vi "数据编码.vi"(0 "table输入":string(combo), 5 "错误常量 2":errorcluster caption="错误输入", 9 "QN":string, 13 "MN":string, 14 "PW":string) -> (4 "错误常量":errorcluster caption="错误输出", 15 "通讯包字符串":string)   [LabVIEW 2016, in "数据传输系统.lvlib"]
panel:
  in  "时间戳 2":string
  out "核查数据发送次数":i32
  out "小时数据发送次数":i32
  out "长度":i32
  in  "数据块":T1
  out "通讯包":T2={"包头（2）"="##", "数据段长度（4）"="", "数据段"="", "CRC校验"="", "包尾"=""}
  # "范例代码：\n\n##0101QN=20160801085857223;ST=32;CN=1062;PW=100000;MN=010000A8900016F000169DC0;Flag=5\n;CP=&&RtdInterval=30&&1C80\\r\\n"
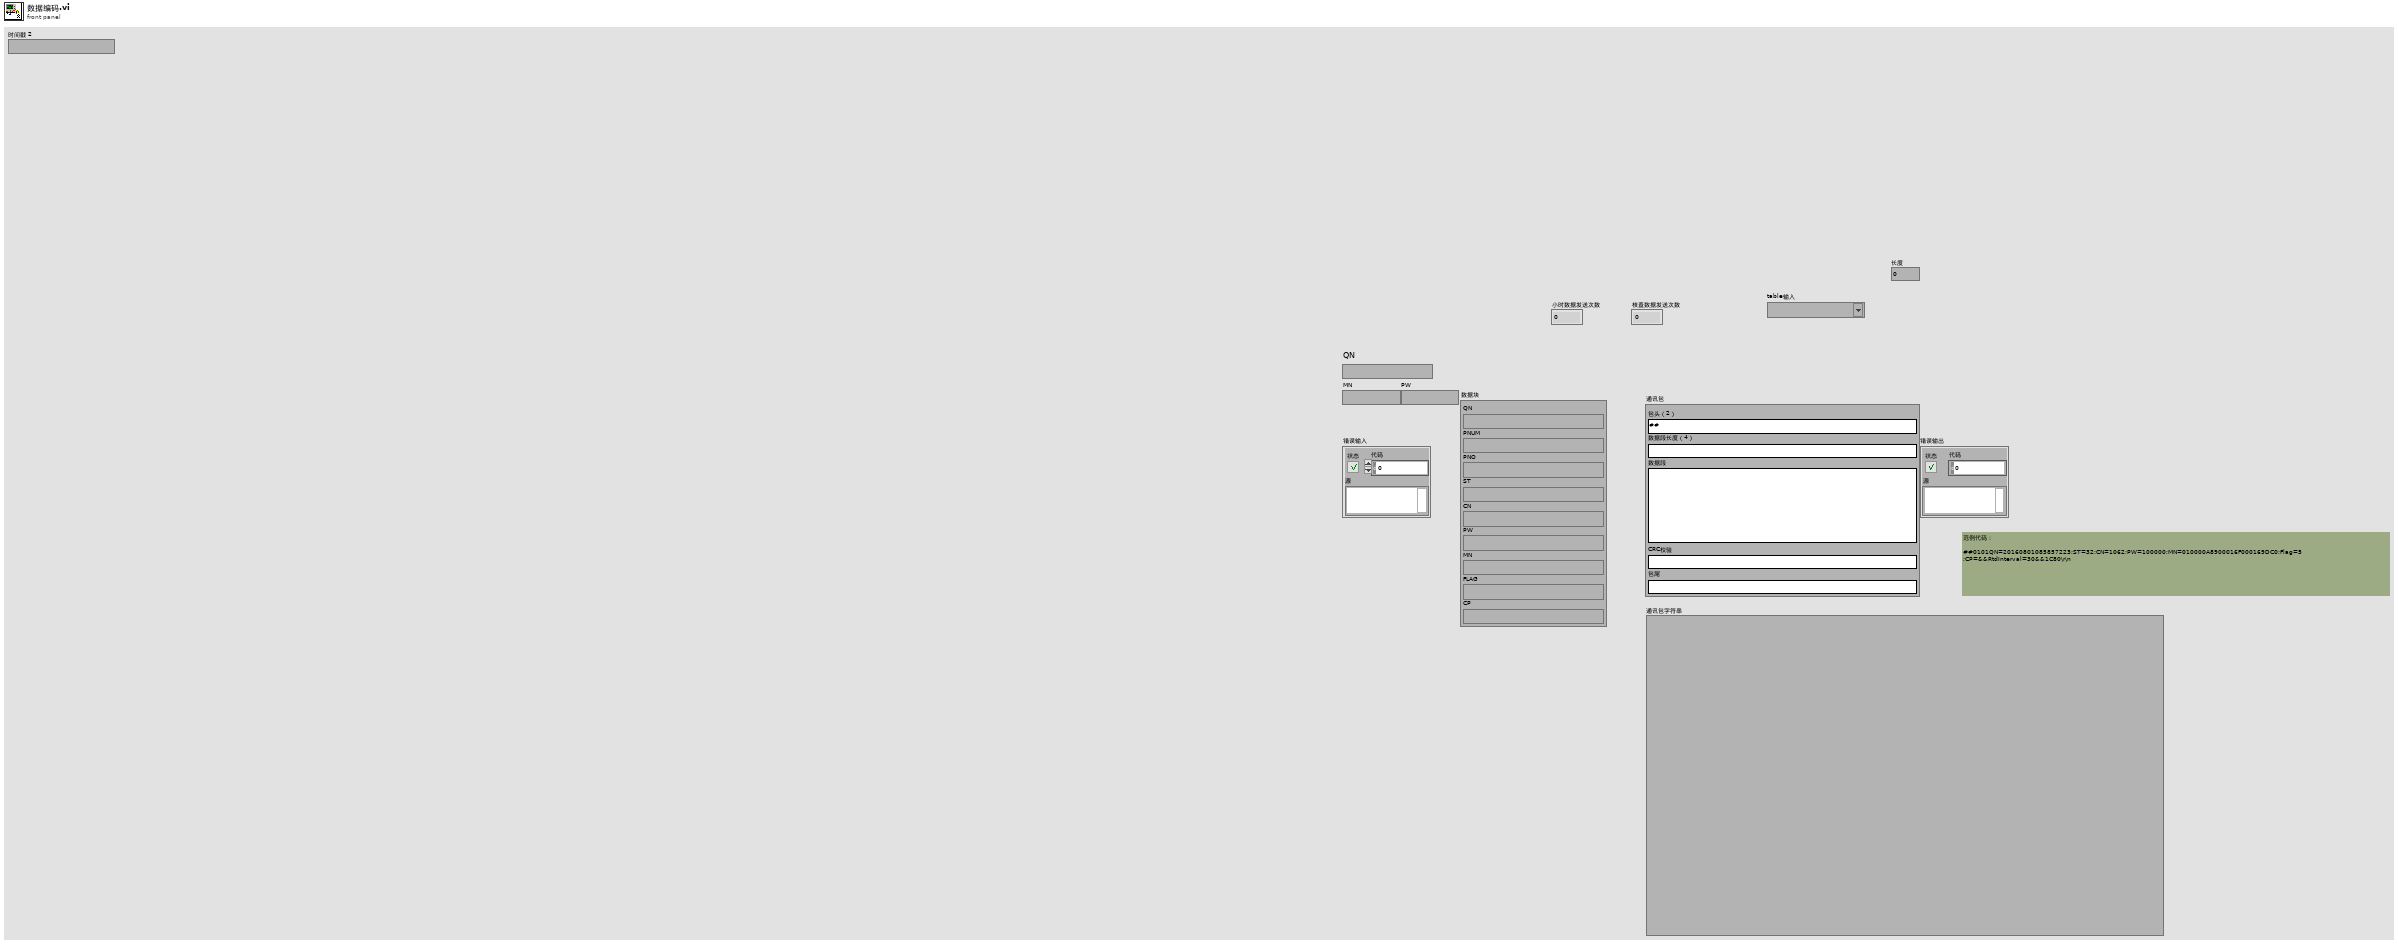
[diagram p1: front panel]
types:
  T1 = cluster{"QN":string, "ST":string, "CN":string, "PW":string, "MN":string, "FLAG":string, "PNUM":string, "PNO":string, "CP":string}
  T2 = cluster{"包头（2）":string, "数据段长度（4）":string, "数据段":string, "CRC校验":string, "包尾":string}
  T3 = cluster{"PH":string[][], "CODCr":string[][], "氨氮":string[][], "CODMn":string[][], "总氮":string[][], "总磷":string[][], "电导率":string[][], "水温":string[][], "DO":string[][], "浊度":string[][], "叶绿素":string[][], "藻密度":string[][], "铜":string[][], "盐度":string[][], "水位":string[][], "流速":string[][], "瞬时流量":string[][], "累积流量":string[][], "亚硝酸盐":string[][], "硫化物":string[][], "ORP":string[][], "铅":string[][], "镉":string[][], "锌":string[][], "镍":string[][], "锰":string[][], "汞":string[][]}
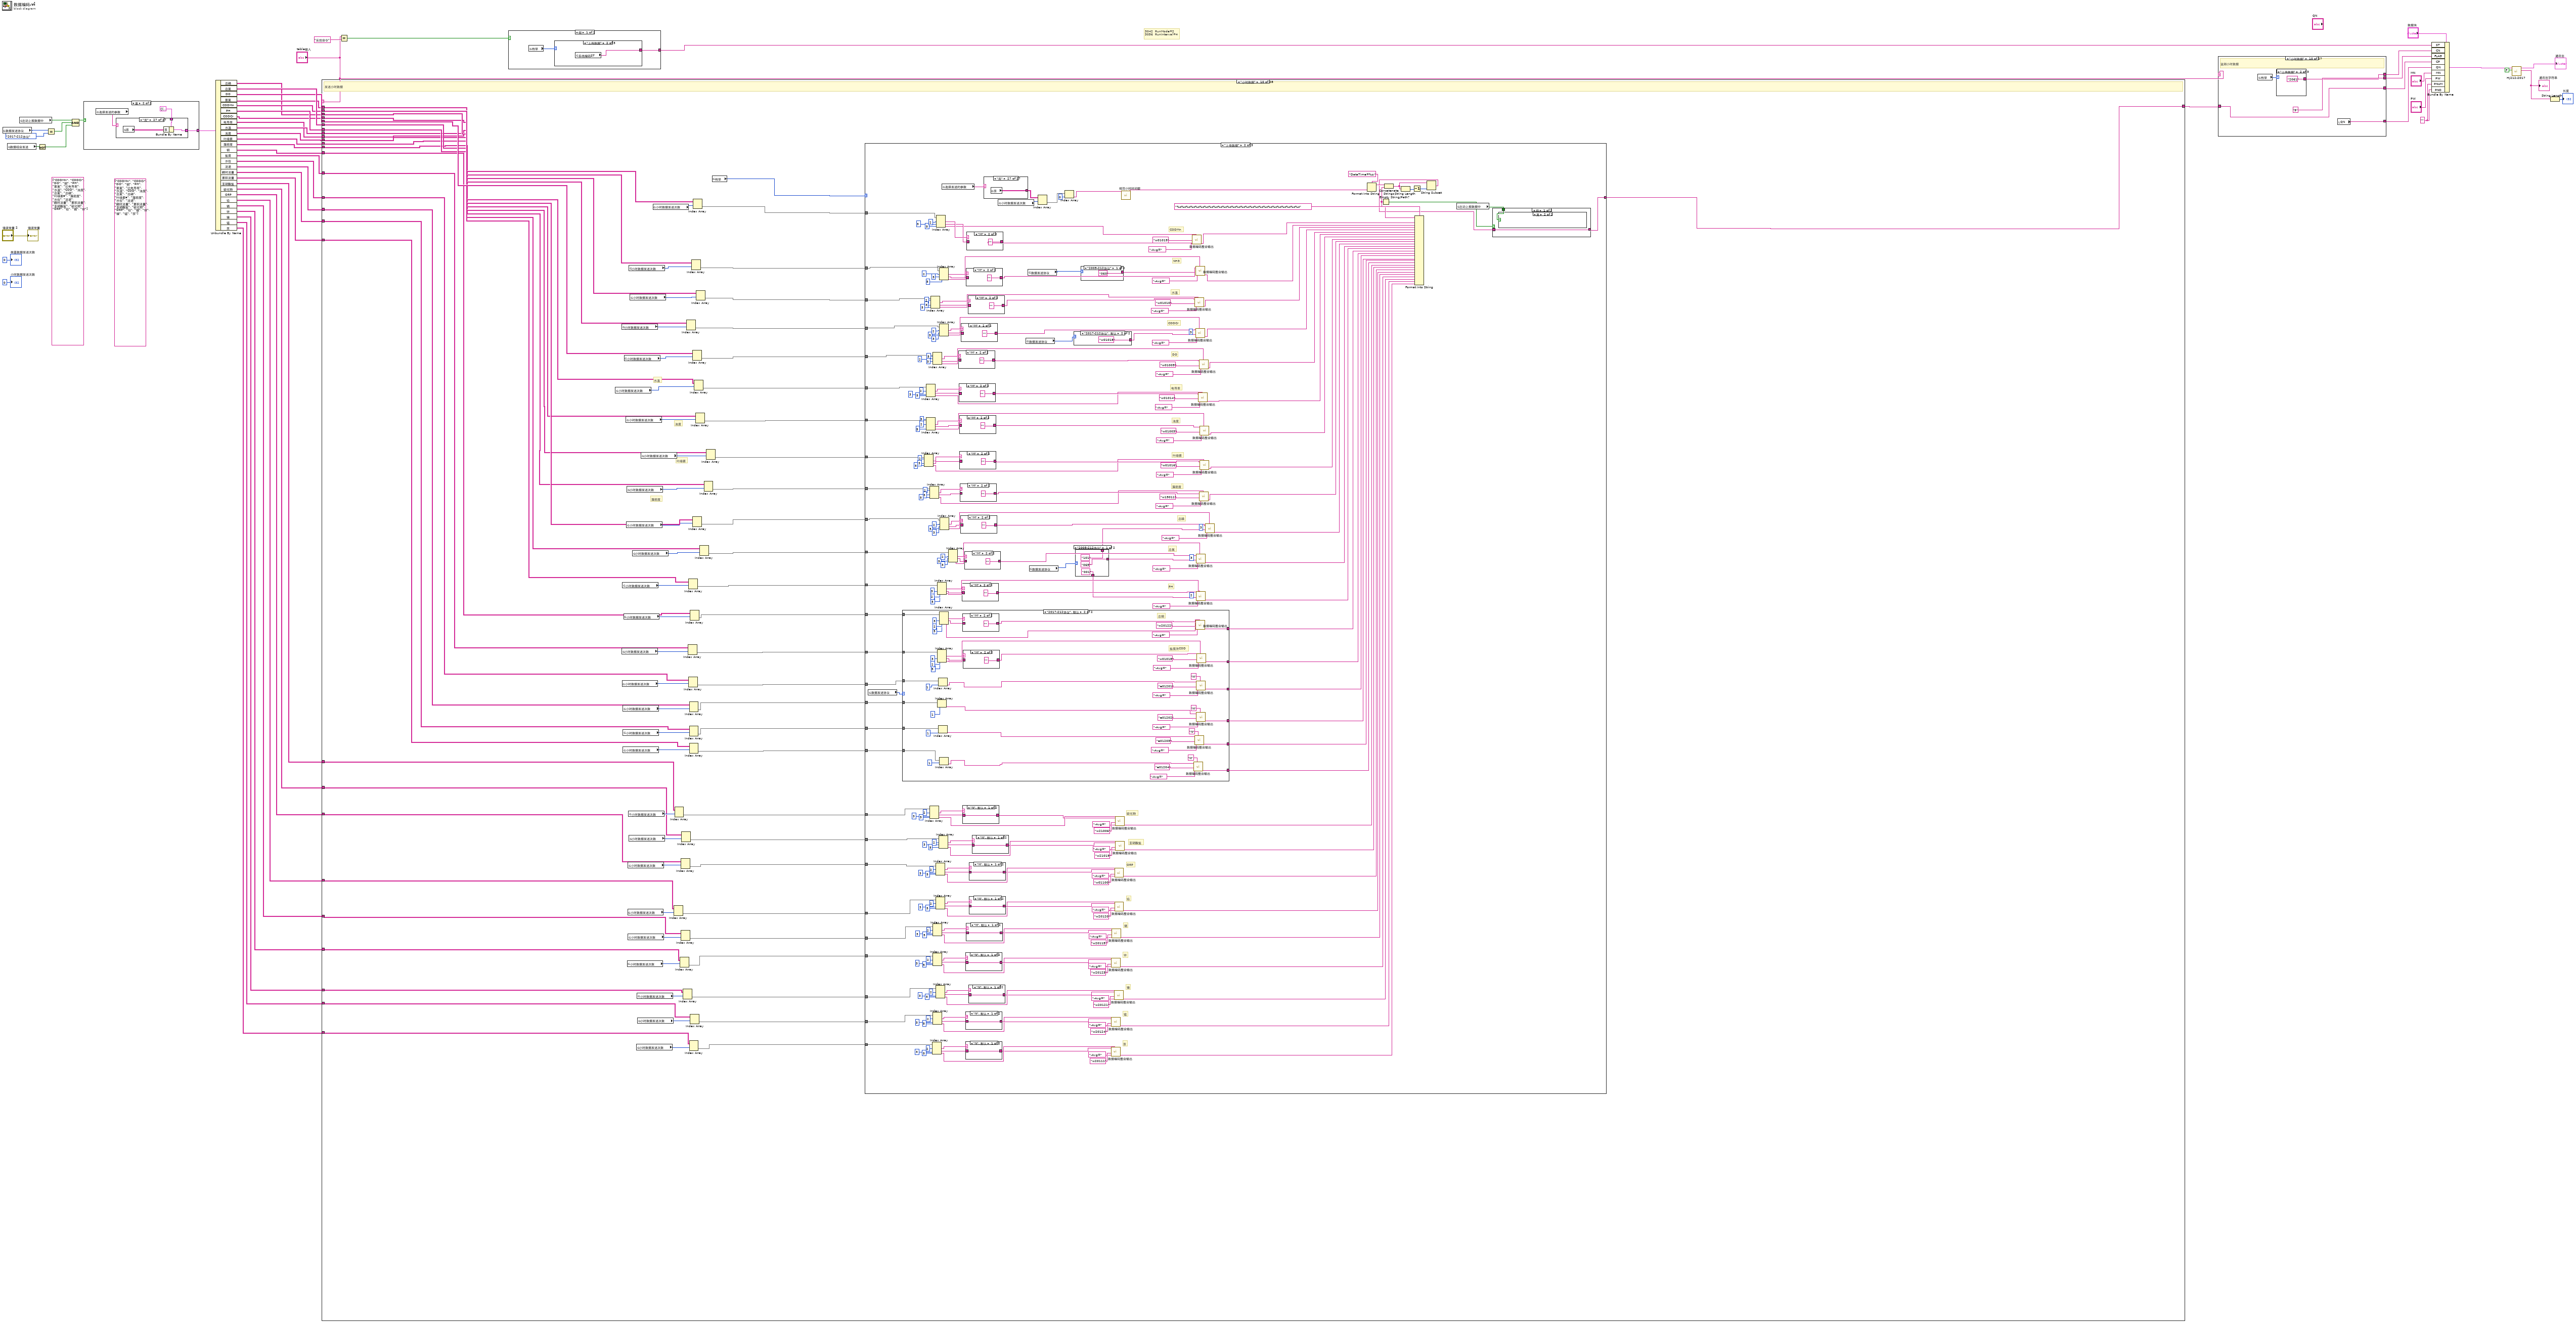
[diagram p0: block diagram]
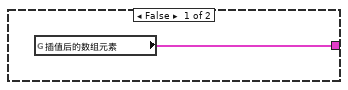
[diagram p2: hidden frame]
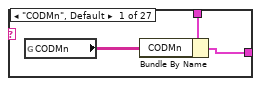
[diagram p3: hidden frame]
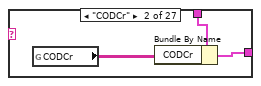
[diagram p4: hidden frame]
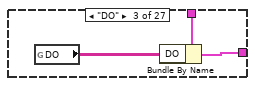
[diagram p5: hidden frame]
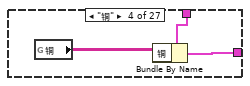
[diagram p6: hidden frame]
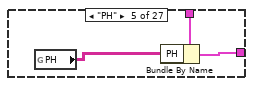
[diagram p7: hidden frame]
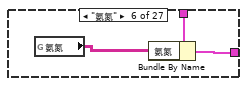
[diagram p8: hidden frame]
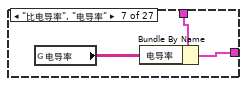
[diagram p9: hidden frame]
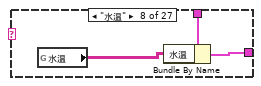
[diagram p10: hidden frame]
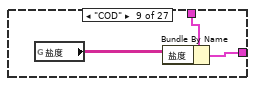
[diagram p11: hidden frame]
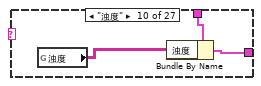
[diagram p12: hidden frame]
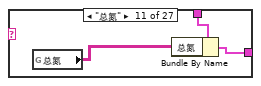
[diagram p13: hidden frame]
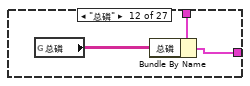
[diagram p14: hidden frame]
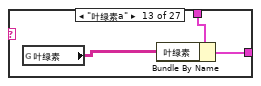
[diagram p15: hidden frame]
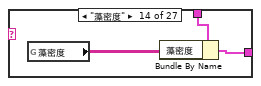
[diagram p16: hidden frame]
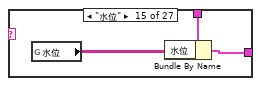
[diagram p17: hidden frame]
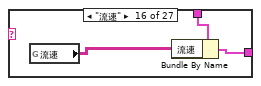
[diagram p18: hidden frame]
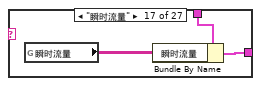
[diagram p19: hidden frame]
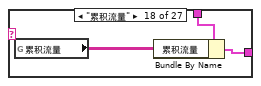
[diagram p20: hidden frame]
diagram:
  (unwired) string[] ["CODMn", "CODCr", "DO", "铜", "PH", "氨氮", "比电导率", "水温", "COD", "浊度", "总氮", "总磷", "叶绿素a", "藻密度", "水位", "流速", "瞬时流量", "累积流量", "亚硝酸盐", "硫化物", "ORP", "铅", "镉", "锌"] ("数组")
  (unwired) string[] ["CODMn", "CODCr", "DO", "铜", "PH", "氨氮", "比电导率", "水温", "COD", "浊度", "总氮", "总磷", "叶绿素a", "藻密度", "水位", "流速", "瞬时流量", "累积流量", "亚硝酸盐", "硫化物", "ORP", "铅", "镉", "锌", "镍", "锰", "汞"] ("数组")
  w40 = ""
  # "3042  RunMode=2\n3056  RunInterval=4"
  n1 = global read "断电保存全局.vi" "数据发送协议"() -> (w11:enum16{"2005-212协议", "2017-212协议"})
  n2 = global read "断电保存全局.vi" "数据组合发送"() -> (w13:bool)
  n3 = global read "全局 数据发送重叠.vi" "主动上报数据中"() -> (w26:bool)
  n4 = Not(x=w13) -> (.not. x?=w12:bool)
  n5 = Equal?(x=w11, y=enum16{"2005-212协议", "2017-212协议"}."2017-212协议" ("数据发送版本")) -> (x = y?=w16:bool)
  n6 = Compound Arithmetic op=AND ("复合运算")(w26, w16, w12) -> (w17:bool)
  n7 = case shown="真" w17 {
    tunnel: [w57 w59] -> w27
    frame False {
      n8 = global read "插值后的新数组.vi" "插值后的数组元素"() -> (w57:T3)
    }
    frame True {
      n9 = global read "全局 水样时间.vi" "选择发送的参数"() -> (w60:string)
      n10 = case shown="\"汞\"" w60 {
        tunnel: T3 {"PH"=[], "CODCr"=[], "氨氮"=[], "CODMn"=[], "总氮"=[], "总磷"=[], "电导率"=[], "水温"=[], "DO"=[], "浊度"=[], "叶绿素"=[], "藻密度"=[], "铜"=[], "盐度"=[], "水位"=[], "流速"=[], "瞬时流量"=[], "累积流量"=[], "亚硝酸盐"=[], "硫化物"=[], "ORP"=[], "铅"=[], "镉"=[], "锌"=[], "镍"=[], "锰"=[], "汞"=[]} ("插值后的数组元素") -> [w62 w66 w69 w72 w75 w78 w81 w84 w87 w90 w93 w96 w99 w101 w105 w108 w110 w113 w116 w119 w122 w125 w128 w131 w134 w137 w140]
        tunnel: [w61 w64 w67 w70 w73 w76 w80 w83 w85 w88 w91 w94 w97 w100 w103 w106 w109 w112 w115 w118 w121 w124 w127 w130 w133 w136 w139] -> w59
        frame "CODMn", Default {
          n11 = global read "全局 所有参数.vi" "CODMn"() -> (w63:string[][])
          n12 = Bundle By Name(cluster=w62, "CODMn"=w63) -> (w61:T3)
        }
        frame "CODCr" {
          n13 = global read "全局 所有参数.vi" "CODCr"() -> (w65:string[][])
          n14 = Bundle By Name(cluster=w66, "CODCr"=w65) -> (w64:T3)
        }
        frame "DO" {
          n15 = global read "全局 所有参数.vi" "DO"() -> (w68:string[][])
          n16 = Bundle By Name(cluster=w69, "DO"=w68) -> (w67:T3)
        }
        frame "铜" {
          n17 = global read "全局 所有参数.vi" "铜"() -> (w71:string[][])
          n18 = Bundle By Name(cluster=w72, "铜"=w71) -> (w70:T3)
        }
        frame "PH" {
          n19 = global read "全局 所有参数.vi" "PH"() -> (w74:string[][])
          n20 = Bundle By Name(cluster=w75, "PH"=w74) -> (w73:T3)
        }
        frame "氨氮" {
          n21 = global read "全局 所有参数.vi" "氨氮"() -> (w77:string[][])
          n22 = Bundle By Name(cluster=w78, "氨氮"=w77) -> (w76:T3)
        }
        frame "比电导率", "电导率" {
          n23 = global read "全局 所有参数.vi" "电导率"() -> (w79:string[][])
          n24 = Bundle By Name(cluster=w81, "电导率"=w79) -> (w80:T3)
        }
        frame "水温" {
          n25 = global read "全局 所有参数.vi" "水温"() -> (w82:string[][])
          n26 = Bundle By Name(cluster=w84, "水温"=w82) -> (w83:T3)
        }
        frame "COD" {
          n27 = global read "全局 所有参数.vi" "盐度"() -> (w86:string[][])
          n28 = Bundle By Name(cluster=w87, "盐度"=w86) -> (w85:T3)
        }
        frame "浊度" {
          n29 = global read "全局 所有参数.vi" "浊度"() -> (w89:string[][])
          n30 = Bundle By Name(cluster=w90, "浊度"=w89) -> (w88:T3)
        }
        frame "总氮" {
          n31 = global read "全局 所有参数.vi" "总氮"() -> (w92:string[][])
          n32 = Bundle By Name(cluster=w93, "总氮"=w92) -> (w91:T3)
        }
        frame "总磷" {
          n33 = global read "全局 所有参数.vi" "总磷"() -> (w95:string[][])
          n34 = Bundle By Name(cluster=w96, "总磷"=w95) -> (w94:T3)
        }
        frame "叶绿素a" {
          n35 = global read "全局 所有参数.vi" "叶绿素"() -> (w98:string[][])
          n36 = Bundle By Name(cluster=w99, "叶绿素"=w98) -> (w97:T3)
        }
        frame "藻密度" {
          n37 = global read "全局 所有参数.vi" "藻密度"() -> (w102:string[][])
          n38 = Bundle By Name(cluster=w101, "藻密度"=w102) -> (w100:T3)
        }
        frame "水位" {
          n39 = global read "全局 所有参数.vi" "水位"() -> (w104:string[][])
          n40 = Bundle By Name(cluster=w105, "水位"=w104) -> (w103:T3)
        }
        frame "流速" {
          n41 = global read "全局 所有参数.vi" "流速"() -> (w107:string[][])
          n42 = Bundle By Name(cluster=w108, "流速"=w107) -> (w106:T3)
        }
        frame "瞬时流量" {
          n43 = global read "全局 所有参数.vi" "瞬时流量"() -> (w111:string[][])
          n44 = Bundle By Name(cluster=w110, "瞬时流量"=w111) -> (w109:T3)
        }
        frame "累积流量" {
          n45 = global read "全局 所有参数.vi" "累积流量"() -> (w114:string[][])
          n46 = Bundle By Name(cluster=w113, "累积流量"=w114) -> (w112:T3)
        }
        frame "亚硝氮" {
          n47 = global read "全局 所有参数.vi" "亚硝酸盐"() -> (w117:string[][])
          n48 = Bundle By Name(cluster=w116, "亚硝酸盐"=w117) -> (w115:T3)
        }
        frame "硫化物" {
          n49 = global read "全局 所有参数.vi" "硫化物"() -> (w120:string[][])
          n50 = Bundle By Name(cluster=w119, "硫化物"=w120) -> (w118:T3)
        }
        frame "ORP" {
          n51 = global read "全局 所有参数.vi" "ORP"() -> (w123:string[][])
          n52 = Bundle By Name(cluster=w122, "ORP"=w123) -> (w121:T3)
        }
        frame "铅" {
          n53 = global read "全局 所有参数.vi" "铅"() -> (w126:string[][])
          n54 = Bundle By Name(cluster=w125, "铅"=w126) -> (w124:T3)
        }
        frame "镉" {
          n55 = global read "全局 所有参数.vi" "镉"() -> (w129:string[][])
          n56 = Bundle By Name(cluster=w128, "镉"=w129) -> (w127:T3)
        }
        frame "锌" {
          n57 = global read "全局 所有参数.vi" "锌"() -> (w132:string[][])
          n58 = Bundle By Name(cluster=w131, "锌"=w132) -> (w130:T3)
        }
        frame "镍" {
          n59 = global read "全局 所有参数.vi" "镍"() -> (w135:string[][])
          n60 = Bundle By Name(cluster=w134, "镍"=w135) -> (w133:T3)
        }
        frame "锰" {
          n61 = global read "全局 所有参数.vi" "锰"() -> (w138:string[][])
          n62 = Bundle By Name(cluster=w137, "锰"=w138) -> (w136:T3)
        }
        frame "汞" {
          n63 = global read "全局 所有参数.vi" "汞"() -> (w141:string[][])
          n64 = Bundle By Name(cluster=w140, "汞"=w141) -> (w139:T3)
        }
      }
    }
  }
  n65 = Unbundle By Name(w27) -> ("总磷"=w19:string[][], "总氮"=w24:string[][], "DO"=w23:string[][], "氨氮"=w22:string[][], "CODMn"=w20:string[][], "PH"=w39:string[][], "CODCr"=w21:string[][], "电导率"=w15:string[][], "水温"=w38:string[][], "浊度"=w14:string[][], "叶绿素"=w37:string[][], "藻密度"=w34:string[][], "铜"=w33:string[][], "盐度"=w32:string[][], "水位"=w31:string[][], "流速"=w30:string[][], "瞬时流量"=w29:string[][], "累积流量"=w28:string[][], "亚硝酸盐"=w10:string[][], "硫化物"=w9:string[][], "ORP"=w8:string[][], "铅"=w6:string[][], "镉"=w5:string[][], "锌"=w4:string[][], "镍"=w3:string[][], "锰"=w2:string[][], "汞"=w1:string[][])
  n66 = case shown="\"小时数据\"" "table输入" {
    tunnel: [w143 w150 w164 w207 w230 _ w244 w253 w289 w1334 w1759 w1806 w1895 w2046 w2218 w2451 w2518 w2564 w2612 w2684 w2812 w2926 w3040 w3133 w3587 w3623 w3634 w3645] -> w35
    tunnel: w20 -> [_ _ _ _ _ _ _ _ w287 w1333 _ _ w1894 w2058 w2222 w2455 w2522 w2563 w2611 w2683 w2811 w2925 w3039 w3132 _ _ _ _]
    tunnel: w22 -> [_ _ _ _ _ _ _ _ w286 w1332 _ _ w1893 w2057 w2221 w2454 w2523 w2562 w2610 w2682 w2810 w2924 w3038 w3131 _ _ _ _]
    tunnel: w23 -> [_ _ _ _ _ _ _ _ w283 w1331 _ _ w1892 w2056 w2200 _ _ _ w2606 w2681 w2809 w2923 w3037 w3111 _ _ _ _]
    tunnel: w19 -> [_ _ _ _ _ _ _ _ w278 w1330 _ _ w1891 w2055 w2220 w2453 w2521 w2561 w2607 w2680 w2808 w2922 w3036 w3130 _ _ _ _]
    tunnel: w24 -> [_ _ _ _ _ _ _ _ w277 w1329 _ _ w1890 w2054 w2219 w2452 w2520 w2559 w2609 w2679 w2807 w2921 w3035 w3129 _ _ _ _]
    tunnel: w39 -> [_ _ _ _ _ _ _ _ w284 w1328 _ _ w1889 w2053 w2204 _ _ _ w2605 _ w2791 w2905 w3013 w3109 _ _ _ _]
    tunnel: w21 -> [_ _ _ _ _ _ _ _ w270 w1327 _ _ w1888 w2052 w2217 w2450 w2519 w2560 w2608 w2666 w2795 w2909 w3023 w3116 _ _ _ _]
    tunnel: w15 -> [_ _ _ _ _ _ _ _ w282 w1326 _ _ w1887 w2051 w2197 _ _ _ w2603 _ w2788 w2902 w3011 w3106 _ _ _ _]
    tunnel: w38 -> [_ _ _ _ _ _ _ _ w285 w1325 _ _ w1886 w2050 _ _ _ _ w2604 _ w2785 w2899 w3012 w3101 _ _ _ _]
    tunnel: w14 -> [_ _ _ _ _ _ _ _ w281 w1324 _ _ w1885 w2049 w2194 _ _ _ w2602 _ w2779 w2893 w3007 w3100 _ _ _ _]
    tunnel: w37 -> [_ _ _ _ _ _ _ _ w280 w1323 _ _ w1884 w2048 _ _ _ _ _ _ w2777 w2891 w3005 w3099 _ _ _ _]
    tunnel: w34 -> [_ _ _ _ _ _ _ _ w279 w1322 _ _ w1883 w2047 _ _ _ _ _ _ w2775 w2889 w3004 w3114 _ _ _ _]
    tunnel: w33 -> [_ _ _ _ _ _ _ _ w276 w1292 _ _ w1853 w2018 _ _ _ _ _ _ _ _ _ _ _ _ _ _]
    tunnel: w32 -> [_ _ _ _ _ _ _ _ w275 w1291 _ _ w1852 w2017 _ _ _ _ _ _ _ _ _ _ _ _ _ _]
    tunnel: w31 -> [_ _ _ _ _ _ _ _ w273 w1282 _ _ _ _ _ _ _ _ _ _ _ _ _ _ _ _ _ _]
    tunnel: w30 -> [_ _ _ _ _ _ _ _ w274 w1281 _ _ _ _ _ _ _ _ _ _ _ _ _ _ _ _ _ _]
    tunnel: w29 -> [_ _ _ _ _ _ _ _ w272 w1280 _ _ _ _ _ _ _ _ _ _ _ _ _ _ _ _ _ _]
    tunnel: w28 -> [_ _ _ _ _ _ _ _ w271 w1279 _ _ _ _ _ _ _ _ _ _ _ _ _ _ _ _ _ _]
    tunnel: w10 -> [_ _ _ _ _ _ _ _ w269 w1275 _ _ _ _ _ _ _ _ _ _ _ _ _ _ _ _ _ _]
    tunnel: w9 -> [_ _ _ _ _ _ _ _ w268 w1274 _ _ _ _ _ _ _ _ _ _ _ _ _ _ _ _ _ _]
    tunnel: w8 -> [_ _ _ _ _ _ _ _ w267 w1273 _ _ _ _ _ _ _ _ _ _ w2773 w2887 w3003 _ _ _ _ _]
    tunnel: w6 -> [_ _ _ _ _ _ _ _ w266 w1266 _ _ _ _ _ _ _ _ _ _ _ _ _ _ _ _ _ _]
    tunnel: w5 -> [_ _ _ _ _ _ _ _ w265 w1265 _ _ _ _ _ _ _ _ _ _ _ _ _ _ _ _ _ _]
    tunnel: w4 -> [_ _ _ _ _ _ _ _ w264 w1264 _ _ _ _ _ _ _ _ _ _ _ _ _ _ _ _ _ _]
    tunnel: w3 -> [_ _ _ _ _ _ _ _ w263 w1257 _ _ _ _ _ _ _ _ _ _ _ _ _ _ _ _ _ _]
    tunnel: w2 -> [_ _ _ _ _ _ _ _ w262 w1256 _ _ _ _ _ _ _ _ _ _ _ _ _ _ _ _ _ _]
    tunnel: w1 -> [_ _ _ _ _ _ _ _ w261 w1255 _ _ _ _ _ _ _ _ _ _ _ _ _ _ _ _ _ _]
    frame "反控命令" {
      n67 = global read "全局 反控命令枚举.vi" "反控命令枚举"() -> (w142:enum16{"返回请求应答", "返回执行结果"})
      n68 = case shown="\"返回执行结果\"" w142 {
        tunnel: ["QnRtn=1" w146] -> w143
        frame "返回请求应答", Default {
        }
        frame "返回执行结果" {
          n69 = global read "全局 反控命令枚举.vi" "执行结果定义"() -> (w147:u16)
          n70 = Number To Decimal String(number=w147) -> (decimal integer string=w145:string)  [unwired: 1 in]
          n71 = Concatenate Strings("ExeRtn=", w145) -> (w146:string)
        }
      }
    }
    frame "超标留样返回" {
      n72 = global read "全局1.vi" "枚举"() -> (w149:enum16{"返回请求应答", "上传数据", "返回执行结果"})
      n73 = case shown="\"返回请求应答\", 默认" w149 {
        tunnel: ["QnRtn=1" w152 "ExeRtn=1"] -> w150
        frame "返回请求应答", Default {
        }
        frame "上传数据" {
          n74 = global read "全局1.vi" "register values"() -> (w161:u16[])
          n75 = Index Array(array=w161, index=7 ("索引")) -> (element=w154:u16)
          n76 = Get Date/Time In Seconds() -> (seconds since 1Jan1904=w159:timestamp)
          n77 = Number To Decimal String(number=w154) -> (decimal integer string=w155:string)  [unwired: 1 in]
          n78 = Format Date/Time String(time format string (%c)="%Y%m%d%H%M%S" ("时间格式字符串(%c)"), seconds (now)=w159) -> (date/time string=w157:string)  [unwired: 1 in]
          n79 = Format Into String(format string="VaseNo=%s" ("格式字符串"), w155) -> (resulting string=w153:string)  [unwired: 2 in, 1 out]
          n80 = Format Into String(format string="DataTime=%s;%s" ("格式字符串"), w157, w153) -> (resulting string=w152:string)  [unwired: 2 in, 1 out]
        }
        frame "返回执行结果" {
        }
      }
    }
    frame "提取经纬度环境信息" {
      # "BDS纬度"
      # "BDS纬度"
      # "GPS纬度"
      # "GPS经度"
      # "湿度"
      # "温度"
      # "电压"
      # "时间"
      n81 = global read "全局1.vi" "枚举"() -> (w165:enum16{"返回请求应答", "上传数据", "返回执行结果"})
      n82 = case shown="\"上传数据\"" w165 {
        tunnel: ["QnRtn=1" w178 "ExeRtn=1"] -> w164
        frame "返回请求应答", Default {
        }
        frame "上传数据" {
          n83 = global read "全局 环境参数.vi" "columns输出"() -> (w175:string[])
          n84 = Array Subset(array=w175, index=1 ("索引")) -> (w176:string[])  [unwired: 1 in]
          n85 = for {
            tunnel: w176 -> [w184] mode=indexing
            tunnel: [w183] -> w177 mode=indexing
            n86 = case shown="\"BDS经度\"" w184 {
              tunnel: ["" "Volt=%s;" "Temp=%s;" ("格式字符串") "Hum=%s;" ("格式字符串") "Lng=%s;" "Lat=%s;" "Lng2=%s;" "Lat2=%s;"] -> w183
              frame "假", Default {
              }
              frame "电压" {
              }
              frame "室温" {
              }
              frame "湿度" {
              }
              frame "GPS经度" {
              }
              frame "GPS纬度" {
              }
              frame "BDS经度" {
              }
              frame "BDS纬度" {
              }
            }
          }
          n87 = global read "全局 环境参数.vi" "环境参数"() -> (w168:string[][])
          n88 = Index Array(array=w168, index (row)=0 ("索引 (行)")) -> (element=w171:string[])  [unwired: 1 in]
          n89 = Array Subset(array=w171, index=1 ("索引")) -> (w173:string[])  [unwired: 1 in]
          n90 = for {
            shift-right: [w198] -> w167
            shift-left: "" -> [w197]
            tunnel: w177 -> [w196] mode=indexing
            tunnel: w173 -> [w194] mode=indexing
            n91 = Fract/Exp String To Number(string=w194) -> (number=w195:dbl)  [unwired: 3 in, 1 out]
            n92 = Empty String/Path?(string/path=w194) -> (empty?=w200:bool)
            n93 = Number To Fractional String(number=w195) -> (F-format string=w193:string)  [unwired: 3 in]
            n94 = case shown="假" w200 {
              tunnel: [w203 w204] -> w199
              tunnel: w196 -> [w202 _]
              tunnel: w193 -> [w201 _]
              tunnel: w193 -> [_ w204]
              frame False {
                n95 = Format Into String(format string=w202, w201) -> (resulting string=w203:string)  [unwired: 2 in, 1 out]
              }
              frame True {
              }
            }
            n96 = Concatenate Strings(w197, w199) -> (w198:string)
          }
          n97 = Get Date/Time In Seconds() -> (seconds since 1Jan1904=w180:timestamp)
          n98 = Format Date/Time String(time format string (%c)="%Y%m%d%H%M%S" ("时间格式字符串(%c)"), seconds (now)=w180) -> (date/time string=w179:string)  [unwired: 1 in]
          n99 = Format Into String(format string="DataTime=%s;%s" ("格式字符串"), w179, w167) -> (resulting string=w178:string)  [unwired: 2 in, 1 out]
        }
        frame "返回执行结果" {
        }
      }
    }
    frame "提取现场系统信息" {
      n100 = global read "全局1.vi" "枚举"() -> (w206:enum16{"返回请求应答", "上传数据", "返回执行结果"})
      n101 = case shown="\"上传数据\"" w206 {
        tunnel: ["QnRtn=1" w227 "ExeRtn=1"] -> w207
        frame "返回请求应答", Default {
        }
        frame "上传数据" {
          n102 = global read "全局1.vi" "register values"() -> (w226:u16[])
          n103 = Get Date/Time In Seconds() -> (seconds since 1Jan1904=w212:timestamp)
          n104 = Index Array(array=w226, index #1=0 ("索引"), index #2=6 ("索引")) -> (element #1=w222:u16, element #2=w209:u16)
          n105 = Format Date/Time String(time format string (%c)="%Y%m%d%H%M%S%u" ("时间格式字符串(%c)"), seconds (now)=w212) -> (date/time string=w215:string)  [unwired: 1 in]
          n106 = Number To Decimal String(number=w222) -> (decimal integer string=w224:string)  [unwired: 1 in]
          n107 = Number To Decimal String(number=w209) -> (decimal integer string=w218:string)  [unwired: 1 in]
          n108 = Search and Replace String(input string=w215, search string="." ("搜索字符串")) -> (result string=w211:string)  [unwired: 6 in, 3 out]
          n109 = Format Into String(format string="RunMode=%s;" ("格式字符串"), w224) -> (resulting string=w221:string)  [unwired: 2 in, 1 out]
          n110 = Format Into String(format string="RunInterval=%s;" ("格式字符串"), w218) -> (resulting string=w219:string)  [unwired: 2 in, 1 out]
          n111 = Format Into String(format string="SystemTime=%s;" ("格式字符串"), w211) -> (resulting string=w216:string)  [unwired: 2 in, 1 out]
          n112 = Concatenate Strings(w221, w219, w216) -> (w227:string)
        }
        frame "返回执行结果" {
        }
      }
    }
    frame "提取监测仪表时间" {
      n113 = global read "全局1.vi" "枚举"() -> (w229:enum16{"返回请求应答", "上传数据", "返回执行结果"})
      n114 = case shown="\"上传数据\"" w229 {
        tunnel: ["QnRtn=1" w242 "ExeRtn=1"] -> w230
        frame "返回请求应答", Default {
        }
        frame "上传数据" {
          n115 = global read "全局 提取仪器参数.vi" "仪器编码"() -> (w232:string)
          n116 = Get Date/Time In Seconds() -> (seconds since 1Jan1904=w235:timestamp)
          n117 = Format Date/Time String(time format string (%c)="%Y%m%d%H%M%S%u" ("时间格式字符串(%c)"), seconds (now)=w235) -> (date/time string=w238:string)  [unwired: 1 in]
          n118 = Search and Replace String(input string=w238, search string="." ("搜索字符串")) -> (result string=w234:string)  [unwired: 6 in, 3 out]
          n119 = Format Into String(format string="PolId=%s;" ("格式字符串"), w232) -> (resulting string=w240:string)  [unwired: 2 in, 1 out]
          n120 = Format Into String(format string="SystemTime=%s;" ("格式字符串"), w234) -> (resulting string=w233:string)  [unwired: 2 in, 1 out]
          n121 = Concatenate Strings(w240, w233) -> (w242:string)
        }
        frame "返回执行结果" {
        }
      }
    }
    frame "心跳包", Default {
    }
    frame "提取数采仪时间" {
      (unwired) ""
      n122 = global read "全局1.vi" "枚举"() -> (w245:enum16{"返回请求应答", "上传数据", "返回执行结果"})
      n123 = case shown="\"上传数据\"" w245 {
        tunnel: ["QnRtn=1" w247 "ExeRtn=1"] -> w244
        frame "返回请求应答", Default {
        }
        frame "上传数据" {
          n124 = Get Date/Time In Seconds() -> (seconds since 1Jan1904=w251:timestamp)
          n125 = Format Date/Time String(time format string (%c)="%Y%m%d%H%M%S" ("时间格式字符串(%c)"), seconds (now)=w251) -> (date/time string=w248:string)  [unwired: 1 in]
          n126 = Concatenate Strings("SystemTime=", w248) -> (w247:string)
        }
        frame "返回执行结果" {
        }
      }
    }
    frame "提取实时数据间隔" {
      (unwired) ""
      n127 = global read "全局1.vi" "枚举"() -> (w254:enum16{"返回请求应答", "上传数据", "返回执行结果"})
      n128 = case shown="\"上传数据\"" w254 {
        tunnel: ["QnRtn=1" w258 "ExeRtn=1"] -> w253
        frame "返回请求应答", Default {
        }
        frame "上传数据" {
          n129 = global read "实时数据发送间隔全局.vi" "实时数据发送间隔"() -> (w257:u32)
          n130 = Number To Decimal String(number=w257) -> (decimal integer string=w256:string)  [unwired: 1 in]
          n131 = Concatenate Strings("RtdInterval=", w256) -> (w258:string)
        }
        frame "返回执行结果" {
        }
      }
    }
    frame "实时数据" {
      # "包含质控数据主动上传"
      n132 = global read "全局 实时数据参数.vi" "实时数据参数"() -> (w288:string)
      n133 = case shown="\"水样测试\", 默认" w288 {
        tunnel: [w317 w695 w746 w825 w1087 w1156] -> w289
        tunnel: w287 -> [w316 w694 w745 w812 w1085 w1154]
        tunnel: w286 -> [w315 w693 w744 w813 w1084 w1153]
        tunnel: w285 -> [w314 w692 w743 w814 _ _]
        tunnel: w284 -> [w313 w691 w742 w815 w1080 _]
        tunnel: w283 -> [w312 w690 w741 w816 w1079 _]
        tunnel: w282 -> [w311 w689 w740 w817 w1078 _]
        tunnel: w281 -> [w310 w688 w739 w818 w1077 _]
        tunnel: w280 -> [w309 w687 w738 w819 w1076 _]
        tunnel: w279 -> [w308 w686 w737 w820 w1075 _]
        tunnel: w278 -> [w307 w685 w736 w821 w1083 w1152]
        tunnel: w277 -> [w306 w684 w735 w822 w1082 w1151]
        tunnel: w270 -> [w305 w683 w734 w823 w1081 w1150]
        tunnel: w276 -> [w304 w682 w733 w811 _ _]
        tunnel: w275 -> [w303 w681 w732 w810 _ _]
        tunnel: w273 -> [w302 _ _ _ _ _]
        tunnel: w272 -> [w301 _ _ _ _ _]
        tunnel: w271 -> [w300 _ _ _ _ _]
        tunnel: w274 -> [w299 _ _ _ _ _]
        tunnel: w269 -> [w298 _ w731 _ w1072 w1149]
        tunnel: w268 -> [w297 _ w730 _ w1073 w1148]
        tunnel: w267 -> [w296 _ w729 _ w1074 w1147]
        tunnel: w266 -> [w295 _ _ _ _ _]
        tunnel: w265 -> [w294 _ _ _ _ _]
        tunnel: w264 -> [w293 _ _ _ _ _]
        tunnel: w263 -> [w292 _ _ _ _ _]
        tunnel: w262 -> [w291 _ _ _ _ _]
        tunnel: w261 -> [w290 _ _ _ _ _]
        frame "水样测试", Default {
          n134 = global read "全局1.vi" "枚举"() -> (w318:enum16{"返回请求应答", "上传数据", "返回执行结果"})
          n135 = case shown="\"上传数据\"" w318 {
            tunnel: ["QnRtn=1" w553 "ExeRtn=1"] -> w317
            tunnel: w316 -> [_ w565 _]
            tunnel: w315 -> [_ w564 _]
            tunnel: w314 -> [_ w563 _]
            tunnel: w313 -> [_ w562 _]
            tunnel: w312 -> [_ w561 _]
            tunnel: w311 -> [_ w560 _]
            tunnel: w310 -> [_ w559 _]
            tunnel: w309 -> [_ w558 _]
            tunnel: w308 -> [_ w557 _]
            tunnel: w307 -> [_ w556 _]
            tunnel: w306 -> [_ w555 _]
            tunnel: w305 -> [_ w554 _]
            tunnel: w304 -> [_ w512 _]
            tunnel: w303 -> [_ w511 _]
            tunnel: w302 -> [_ w508 _]
            tunnel: w299 -> [_ w507 _]
            tunnel: w301 -> [_ w506 _]
            tunnel: w300 -> [_ w438 _]
            tunnel: w298 -> [_ w445 _]
            tunnel: w297 -> [_ w444 _]
            tunnel: w296 -> [_ w443 _]
            tunnel: w295 -> [_ w358 _]
            tunnel: w294 -> [_ w357 _]
            tunnel: w293 -> [_ w356 _]
            tunnel: w292 -> [_ w325 _]
            tunnel: w291 -> [_ w324 _]
            tunnel: w290 -> [_ w323 _]
            frame "返回请求应答", Default {
            }
            frame "上传数据" {
              # "汞"
              # "锰"
              # "镍"
              # "锌"
              # "镉"
              # "铅"
              # "藻密度"
              # "叶绿素a"
              # "浊度"
              # "电导率"
              # "DO"
              # "水温"
              # "CODMn"
              # "ORP"
              # "硫化物"
              # "亚硝酸盐"
              # "CODCr"
              # "总氮"
              # "总磷"
              # "PH"
              # "NH3"
              n136 = global read "断电保存全局.vi" "数据发送协议"() -> (w474:enum16{"2005-212协议", "2017-212协议"})
              n137 = global read "断电保存全局.vi" "数据发送协议"() -> (w478:enum16{"2005-212协议", "2017-212协议"})
              n138 = global read "断电保存全局.vi" "数据发送协议"() -> (w473:enum16{"2005-212协议", "2017-212协议"})
              n139 = global read "断电保存全局.vi" "数据发送协议"() -> (w476:enum16{"2005-212协议", "2017-212协议"})
              n140 = global read "断电保存全局.vi" "数据发送协议"() -> (w477:enum16{"2005-212协议", "2017-212协议"})
              n141 = global read "断电保存全局.vi" "数据发送协议"() -> (w475:enum16{"2005-212协议", "2017-212协议"})
              n142 = case shown="\"2017-212协议\", 默认" w473 {
                tunnel: ["060" ("污染物编码") "w21003" ("污染物编码")] -> w549
                frame "2005-212协议" {
                }
                frame "2017-212协议", Default {
                }
              }
              n143 = case shown="\"2005-212协议\"" w474 {
                tunnel: ["001" ("污染物编码") "w01001" ("污染物编码")] -> w542
                frame "2005-212协议" {
                }
                frame "2017-212协议", Default {
                }
              }
              n144 = global read "全局 水样时间.vi" "选择发送的参数"() -> (w492:string)
              n145 = case shown="\"2005-212协议\"" w476 {
                tunnel: ["065" ("污染物编码") "w21001" ("污染物编码")] -> w527
                frame "2005-212协议" {
                }
                frame "2017-212协议", Default {
                }
              }
              n146 = case shown="\"2017-212协议\", 默认" w475 {
                tunnel: ["011" ("污染物编码") "w01018" ("污染物编码")] -> w521
                frame "2005-212协议" {
                }
                frame "2017-212协议", Default {
                }
              }
              n147 = case shown="\"2005-212协议\"" w477 {
                tunnel: ["101" ("污染物编码") "w21011" ("污染物编码")] -> w531
                frame "2005-212协议" {
                }
                frame "2017-212协议", Default {
                }
              }
              n148 = case shown="\"汞\"" w492 {
                tunnel: [w647 w648 w649 w650 w651 w652 w653 w654 w655 w656 w657 w658 w659 w660 w661 w662 w663 w664 w665 w666 w667 w668 w669 w670 w671 w672 w673] -> w490
                frame "CODMn", Default {
                  n149 = global read "全局 所有参数.vi" "CODMn"() -> (w647:string[][])
                }
                frame "CODCr" {
                  n150 = global read "全局 所有参数.vi" "CODCr"() -> (w648:string[][])
                }
                frame "DO" {
                  n151 = global read "全局 所有参数.vi" "DO"() -> (w649:string[][])
                }
                frame "铜" {
                  n152 = global read "全局 所有参数.vi" "铜"() -> (w650:string[][])
                }
                frame "PH" {
                  n153 = global read "全局 所有参数.vi" "PH"() -> (w651:string[][])
                }
                frame "氨氮" {
                  n154 = global read "全局 所有参数.vi" "氨氮"() -> (w652:string[][])
                }
                frame "比电导率", "电导率" {
                  n155 = global read "全局 所有参数.vi" "电导率"() -> (w653:string[][])
                }
                frame "水温" {
                  n156 = global read "全局 所有参数.vi" "水温"() -> (w654:string[][])
                }
                frame "COD" {
                  n157 = global read "全局 所有参数.vi" "盐度"() -> (w655:string[][])
                }
                frame "浊度" {
                  n158 = global read "全局 所有参数.vi" "浊度"() -> (w656:string[][])
                }
                frame "总氮" {
                  n159 = global read "全局 所有参数.vi" "总氮"() -> (w657:string[][])
                }
                frame "总磷" {
                  n160 = global read "全局 所有参数.vi" "总磷"() -> (w658:string[][])
                }
                frame "叶绿素a" {
                  n161 = global read "全局 所有参数.vi" "叶绿素"() -> (w659:string[][])
                }
                frame "藻密度" {
                  n162 = global read "全局 所有参数.vi" "藻密度"() -> (w660:string[][])
                }
                frame "水位" {
                  n163 = global read "全局 所有参数.vi" "水位"() -> (w661:string[][])
                }
                frame "流速" {
                  n164 = global read "全局 所有参数.vi" "流速"() -> (w662:string[][])
                }
                frame "瞬时流量" {
                  n165 = global read "全局 所有参数.vi" "瞬时流量"() -> (w663:string[][])
                }
                frame "累积流量" {
                  n166 = global read "全局 所有参数.vi" "累积流量"() -> (w664:string[][])
                }
                frame "亚硝氮" {
                  n167 = global read "全局 所有参数.vi" "亚硝酸盐"() -> (w665:string[][])
                }
                frame "硫化物" {
                  n168 = global read "全局 所有参数.vi" "硫化物"() -> (w666:string[][])
                }
                frame "ORP" {
                  n169 = global read "全局 所有参数.vi" "ORP"() -> (w667:string[][])
                }
                frame "铅" {
                  n170 = global read "全局 所有参数.vi" "铅"() -> (w668:string[][])
                }
                frame "镉" {
                  n171 = global read "全局 所有参数.vi" "镉"() -> (w669:string[][])
                }
                frame "锌" {
                  n172 = global read "全局 所有参数.vi" "锌"() -> (w670:string[][])
                }
                frame "镍" {
                  n173 = global read "全局 所有参数.vi" "镍"() -> (w671:string[][])
                }
                frame "锰" {
                  n174 = global read "全局 所有参数.vi" "锰"() -> (w672:string[][])
                }
                frame "汞" {
                  n175 = global read "全局 所有参数.vi" "汞"() -> (w673:string[][])
                }
              }
              n176 = global read "全局 小时数据发送次数.vi" "小时数据发送次数"() -> (w431:i32)
              n177 = global read "全局 小时数据发送次数.vi" "小时数据发送次数"() -> (w395:i32)
              n178 = global read "全局 小时数据发送次数.vi" "小时数据发送次数"() -> (w516:i32)
              n179 = global read "全局 小时数据发送次数.vi" "小时数据发送次数"() -> (w515:i32)
              n180 = global read "全局 小时数据发送次数.vi" "小时数据发送次数"() -> (w423:i32)
              n181 = global read "全局 小时数据发送次数.vi" "小时数据发送次数"() -> (w491:i32)
              n182 = global read "全局 小时数据发送次数.vi" "小时数据发送次数"() -> (w396:i32)
              n183 = global read "全局 小时数据发送次数.vi" "小时数据发送次数"() -> (w397:i32)
              n184 = global read "全局 小时数据发送次数.vi" "小时数据发送次数"() -> (w398:i32)
              n185 = global read "全局 小时数据发送次数.vi" "小时数据发送次数"() -> (w399:i32)
              n186 = global read "全局 小时数据发送次数.vi" "小时数据发送次数"() -> (w514:i32)
              n187 = case shown="\"2005-212协议\"" w478 {
                tunnel: w512 -> [_ w627]
                tunnel: w511 -> [_ w626]
                tunnel: [w570 w625] -> w510
                tunnel: [w570 w624] -> w509
                tunnel: w508 -> [_ w610]
                tunnel: w507 -> [_ w609]
                tunnel: w506 -> [w568 w608]
                tunnel: [w570 w607] -> w505
                tunnel: [w570 w606] -> w504
                tunnel: [w569 w605] -> w503
                tunnel: w438 -> [_ w582]
                tunnel: [w570 w581] -> w437
                frame "2005-212协议" {
                  w570 = "" ("编码输出")
                  # "瞬时流量"
                  n188 = global read "全局 小时数据发送次数.vi" "小时数据发送次数"() -> (w576:i32)
                  n189 = Index Array(array=w568, index (row)=w576) -> (element=w574:string[])  [unwired: 1 in]
                  n190 = Index Array(array=w574, index #1=5 ("索引"), index #2=1 ("索引")) -> (element #2=w573:string)  [unwired: 1 out]
                  n191 = call "数据编码整合输出.vi"("数据标识"="N", "数据类型"="-Rtd=", "污染物编码"="B01", "数据值"=w573) -> ("编码输出"=w569:string)  [unwired: 7 in]
                }
                frame "2017-212协议", Default {
                  # "累计流量"
                  # "瞬时流量"
                  # "流速"
                  # "水位"
                  # "盐度改COD"
                  # "总铜"
                  n192 = global read "全局 小时数据发送次数.vi" "小时数据发送次数"() -> (w629:i32)
                  n193 = global read "全局 小时数据发送次数.vi" "小时数据发送次数"() -> (w628:i32)
                  n194 = global read "全局 小时数据发送次数.vi" "小时数据发送次数"() -> (w623:i32)
                  n195 = global read "全局 小时数据发送次数.vi" "小时数据发送次数"() -> (w615:i32)
                  n196 = global read "全局 小时数据发送次数.vi" "小时数据发送次数"() -> (w614:i32)
                  n197 = global read "全局 小时数据发送次数.vi" "小时数据发送次数"() -> (w585:i32)
                  n198 = Index Array(array=w627, index (row)=w629) -> (element=w633:string[])  [unwired: 1 in]
                  n199 = Index Array(array=w626, index (row)=w628) -> (element=w632:string[])  [unwired: 1 in]
                  n200 = Index Array(array=w610, index (row)=w623) -> (element=w620:string[])  [unwired: 1 in]
                  n201 = Index Array(array=w609, index (row)=w615) -> (element=w619:string[])  [unwired: 1 in]
                  n202 = Index Array(array=w608, index (row)=w614) -> (element=w611:string[])  [unwired: 1 in]
                  n203 = Index Array(array=w582, index (row)=w585) -> (element=w588:string[])  [unwired: 1 in]
                  n204 = Index Array(array=w633, index #1=5 ("索引"), index #2=3 ("索引")) -> (element #1=w604:string, element #2=w603:string)
                  n205 = Index Array(array=w632, index #1=5 ("索引"), index #2=3 ("索引")) -> (element #1=w602:string, element #2=w601:string)
                  n206 = Index Array(array=w620, index #1=5 ("索引"), index #2=1 ("索引")) -> (element #2=w599:string)  [unwired: 1 out]
                  n207 = Index Array(array=w619, index #1=5 ("索引"), index #2=1 ("索引")) -> (element #2=w598:string)  [unwired: 1 out]
                  n208 = Index Array(array=w611, index #1=5 ("索引"), index #2=1 ("索引")) -> (element #2=w597:string)  [unwired: 1 out]
                  n209 = Index Array(array=w588, index #1=5 ("索引"), index #2=1 ("索引")) -> (element #2=w584:string)  [unwired: 1 out]
                  n210 = call "数据编码整合输出.vi"("数据标识"=w604, "数据类型"="-Rtd=", "污染物编码"="w20122", "数据值"=w603) -> ("编码输出"=w625:string)  [unwired: 7 in]
                  n211 = call "数据编码整合输出.vi"("数据标识"=w602, "数据类型"="-Rtd=", "污染物编码"="w01018", "数据值"=w601) -> ("编码输出"=w624:string)  [unwired: 7 in]
                  n212 = call "数据编码整合输出.vi"("数据标识"="N", "数据类型"="-Rtd=", "污染物编码"="e01201", "数据值"=w599) -> ("编码输出"=w607:string)  [unwired: 7 in]
                  n213 = call "数据编码整合输出.vi"("数据标识"="N", "数据类型"="-Rtd=", "污染物编码"="e01202", "数据值"=w598) -> ("编码输出"=w606:string)  [unwired: 7 in]
                  n214 = call "数据编码整合输出.vi"("数据标识"="N", "数据类型"="-Rtd=", "污染物编码"="e01203", "数据值"=w597) -> ("编码输出"=w605:string)  [unwired: 7 in]
                  n215 = call "数据编码整合输出.vi"("数据标识"="N", "数据类型"="-Rtd=", "污染物编码"="e01204", "数据值"=w584) -> ("编码输出"=w581:string)  [unwired: 7 in]
                }
              }
              n216 = global read "全局 小时数据发送次数.vi" "小时数据发送次数"() -> (w517:i32)
              n217 = global read "全局 小时数据发送次数.vi" "小时数据发送次数"() -> (w453:i32)
              n218 = global read "全局 小时数据发送次数.vi" "小时数据发送次数"() -> (w469:i32)
              n219 = global read "全局 小时数据发送次数.vi" "小时数据发送次数"() -> (w376:i32)
              n220 = global read "全局 小时数据发送次数.vi" "小时数据发送次数"() -> (w460:i32)
              n221 = global read "全局 小时数据发送次数.vi" "小时数据发送次数"() -> (w362:i32)
              n222 = global read "全局 小时数据发送次数.vi" "小时数据发送次数"() -> (w369:i32)
              n223 = global read "全局 小时数据发送次数.vi" "小时数据发送次数"() -> (w518:i32)
              n224 = global read "全局 小时数据发送次数.vi" "小时数据发送次数"() -> (w346:i32)
              n225 = global read "全局 小时数据发送次数.vi" "小时数据发送次数"() -> (w332:i32)
              n226 = global read "全局 小时数据发送次数.vi" "小时数据发送次数"() -> (w339:i32)
              n227 = Index Array(array=w490, index (row)=w491) -> (element=w489:string[])  [unwired: 1 in]
              n228 = Index Array(array=w564, index (row)=w516) -> (element=w546:string[])  [unwired: 1 in]
              n229 = Index Array(array=w565, index (row)=w431) -> (element=w433:string[])  [unwired: 1 in]
              n230 = Index Array(array=w563, index (row)=w423) -> (element=w427:string[])  [unwired: 1 in]
              n231 = Index Array(array=w561, index (row)=w395) -> (element=w419:string[])  [unwired: 1 in]
              n232 = Index Array(array=w562, index (row)=w515) -> (element=w540:string[])  [unwired: 1 in]
              n233 = Index Array(array=w560, index (row)=w396) -> (element=w412:string[])  [unwired: 1 in]
              n234 = Index Array(array=w489, index=0 ("索引")) -> (element=w487:string)
              n235 = Index Array(array=w559, index (row)=w397) -> (element=w411:string[])  [unwired: 1 in]
              n236 = Index Array(array=w557, index (row)=w399) -> (element=w400:string[])  [unwired: 1 in]
              n237 = Index Array(array=w558, index (row)=w398) -> (element=w407:string[])  [unwired: 1 in]
              n238 = Index Array(array=w556, index (row)=w517) -> (element=w533:string[])  [unwired: 1 in]
              n239 = Index Array(array=w546, index #1=3 ("索引"), index #2=5 ("索引")) -> (element #1=w545:string, element #2=w501:string)
              n240 = Index Array(array=w555, index (row)=w518) -> (element=w525:string[])  [unwired: 1 in]
              n241 = Index Array(array=w554, index (row)=w514) -> (element=w523:string[])  [unwired: 1 in]
              n242 = Index Array(array=w443, index (row)=w453) -> (element=w456:string[])  [unwired: 1 in]
              n243 = Index Array(array=w445, index (row)=w469) -> (element=w472:string[])  [unwired: 1 in]
              n244 = Index Array(array=w356, index (row)=w376) -> (element=w373:string[])  [unwired: 1 in]
              n245 = Index Array(array=w444, index (row)=w460) -> (element=w457:string[])  [unwired: 1 in]
              n246 = Index Array(array=w427, index #1=5 ("索引"), index #2=3 ("索引")) -> (element #1=w421:string, element #2=w422:string)
              n247 = Index Array(array=w358, index (row)=w362) -> (element=w359:string[])  [unwired: 1 in]
              n248 = Index Array(array=w357, index (row)=w369) -> (element=w372:string[])  [unwired: 1 in]
              n249 = Index Array(array=w433, index #1=3 ("索引"), index #2=0 ("索引"), index #3=5 ("索引")) -> (element #1=w432:string, element #3=w428:string)  [unwired: 1 out]
              n250 = Index Array(array=w323, index (row)=w346) -> (element=w343:string[])  [unwired: 1 in]
              n251 = Index Array(array=w419, index #1=5 ("索引"), index #2=3 ("索引")) -> (element #1=w392:string, element #2=w393:string)
              n252 = Index Array(array=w325, index (row)=w332) -> (element=w329:string[])  [unwired: 1 in]
              n253 = Index Array(array=w324, index (row)=w339) -> (element=w342:string[])  [unwired: 1 in]
              n254 = Index Array(array=w540, index #1=5 ("索引"), index #2=3 ("索引")) -> (element #1=w500:string, element #2=w499:string)
              n255 = Index Array(array=w412, index #1=5 ("索引"), index #2=3 ("索引")) -> (element #1=w391:string, element #2=w390:string)
              n256 = Index Array(array=w411, index #1=5 ("索引"), index #2=3 ("索引")) -> (element #1=w388:string, element #2=w389:string)
              n257 = Index Array(array=w400, index #1=5 ("索引"), index #2=3 ("索引")) -> (element #1=w384:string, element #2=w385:string)
              n258 = Index Array(array=w407, index #1=5 ("索引"), index #2=3 ("索引")) -> (element #1=w387:string, element #2=w386:string)
              n259 = Index Array(array=w533, index #1=5 ("索引"), index #2=3 ("索引")) -> (element #1=w498:string, element #2=w497:string)
              n260 = Index Array(array=w525, index #1=5 ("索引"), index #2=3 ("索引")) -> (element #1=w496:string, element #2=w495:string)
              n261 = Index Array(array=w523, index #1=5 ("索引"), index #2=3 ("索引")) -> (element #1=w494:string, element #2=w493:string)
              n262 = Index Array(array=w456, index #1=5 ("索引"), index #2=3 ("索引")) -> (element #1=w452:string, element #2=w451:string)
              n263 = Index Array(array=w472, index #1=5 ("索引"), index #2=3 ("索引")) -> (element #1=w468:string, element #2=w467:string)
              n264 = Index Array(array=w373, index #1=5 ("索引"), index #2=3 ("索引")) -> (element #1=w377:string, element #2=w378:string)
              n265 = Index Array(array=w457, index #1=5 ("索引"), index #2=3 ("索引")) -> (element #1=w461:string, element #2=w462:string)
              n266 = Index Array(array=w359, index #1=5 ("索引"), index #2=3 ("索引")) -> (element #1=w363:string, element #2=w364:string)
              n267 = Index Array(array=w372, index #1=5 ("索引"), index #2=3 ("索引")) -> (element #1=w368:string, element #2=w367:string)
              n268 = Index Array(array=w343, index #1=5 ("索引"), index #2=3 ("索引")) -> (element #1=w347:string, element #2=w348:string)
              n269 = Index Array(array=w329, index #1=5 ("索引"), index #2=3 ("索引")) -> (element #1=w333:string, element #2=w334:string)
              n270 = Index Array(array=w342, index #1=5 ("索引"), index #2=3 ("索引")) -> (element #1=w338:string, element #2=w337:string)
              n271 = call "规范时间戳.vi"("字符串"=w487) -> ("result string"=w485:string)  [unwired: 10 in]
              n272 = call "数据编码整合输出.vi"("数据标识"=w501, "数据类型"="-Rtd=", "污染物编码"=w549, "数据值"=w545) -> ("编码输出"=w548:string)  [unwired: 7 in]
              n273 = call "数据编码整合输出.vi"("数据标识"=w421, "数据类型"="-Rtd=", "污染物编码"="w01010", "数据值"=w422) -> ("编码输出"=w544:string)  [unwired: 7 in]
              n274 = call "数据编码整合输出.vi"("数据标识"=w392, "数据类型"="-Rtd=", "污染物编码"="w01009", "数据值"=w393) -> ("编码输出"=w538:string)  [unwired: 7 in]
              n275 = call "数据编码整合输出.vi"("数据标识"=w500, "数据类型"="-Rtd=", "污染物编码"=w542, "数据值"=w499) -> ("编码输出"=w539:string)  [unwired: 7 in]
              n276 = call "数据编码整合输出.vi"("数据标识"=w391, "数据类型"="-Rtd=", "污染物编码"="w01014", "数据值"=w390) -> ("编码输出"=w537:string)  [unwired: 7 in]
              n277 = call "数据编码整合输出.vi"("数据标识"=w388, "数据类型"="-Rtd=", "污染物编码"="w01003", "数据值"=w389) -> ("编码输出"=w536:string)  [unwired: 7 in]
              n278 = call "数据编码整合输出.vi"("数据标识"=w428, "数据类型"="-Rtd=", "污染物编码"="w01019", "数据值"=w432) -> ("编码输出"=w551:string)  [unwired: 7 in]
              n279 = call "数据编码整合输出.vi"("数据标识"=w384, "数据类型"="-Rtd=", "污染物编码"="w19011", "数据值"=w385) -> ("编码输出"=w534:string)  [unwired: 7 in]
              n280 = call "数据编码整合输出.vi"("数据标识"=w387, "数据类型"="-Rtd=", "污染物编码"="w01016", "数据值"=w386) -> ("编码输出"=w535:string)  [unwired: 7 in]
              n281 = call "数据编码整合输出.vi"("数据标识"=w498, "数据类型"="-Rtd=", "污染物编码"=w531, "数据值"=w497) -> ("编码输出"=w529:string)  [unwired: 7 in]
              n282 = call "数据编码整合输出.vi"("数据标识"=w496, "数据类型"="-Rtd=", "污染物编码"=w527, "数据值"=w495) -> ("编码输出"=w524:string)  [unwired: 7 in]
              n283 = call "数据编码整合输出.vi"("数据标识"=w494, "数据类型"="-Rtd=", "污染物编码"=w521, "数据值"=w493) -> ("编码输出"=w519:string)  [unwired: 7 in]
              n284 = call "数据编码整合输出.vi"("数据标识"=w452, "数据类型"="-Rtd=", "污染物编码"="w01100", "数据值"=w451) -> ("编码输出"=w446:string)  [unwired: 7 in]
              n285 = call "数据编码整合输出.vi"("数据标识"=w468, "数据类型"="-Rtd=", "污染物编码"="w21006", "数据值"=w467) -> ("编码输出"=w447:string)  [unwired: 7 in]
              n286 = call "数据编码整合输出.vi"("数据标识"=w377, "数据类型"="-Rtd=", "污染物编码"="w20123", "数据值"=w378) -> ("编码输出"=w352:string)  [unwired: 7 in]
              n287 = call "数据编码整合输出.vi"("数据标识"=w461, "数据类型"="-Rtd=", "污染物编码"="w21019", "数据值"=w462) -> ("编码输出"=w448:string)  [unwired: 7 in]
              n288 = call "数据编码整合输出.vi"("数据标识"=w363, "数据类型"="-Rtd=", "污染物编码"="w20120", "数据值"=w364) -> ("编码输出"=w350:string)  [unwired: 7 in]
              n289 = call "数据编码整合输出.vi"("数据标识"=w368, "数据类型"="-Rtd=", "污染物编码"="w20115", "数据值"=w367) -> ("编码输出"=w351:string)  [unwired: 7 in]
              n290 = call "数据编码整合输出.vi"("数据标识"=w347, "数据类型"="-Rtd=", "污染物编码"="w20111", "数据值"=w348) -> ("编码输出"=w320:string)  [unwired: 7 in]
              n291 = call "数据编码整合输出.vi"("数据标识"=w333, "数据类型"="-Rtd=", "污染物编码"="w20121", "数据值"=w334) -> ("编码输出"=w322:string)  [unwired: 7 in]
              n292 = call "数据编码整合输出.vi"("数据标识"=w338, "数据类型"="-Rtd=", "污染物编码"="w20124", "数据值"=w337) -> ("编码输出"=w321:string)  [unwired: 7 in]
              n293 = Format Into String(format string="DataTime=%s;", w485) -> (resulting string=w484:string)  [unwired: 2 in, 1 out]
              n294 = Format Into String(format string="%s%s%s%s%s%s%s%s%s%s%s%s%s%s%s%s%s%s%s%s%s%s%s%s%s%s%s" ("格式字符串"), w551, w548, w544, w539, w538, w537, w536, w535, w534, w529, w524, w519, w510, w509, w505, w504, w503, w437, w447, w448, w446, w350, w351, w352, w322, w321, w320) -> (resulting string=w483:string)  [unwired: 2 in, 1 out]
              n295 = Concatenate Strings(w484, w483) -> (w440:string)
              n296 = String Length(string=w440) -> (length=w442:i32)
              n297 = Empty String/Path?(string/path=w483) -> (empty?=w513:bool)
              n298 = Decrement(x=w442) -> (x-1=w441:i32)
              n299 = String Subset(string=w440, length (rest)=w441) -> (substring=w439:string)  [unwired: 1 in]
              n300 = case shown="假" w513 {
                tunnel: [w676 ""] -> w553
                tunnel: w439 -> [w676 _]
                frame False {
                  n301 = global read "全局 小时数据发送次数.vi" "小时数据发送次数"() -> (w675:i32)
                  n302 = Increment(x=w675) -> (x+1=w674:i32)
                  n303 = global write "全局 小时数据发送次数.vi" "小时数据发送次数"(w674) -> ()
                }
                frame True {
                  n304 = global read "全局 小时数据发送次数.vi" "小时数据发送次数"() -> (w678:i32)
                  n305 = Increment(x=w678) -> (x+1=w677:i32)
                  n306 = global write "全局 小时数据发送次数.vi" "小时数据发送次数"(w677) -> ()
                }
              }
            }
            frame "返回执行结果" {
            }
          }
        }
        frame "平行样测试" {
          n307 = global read "全局1.vi" "枚举"() -> (w696:enum16{"返回请求应答", "上传数据", "返回执行结果"})
          n308 = case shown="\"上传数据\"" w696 {
            tunnel: ["QnRtn=1" w719 "ExeRtn=1"] -> w695
            tunnel: w694 -> [_ w700 _]
            tunnel: w693 -> [_ w712 _]
            tunnel: w692 -> [_ _ _]
            tunnel: w691 -> [_ _ _]
            tunnel: w690 -> [_ _ _]
            tunnel: w689 -> [_ _ _]
            tunnel: w688 -> [_ _ _]
            tunnel: w687 -> [_ _ _]
            tunnel: w686 -> [_ _ _]
            tunnel: w685 -> [_ w709 _]
            tunnel: w684 -> [_ w707 _]
            tunnel: w683 -> [_ w703 _]
            tunnel: w682 -> [_ _ _]
            tunnel: w681 -> [_ _ _]
            frame "返回请求应答", Default {
            }
            frame "上传数据" {
              # "CODMn"
              n309 = global read "全局 小时数据发送次数.vi" "小时数据发送次数"() -> (w698:i32)
              n310 = Index Array(array=w700, index (row)=w698) -> (element=w717:string[])  [unwired: 1 in]
              n311 = Index Array(array=w717, index=0 ("索引")) -> (element=w714:string)
              n312 = call "规范时间戳.vi"("字符串"=w714) -> ("result string"=w715:string)  [unwired: 10 in]
              n313 = call "平行样集成干预数据组合(子VI).vi"("污染物编码"="w21001", "数据输入"=w707, "小时数据发送次数"=w698) -> ("输出组合"=w705:string)  [unwired: 8 in]
              n314 = call "平行样集成干预数据组合(子VI).vi"("污染物编码"="w01018", "数据输入"=w703, "小时数据发送次数"=w698) -> ("输出组合"=w702:string)  [unwired: 8 in]
              n315 = call "平行样集成干预数据组合(子VI).vi"("污染物编码"="w21011", "数据输入"=w709, "小时数据发送次数"=w698) -> ("输出组合"=w708:string)  [unwired: 8 in]
              n316 = call "平行样集成干预数据组合(子VI).vi"("污染物编码"="w21003", "数据输入"=w712, "小时数据发送次数"=w698) -> ("输出组合"=w711:string)  [unwired: 8 in]
              n317 = call "平行样集成干预数据组合(子VI).vi"("污染物编码"="w01019", "数据输入"=w700, "小时数据发送次数"=w698) -> ("输出组合"=w699:string)  [unwired: 8 in]
              n318 = Empty String/Path?(string/path=w714) -> (empty?=w718:bool)
              n319 = Format Into String(format string="DataTime=%s;%s%s%s%s%s" ("格式字符串"), w715, w699, w711, w708, w705, w702) -> (resulting string=w720:string)  [unwired: 2 in, 1 out]
              n320 = case shown="真" w718 {
                tunnel: [w724 ""] -> w719
                tunnel: w720 -> [w724 _]
                frame False {
                  n321 = global read "全局 小时数据发送次数.vi" "小时数据发送次数"() -> (w723:i32)
                  n322 = Increment(x=w723) -> (x+1=w722:i32)
                  n323 = global write "全局 小时数据发送次数.vi" "小时数据发送次数"(w722) -> ()
                }
                frame True {
                  n324 = global read "全局 小时数据发送次数.vi" "小时数据发送次数"() -> (w726:i32)
                  n325 = Increment(x=w726) -> (x+1=w725:i32)
                  n326 = global write "全局 小时数据发送次数.vi" "小时数据发送次数"(w725) -> ()
                }
              }
            }
            frame "返回执行结果" {
            }
          }
        }
        frame "集成干预测试" {
          n327 = global read "全局1.vi" "枚举"() -> (w747:enum16{"返回请求应答", "上传数据", "返回执行结果"})
          n328 = case shown="\"上传数据\"" w747 {
            tunnel: ["QnRtn=1" w800 "ExeRtn=1"] -> w746
            tunnel: w745 -> [_ w793 _]
            tunnel: w744 -> [_ w790 _]
            tunnel: w743 -> [_ w787 _]
            tunnel: w742 -> [_ w785 _]
            tunnel: w741 -> [_ w781 _]
            tunnel: w740 -> [_ w779 _]
            tunnel: w739 -> [_ w775 _]
            tunnel: w738 -> [_ w772 _]
            tunnel: w737 -> [_ w769 _]
            tunnel: w736 -> [_ w766 _]
            tunnel: w735 -> [_ w763 _]
            tunnel: w734 -> [_ w760 _]
            tunnel: w733 -> [_ _ _]
            tunnel: w732 -> [_ _ _]
            tunnel: w731 -> [_ w758 _]
            tunnel: w730 -> [_ w755 _]
            tunnel: w729 -> [_ w752 _]
            frame "返回请求应答", Default {
            }
            frame "上传数据" {
              # "CODMn"
              n329 = global read "全局 小时数据发送次数.vi" "小时数据发送次数"() -> (w751:i32)
              n330 = Index Array(array=w793, index (row)=w751) -> (element=w798:string[])  [unwired: 1 in]
              n331 = Index Array(array=w798, index=0 ("索引")) -> (element=w795:string)
              n332 = call "规范时间戳.vi"("字符串"=w795) -> ("result string"=w796:string)  [unwired: 10 in]
              n333 = call "平行样集成干预数据组合(子VI).vi"("污染物编码"="w21003", "数据输入"=w790, "小时数据发送次数"=w751) -> ("输出组合"=w789:string)  [unwired: 8 in]
              n334 = call "平行样集成干预数据组合(子VI).vi"("污染物编码"="w01019", "数据输入"=w793, "小时数据发送次数"=w751) -> ("输出组合"=w792:string)  [unwired: 8 in]
              n335 = call "平行样集成干预数据组合(子VI).vi"("污染物编码"="w01010", "数据输入"=w787, "小时数据发送次数"=w751) -> ("输出组合"=w786:string)  [unwired: 8 in]
              n336 = call "平行样集成干预数据组合(子VI).vi"("污染物编码"="w01001", "数据输入"=w785, "小时数据发送次数"=w751) -> ("输出组合"=w783:string)  [unwired: 8 in]
              n337 = call "平行样集成干预数据组合(子VI).vi"("污染物编码"="w01009", "数据输入"=w781, "小时数据发送次数"=w751) -> ("输出组合"=w780:string)  [unwired: 8 in]
              n338 = call "平行样集成干预数据组合(子VI).vi"("污染物编码"="w01003", "数据输入"=w775, "小时数据发送次数"=w751) -> ("输出组合"=w774:string)  [unwired: 8 in]
              n339 = call "平行样集成干预数据组合(子VI).vi"("污染物编码"="w01014", "数据输入"=w779, "小时数据发送次数"=w751) -> ("输出组合"=w777:string)  [unwired: 8 in]
              n340 = call "平行样集成干预数据组合(子VI).vi"("污染物编码"="w21019", "数据输入"=w755, "小时数据发送次数"=w751) -> ("输出组合"=w753:string)  [unwired: 8 in]
              n341 = call "平行样集成干预数据组合(子VI).vi"("污染物编码"="w01100", "数据输入"=w752, "小时数据发送次数"=w751) -> ("输出组合"=w749:string)  [unwired: 8 in]
              n342 = call "平行样集成干预数据组合(子VI).vi"("污染物编码"="w01016", "数据输入"=w772, "小时数据发送次数"=w751) -> ("输出组合"=w771:string)  [unwired: 8 in]
              n343 = call "平行样集成干预数据组合(子VI).vi"("污染物编码"="w19011", "数据输入"=w769, "小时数据发送次数"=w751) -> ("输出组合"=w768:string)  [unwired: 8 in]
              n344 = call "平行样集成干预数据组合(子VI).vi"("污染物编码"="w21001", "数据输入"=w763, "小时数据发送次数"=w751) -> ("输出组合"=w762:string)  [unwired: 8 in]
              n345 = call "平行样集成干预数据组合(子VI).vi"("污染物编码"="w21006", "数据输入"=w758, "小时数据发送次数"=w751) -> ("输出组合"=w756:string)  [unwired: 8 in]
              n346 = call "平行样集成干预数据组合(子VI).vi"("污染物编码"="w01018", "数据输入"=w760, "小时数据发送次数"=w751) -> ("输出组合"=w759:string)  [unwired: 8 in]
              n347 = call "平行样集成干预数据组合(子VI).vi"("污染物编码"="w21011", "数据输入"=w766, "小时数据发送次数"=w751) -> ("输出组合"=w765:string)  [unwired: 8 in]
              n348 = Empty String/Path?(string/path=w795) -> (empty?=w799:bool)
              n349 = Format Into String(format string="DataTime=%s;%s%s%s%s%s%s%s%s%s%s%s%s%s%s%s" ("格式字符串"), w796, w792, w789, w786, w783, w780, w777, w774, w771, w768, w765, w762, w759, w756, w753, w749) -> (resulting string=w801:string)  [unwired: 2 in, 1 out]
              n350 = case shown="真" w799 {
                tunnel: [w805 ""] -> w800
                tunnel: w801 -> [w805 _]
                frame False {
                  n351 = global read "全局 小时数据发送次数.vi" "小时数据发送次数"() -> (w804:i32)
                  n352 = Increment(x=w804) -> (x+1=w803:i32)
                  n353 = global write "全局 小时数据发送次数.vi" "小时数据发送次数"(w803) -> ()
                }
                frame True {
                  n354 = global read "全局 小时数据发送次数.vi" "小时数据发送次数"() -> (w807:i32)
                  n355 = Increment(x=w807) -> (x+1=w806:i32)
                  n356 = global write "全局 小时数据发送次数.vi" "小时数据发送次数"(w806) -> ()
                }
              }
            }
            frame "返回执行结果" {
            }
          }
        }
        frame "加标回收测试" {
          n357 = global read "全局1.vi" "枚举"() -> (w824:enum16{"返回请求应答", "上传数据", "返回执行结果"})
          n358 = case shown="\"上传数据\"" w824 {
            tunnel: ["QnRtn=1" w1047 "ExeRtn=1"] -> w825
            tunnel: w823 -> [_ w1053 _]
            tunnel: w822 -> [_ w1052 _]
            tunnel: w821 -> [_ w1051 _]
            tunnel: w820 -> [_ _ _]
            tunnel: w819 -> [_ _ _]
            tunnel: w818 -> [_ _ _]
            tunnel: w817 -> [_ _ _]
            tunnel: w816 -> [_ _ _]
            tunnel: w815 -> [_ _ _]
            tunnel: w814 -> [_ _ _]
            tunnel: w813 -> [_ w1050 _]
            tunnel: w812 -> [_ w1049 _]
            tunnel: w811 -> [_ _ _]
            tunnel: w810 -> [_ _ _]
            frame "返回请求应答", Default {
            }
            frame "上传数据" {
              # "w01001-Check=63.0,w01001-WaterTime=20160801080000,w01001-Water=45.23,w01001-Chroma=1000,w01001-Volume=0.2,w01001-DVolume=200,w01003-Flag=N;"
              # "CODCr"
              # "总氮"
              # "总磷"
              # "NH3"
              # "CODMn"
              n359 = global read "全局 小时数据发送次数.vi" "小时数据发送次数"() -> (w1054:i32)
              n360 = Index Array(array=w1052, index (row)=w1054) -> (element=w1059:string[])  [unwired: 1 in]
              n361 = Index Array(array=w1049, index (row)=w1054) -> (element=w1061:string[])  [unwired: 1 in]
              n362 = Index Array(array=w1050, index (row)=w1054) -> (element=w1063:string[])  [unwired: 1 in]
              n363 = Index Array(array=w1059, index #1=4 ("索引"), index #2=2 ("索引"), index #3=3 ("索引"), index #4=5 ("索引"), index #5=6 ("索引"), index #6=7 ("索引")) -> (element #1=w948:string, element #2=w842:string, element #3=w933:string, element #4=w932:string, element #5=w931:string, element #6=w930:string)
              n364 = Index Array(array=w1051, index (row)=w1054) -> (element=w1060:string[])  [unwired: 1 in]
              n365 = Index Array(array=w1053, index (row)=w1054) -> (element=w1058:string[])  [unwired: 1 in]
              n366 = Index Array(array=w1063, index #1=4 ("索引"), index #2=2 ("索引"), index #3=3 ("索引"), index #4=5 ("索引"), index #5=6 ("索引"), index #6=7 ("索引")) -> (element #1=w1018:string, element #2=w846:string, element #3=w998:string, element #4=w997:string, element #5=w996:string, element #6=w995:string)
              n367 = Index Array(array=w1061, index #1=0 ("索引"), index #2=4 ("索引"), index #3=2 ("索引"), index #4=3 ("索引"), index #5=5 ("索引"), index #6=6 ("索引"), index #7=7 ("索引")) -> (element #1=w1056:string, element #2=w1044:string, element #3=w868:string, element #4=w1036:string, element #5=w1033:string, element #6=w1029:string, element #7=w1028:string)
              n368 = Index Array(array=w1060, index #1=4 ("索引"), index #2=2 ("索引"), index #3=3 ("索引"), index #4=5 ("索引"), index #5=6 ("索引"), index #6=7 ("索引")) -> (element #1=w976:string, element #2=w844:string, element #3=w953:string, element #4=w952:string, element #5=w951:string, element #6=w950:string)
              n369 = Index Array(array=w1058, index #1=4 ("索引"), index #2=2 ("索引"), index #3=3 ("索引"), index #4=5 ("索引"), index #5=6 ("索引"), index #6=7 ("索引")) -> (element #1=w946:string, element #2=w840:string, element #3=w883:string, element #4=w884:string, element #5=w885:string, element #6=w886:string)
              n370 = call "规范时间戳.vi"("字符串"=w1056) -> ("result string"=w1055:string)  [unwired: 10 in]
              n371 = call "规范时间戳.vi"("字符串"=w868) -> ("result string"=w867:string)  [unwired: 10 in]
              n372 = call "规范时间戳.vi"("字符串"=w842) -> ("result string"=w841:string)  [unwired: 10 in]
              n373 = call "规范时间戳.vi"("字符串"=w844) -> ("result string"=w843:string)  [unwired: 10 in]
              n374 = call "规范时间戳.vi"("字符串"=w846) -> ("result string"=w845:string)  [unwired: 10 in]
              n375 = call "规范时间戳.vi"("字符串"=w840) -> ("result string"=w839:string)  [unwired: 10 in]
              n376 = call "核查数据编码整合输出.vi"("字段结束"=FALSE, "数据标识"="N" ("字符串"), "数据类型"="-Check=", "污染物编码"="w21011", "数据值"=w976) -> ("编码输出"=w975:string)  [unwired: 6 in]
              n377 = call "核查数据编码整合输出.vi"("字段结束"=FALSE, "数据标识"="N" ("字符串"), "数据类型"="-WaterTime=", "污染物编码"="w21011", "数据值"=w843) -> ("编码输出"=w958:string)  [unwired: 6 in]
              n378 = call "核查数据编码整合输出.vi"("字段结束"=FALSE, "数据标识"="N" ("字符串"), "数据类型"="-Water=", "污染物编码"="w21011", "数据精度"=2, "数据值"=w953) -> ("编码输出"=w957:string)  [unwired: 5 in]
              n379 = call "核查数据编码整合输出.vi"("字段结束"=TRUE, "数据标识"="N" ("字符串"), "数据类型"="-DVolume=", "污染物编码"="w21011", "数据值"=w950) -> ("编码输出"=w954:string)  [unwired: 6 in]
              n380 = call "核查数据编码整合输出.vi"("字段结束"=FALSE, "数据标识"="N" ("字符串"), "数据类型"="-Chroma=", "污染物编码"="w21011", "数据值"=w952) -> ("编码输出"=w956:string)  [unwired: 6 in]
              n381 = call "核查数据编码整合输出.vi"("字段结束"=FALSE, "数据标识"="N" ("字符串"), "数据类型"="-Volume=", "污染物编码"="w21011", "数据值"=w951) -> ("编码输出"=w955:string)  [unwired: 6 in]
              n382 = call "核查数据编码整合输出.vi"("字段结束"=FALSE, "数据标识"="N" ("字符串"), "数据类型"="-WaterTime=", "污染物编码"="w21001", "数据值"=w841) -> ("编码输出"=w928:string)  [unwired: 6 in]
              n383 = call "核查数据编码整合输出.vi"("字段结束"=FALSE, "数据类型"="-Volume=", "污染物编码"="w01019", "数据值"=w1029) -> ("编码输出"=w1021:string)  [unwired: 7 in]
              n384 = call "核查数据编码整合输出.vi"("字段结束"=FALSE, "数据标识"="N" ("字符串"), "数据类型"="-Check=", "污染物编码"="w21001", "数据值"=w948) -> ("编码输出"=w929:string)  [unwired: 6 in]
              n385 = call "核查数据编码整合输出.vi"("字段结束"=FALSE, "数据标识"="N" ("字符串"), "数据类型"="-Water=", "污染物编码"="w21001", "数据精度"=2, "数据值"=w933) -> ("编码输出"=w927:string)  [unwired: 5 in]
              n386 = call "核查数据编码整合输出.vi"("字段结束"=FALSE, "数据标识"="N" ("字符串"), "数据类型"="-Chroma=", "污染物编码"="w21001", "数据值"=w932) -> ("编码输出"=w926:string)  [unwired: 6 in]
              n387 = call "核查数据编码整合输出.vi"("字段结束"=FALSE, "数据标识"="N" ("字符串"), "数据类型"="-Volume=", "污染物编码"="w21001", "数据值"=w931) -> ("编码输出"=w925:string)  [unwired: 6 in]
              n388 = call "核查数据编码整合输出.vi"("字段结束"=TRUE, "数据标识"="N" ("字符串"), "数据类型"="-DVolume=", "污染物编码"="w21001", "数据值"=w930) -> ("编码输出"=w924:string)  [unwired: 6 in]
              n389 = call "核查数据编码整合输出.vi"("字段结束"=TRUE, "数据类型"="-DVolume=", "污染物编码"="w01019", "数据值"=w1028) -> ("编码输出"=w1020:string)  [unwired: 7 in]
              n390 = call "核查数据编码整合输出.vi"("字段结束"=FALSE, "数据类型"="-Chroma=", "污染物编码"="w01019", "数据值"=w1033) -> ("编码输出"=w1022:string)  [unwired: 7 in]
              n391 = call "核查数据编码整合输出.vi"("字段结束"=FALSE, "数据标识"="N" ("字符串"), "数据类型"="-Check=", "污染物编码"="w21003", "数据值"=w1018) -> ("编码输出"=w989:string)  [unwired: 6 in]
              n392 = call "核查数据编码整合输出.vi"("字段结束"=FALSE, "数据标识"="N" ("字符串"), "数据类型"="-WaterTime=", "污染物编码"="w21003", "数据值"=w845) -> ("编码输出"=w988:string)  [unwired: 6 in]
              n393 = call "核查数据编码整合输出.vi"("字段结束"=FALSE, "数据标识"="N" ("字符串"), "数据类型"="-Check=", "污染物编码"="w01019", "数据值"=w1044) -> ("编码输出"=w1025:string)  [unwired: 6 in]
              n394 = call "核查数据编码整合输出.vi"("字段结束"=FALSE, "数据类型"="-WaterTime=", "污染物编码"="w01019", "数据值"=w867) -> ("编码输出"=w1024:string)  [unwired: 7 in]
              n395 = call "核查数据编码整合输出.vi"("字段结束"=FALSE, "数据标识"="N" ("字符串"), "数据类型"="-Water=", "污染物编码"="w21003", "数据精度"=2, "数据值"=w998) -> ("编码输出"=w987:string)  [unwired: 5 in]
              n396 = call "核查数据编码整合输出.vi"("字段结束"=FALSE, "数据类型"="-Water=", "污染物编码"="w01019", "数据精度"=2, "数据值"=w1036) -> ("编码输出"=w1023:string)  [unwired: 6 in]
              n397 = call "核查数据编码整合输出.vi"("字段结束"=FALSE, "数据标识"="N" ("字符串"), "数据类型"="-Chroma=", "污染物编码"="w21003", "数据值"=w997) -> ("编码输出"=w986:string)  [unwired: 6 in]
              n398 = call "核查数据编码整合输出.vi"("字段结束"=FALSE, "数据标识"="N" ("字符串"), "数据类型"="-Volume=", "污染物编码"="w21003", "数据值"=w996) -> ("编码输出"=w985:string)  [unwired: 6 in]
              n399 = call "核查数据编码整合输出.vi"("字段结束"=TRUE, "数据标识"="N" ("字符串"), "数据类型"="-DVolume=", "污染物编码"="w21003", "数据值"=w995) -> ("编码输出"=w984:string)  [unwired: 6 in]
              n400 = call "核查数据编码整合输出.vi"("字段结束"=FALSE, "数据标识"="N" ("字符串"), "数据类型"="-Check=", "污染物编码"="w01018", "数据值"=w946) -> ("编码输出"=w901:string)  [unwired: 6 in]
              n401 = call "核查数据编码整合输出.vi"("字段结束"=FALSE, "数据标识"="N" ("字符串"), "数据类型"="-Water=", "污染物编码"="w01018", "数据精度"=2, "数据值"=w883) -> ("编码输出"=w899:string)  [unwired: 5 in]
              n402 = call "核查数据编码整合输出.vi"("字段结束"=FALSE, "数据标识"="N" ("字符串"), "数据类型"="-WaterTime=", "污染物编码"="w01018", "数据值"=w839) -> ("编码输出"=w900:string)  [unwired: 6 in]
              n403 = call "核查数据编码整合输出.vi"("字段结束"=FALSE, "数据标识"="N" ("字符串"), "数据类型"="-Chroma=", "污染物编码"="w01018", "数据值"=w884) -> ("编码输出"=w898:string)  [unwired: 6 in]
              n404 = call "核查数据编码整合输出.vi"("字段结束"=FALSE, "数据标识"="N" ("字符串"), "数据类型"="-Volume=", "污染物编码"="w01018", "数据值"=w885) -> ("编码输出"=w897:string)  [unwired: 6 in]
              n405 = call "核查数据编码整合输出.vi"("字段结束"=TRUE, "数据标识"="N" ("字符串"), "数据类型"="-DVolume=", "污染物编码"="w01018", "数据值"=w886) -> ("编码输出"=w896:string)  [unwired: 6 in]
              n406 = Concatenate Strings(w975, w958, w957, w956, w955, w954) -> (w944:string)
              n407 = Concatenate Strings(w1025, w1024, w1023, w1022, w1021, w1020) -> (w1019:string)
              n408 = Concatenate Strings(w989, w988, w987, w986, w985, w984) -> (w983:string)
              n409 = Concatenate Strings(w929, w928, w927, w926, w925, w924) -> (w879:string)
              n410 = Empty String/Path?(string/path=w1055) -> (empty?=w1046:bool)
              n411 = Concatenate Strings(w901, w900, w899, w898, w897, w896) -> (w878:string)
              n412 = Format Into String(format string="DataTime=%s;%s%s%s%s%s" ("格式字符串"), w1055, w1019, w983, w944, w879, w878) -> (resulting string=w1048:string)  [unwired: 2 in, 1 out]
              n413 = case shown="真" w1046 {
                tunnel: [w1067 ""] -> w1047
                tunnel: w1048 -> [w1067 _]
                frame False {
                  n414 = global read "全局 小时数据发送次数.vi" "小时数据发送次数"() -> (w1066:i32)
                  n415 = Increment(x=w1066) -> (x+1=w1065:i32)
                  n416 = global write "全局 小时数据发送次数.vi" "小时数据发送次数"(w1065) -> ()
                }
                frame True {
                  n417 = global read "全局 小时数据发送次数.vi" "小时数据发送次数"() -> (w1069:i32)
                  n418 = Increment(x=w1069) -> (x+1=w1068:i32)
                  n419 = global write "全局 小时数据发送次数.vi" "小时数据发送次数"(w1068) -> ()
                }
              }
            }
            frame "返回执行结果" {
            }
          }
        }
        frame "核查数据" {
          n420 = global read "全局1.vi" "枚举"() -> (w1086:enum16{"返回请求应答", "上传数据", "返回执行结果"})
          n421 = case shown="\"上传数据\"" w1086 {
            tunnel: ["QnRtn=1" w1134 "ExeRtn=1"] -> w1087
            tunnel: w1085 -> [_ w1127 _]
            tunnel: w1084 -> [_ w1132 _]
            tunnel: w1083 -> [_ w1124 _]
            tunnel: w1082 -> [_ w1121 _]
            tunnel: w1081 -> [_ w1118 _]
            tunnel: w1080 -> [_ w1115 _]
            tunnel: w1079 -> [_ w1112 _]
            tunnel: w1078 -> [_ w1109 _]
            tunnel: w1077 -> [_ w1106 _]
            tunnel: w1076 -> [_ w1094 _]
            tunnel: w1075 -> [_ w1091 _]
            tunnel: w1074 -> [_ w1103 _]
            tunnel: w1073 -> [_ w1100 _]
            tunnel: w1072 -> [_ w1097 _]
            frame "返回请求应答", Default {
            }
            frame "上传数据" {
              # "将非空数组的时间戳写入"
              n422 = global read "全局 小时数据发送次数.vi" "小时数据发送次数"() -> (w1090:i32)
              n423 = Index Array(array=w1127, index (row)=w1090) -> (element=w1133:string[])  [unwired: 1 in]
              n424 = Index Array(array=w1133, index=0 ("索引")) -> (element=w1131:string)
              n425 = call "规范分钟数据时间戳.vi"("字符串"=w1131) -> ("result string"=w1130:string)  [unwired: 10 in]
              n426 = call "标样核查数据组合(子VI).vi"("小时数据发送次数"=w1090, "数据输入"=w1097, "污染物编码"="w21006") -> ("输出组合"=w1096:string)  [unwired: 8 in]
              n427 = call "标样核查数据组合(子VI).vi"("小时数据发送次数"=w1090, "数据输入"=w1127, "污染物编码"="w01019") -> ("输出组合"=w1126:string)  [unwired: 8 in]
              n428 = call "标样核查数据组合(子VI).vi"("小时数据发送次数"=w1090, "数据输入"=w1103, "污染物编码"="w01100") -> ("输出组合"=w1102:string)  [unwired: 8 in]
              n429 = call "标样核查数据组合(子VI).vi"("小时数据发送次数"=w1090, "数据输入"=w1100, "污染物编码"="w21019") -> ("输出组合"=w1099:string)  [unwired: 8 in]
              n430 = call "标样核查数据组合(子VI).vi"("小时数据发送次数"=w1090, "数据输入"=w1091, "污染物编码"="w19011") -> ("输出组合"=w1089:string)  [unwired: 8 in]
              n431 = call "标样核查数据组合(子VI).vi"("小时数据发送次数"=w1090, "数据输入"=w1132, "污染物编码"="w21003") -> ("输出组合"=w1135:string)  [unwired: 8 in]
              n432 = call "标样核查数据组合(子VI).vi"("小时数据发送次数"=w1090, "数据输入"=w1094, "污染物编码"="w01016") -> ("输出组合"=w1093:string)  [unwired: 8 in]
              n433 = call "标样核查数据组合(子VI).vi"("小时数据发送次数"=w1090, "数据输入"=w1124, "污染物编码"="w21011") -> ("输出组合"=w1123:string)  [unwired: 8 in]
              n434 = call "标样核查数据组合(子VI).vi"("小时数据发送次数"=w1090, "数据输入"=w1121, "污染物编码"="w21001") -> ("输出组合"=w1120:string)  [unwired: 8 in]
              n435 = call "标样核查数据组合(子VI).vi"("小时数据发送次数"=w1090, "数据输入"=w1118, "污染物编码"="w01018") -> ("输出组合"=w1117:string)  [unwired: 8 in]
              n436 = call "标样核查数据组合(子VI).vi"("小时数据发送次数"=w1090, "数据输入"=w1115, "污染物编码"="w01001") -> ("输出组合"=w1114:string)  [unwired: 8 in]
              n437 = call "标样核查数据组合(子VI).vi"("小时数据发送次数"=w1090, "数据输入"=w1112, "污染物编码"="w01009") -> ("输出组合"=w1111:string)  [unwired: 8 in]
              n438 = call "标样核查数据组合(子VI).vi"("小时数据发送次数"=w1090, "数据输入"=w1109, "污染物编码"="w01014") -> ("输出组合"=w1108:string)  [unwired: 8 in]
              n439 = call "标样核查数据组合(子VI).vi"("小时数据发送次数"=w1090, "数据输入"=w1106, "污染物编码"="w01003") -> ("输出组合"=w1105:string)  [unwired: 8 in]
              n440 = Format Into String(format string="DataTime=%s;%s%s%s%s%s%s%s%s%s%s%s%s%s%s" ("格式字符串"), w1130, w1126, w1135, w1123, w1120, w1117, w1114, w1111, w1108, w1105, w1093, w1089, w1096, w1099, w1102) -> (resulting string=w1136:string)  [unwired: 2 in, 1 out]
              n441 = Empty String/Path?(string/path=w1130) -> (empty?=w1137:bool)
              n442 = case shown="假" w1137 {
                tunnel: [w1142 ""] -> w1134
                tunnel: w1136 -> [w1142 _]
                frame False {
                  n443 = global read "全局 小时数据发送次数.vi" "小时数据发送次数"() -> (w1141:i32)
                  n444 = Increment(x=w1141) -> (x+1=w1140:i32)
                  n445 = global write "全局 小时数据发送次数.vi" "小时数据发送次数"(w1140) -> ()
                }
                frame True {
                  n446 = global read "全局 小时数据发送次数.vi" "小时数据发送次数"() -> (w1144:i32)
                  n447 = Increment(x=w1144) -> (x+1=w1143:i32)
                  n448 = global write "全局 小时数据发送次数.vi" "小时数据发送次数"(w1143) -> ()
                }
              }
            }
            frame "返回执行结果" {
            }
          }
        }
        frame "空白测试", "跨度核查" {
          n449 = global read "全局1.vi" "枚举"() -> (w1155:enum16{"返回请求应答", "上传数据", "返回执行结果"})
          n450 = case shown="\"上传数据\"" w1155 {
            tunnel: ["QnRtn=1" w1220 "ExeRtn=1"] -> w1156
            tunnel: w1154 -> [_ w1226 _]
            tunnel: w1153 -> [_ w1225 _]
            tunnel: w1152 -> [_ w1224 _]
            tunnel: w1151 -> [_ w1223 _]
            tunnel: w1150 -> [_ w1222 _]
            tunnel: w1149 -> [_ w1197 _]
            tunnel: w1148 -> [_ w1196 _]
            tunnel: w1147 -> [_ w1195 _]
            frame "返回请求应答", Default {
            }
            frame "上传数据" {
              n451 = global read "全局 小时数据发送次数.vi" "小时数据发送次数"() -> (w1213:i32)
              n452 = global read "全局 小时数据发送次数.vi" "小时数据发送次数"() -> (w1214:i32)
              n453 = global read "全局 小时数据发送次数.vi" "小时数据发送次数"() -> (w1217:i32)
              n454 = global read "全局 小时数据发送次数.vi" "小时数据发送次数"() -> (w1216:i32)
              n455 = global read "全局 小时数据发送次数.vi" "小时数据发送次数"() -> (w1200:i32)
              n456 = global read "全局 小时数据发送次数.vi" "小时数据发送次数"() -> (w1199:i32)
              n457 = global read "全局 小时数据发送次数.vi" "小时数据发送次数"() -> (w1215:i32)
              n458 = global read "全局 小时数据发送次数.vi" "小时数据发送次数"() -> (w1198:i32)
              n459 = Index Array(array=w1225, index (row)=w1214) -> (element=w1242:string[])  [unwired: 1 in]
              n460 = Index Array(array=w1226, index (row)=w1213) -> (element=w1240:string[])  [unwired: 1 in]
              n461 = Index Array(array=w1223, index (row)=w1217) -> (element=w1236:string[])  [unwired: 1 in]
              n462 = Index Array(array=w1222, index (row)=w1216) -> (element=w1235:string[])  [unwired: 1 in]
              n463 = Index Array(array=w1196, index (row)=w1200) -> (element=w1206:string[])  [unwired: 1 in]
              n464 = Index Array(array=w1195, index (row)=w1199) -> (element=w1205:string[])  [unwired: 1 in]
              n465 = Index Array(array=w1224, index (row)=w1215) -> (element=w1239:string[])  [unwired: 1 in]
              n466 = Index Array(array=w1197, index (row)=w1198) -> (element=w1209:string[])  [unwired: 1 in]
              n467 = Index Array(array=w1242, index #1=3 ("索引"), index #2=7 ("索引")) -> (element #1=w1191:string, element #2=w1190:string)
              n468 = Index Array(array=w1240, index #1=0 ("索引"), index #2=3 ("索引"), index #3=7 ("索引")) -> (element #1=w1211:string, element #2=w1212:string, element #3=w1218:string)
              n469 = Index Array(array=w1236, index #1=3 ("索引"), index #2=7 ("索引")) -> (element #1=w1181:string, element #2=w1180:string)
              n470 = Index Array(array=w1235, index #1=3 ("索引"), index #2=7 ("索引")) -> (element #1=w1176:string, element #2=w1175:string)
              n471 = Index Array(array=w1206, index #1=3 ("索引"), index #2=7 ("索引")) -> (element #1=w1166:string, element #2=w1165:string)
              n472 = Index Array(array=w1205, index #1=3 ("索引"), index #2=7 ("索引")) -> (element #1=w1162:string, element #2=w1161:string)
              n473 = Index Array(array=w1239, index #1=3 ("索引"), index #2=7 ("索引")) -> (element #1=w1186:string, element #2=w1185:string)
              n474 = Index Array(array=w1209, index #1=3 ("索引"), index #2=7 ("索引")) -> (element #1=w1171:string, element #2=w1170:string)
              n475 = call "规范小时时间戳.vi"("字符串"=w1211) -> ("result string"=w1210:string)  [unwired: 10 in]
              n476 = call "零点跨度数据组合 (子VI).vi"("span value"="0", "standard value"=w1161, "check value"=w1162, "污染物编码"="w01100") -> ("组合输出"=w1158:string)  [unwired: 7 in]
              n477 = call "零点跨度数据组合 (子VI).vi"("span value"="0", "standard value"=w1165, "check value"=w1166, "污染物编码"="w21019") -> ("组合输出"=w1164:string)  [unwired: 7 in]
              n478 = call "零点跨度数据组合 (子VI).vi"("span value"="0", "standard value"=w1190, "check value"=w1191, "污染物编码"="w21003") -> ("组合输出"=w1188:string)  [unwired: 7 in]
              n479 = call "零点跨度数据组合 (子VI).vi"("span value"="0", "standard value"=w1218, "check value"=w1212, "污染物编码"="w01019") -> ("组合输出"=w1232:string)  [unwired: 7 in]
              n480 = call "零点跨度数据组合 (子VI).vi"("span value"="0", "standard value"=w1185, "check value"=w1186, "污染物编码"="w21011") -> ("组合输出"=w1184:string)  [unwired: 7 in]
              n481 = call "零点跨度数据组合 (子VI).vi"("span value"="0", "standard value"=w1180, "check value"=w1181, "污染物编码"="w21001") -> ("组合输出"=w1179:string)  [unwired: 7 in]
              n482 = call "零点跨度数据组合 (子VI).vi"("span value"="0", "standard value"=w1175, "check value"=w1176, "污染物编码"="w01018") -> ("组合输出"=w1174:string)  [unwired: 7 in]
              n483 = call "零点跨度数据组合 (子VI).vi"("span value"="0", "standard value"=w1170, "check value"=w1171, "污染物编码"="w21006") -> ("组合输出"=w1169:string)  [unwired: 7 in]
              n484 = Format Into String(format string="DataTime=%s;%s%s%s%s%s%s%s%s" ("格式字符串"), w1210, w1232, w1188, w1184, w1179, w1174, w1169, w1164, w1158) -> (resulting string=w1219:string)  [unwired: 2 in, 1 out]
              n485 = Empty String/Path?(string/path=w1210) -> (empty?=w1221:bool)
              n486 = case shown="假" w1221 {
                tunnel: [w1245 ""] -> w1220
                tunnel: w1219 -> [w1245 _]
                frame False {
                  n487 = global read "全局 小时数据发送次数.vi" "小时数据发送次数"() -> (w1247:i32)
                  n488 = Increment(x=w1247) -> (x+1=w1246:i32)
                  n489 = global write "全局 小时数据发送次数.vi" "小时数据发送次数"(w1246) -> ()
                }
                frame True {
                  n490 = global read "全局 小时数据发送次数.vi" "小时数据发送次数"() -> (w1249:i32)
                  n491 = Increment(x=w1249) -> (x+1=w1248:i32)
                  n492 = global write "全局 小时数据发送次数.vi" "小时数据发送次数"(w1248) -> ()
                }
              }
            }
            frame "返回执行结果" {
            }
          }
        }
      }
    }
    frame "小时数据" {
      # "藻密度"
      # "叶绿素"
      # "浊度"
      # "水温"
      # "发送小时数据"
      n493 = global read "全局 小时数据发送次数.vi" "小时数据发送次数"() -> (w1306:i32)
      n494 = global read "全局 小时数据发送次数.vi" "小时数据发送次数"() -> (w1307:i32)
      n495 = global read "全局 小时数据发送次数.vi" "小时数据发送次数"() -> (w1294:i32)
      n496 = global read "全局 小时数据发送次数.vi" "小时数据发送次数"() -> (w1290:i32)
      n497 = global read "全局 小时数据发送次数.vi" "小时数据发送次数"() -> (w1310:i32)
      n498 = global read "全局 小时数据发送次数.vi" "小时数据发送次数"() -> (w1289:i32)
      n499 = global read "全局 小时数据发送次数.vi" "小时数据发送次数"() -> (w1288:i32)
      n500 = global read "全局 小时数据发送次数.vi" "小时数据发送次数"() -> (w1287:i32)
      n501 = global read "全局 小时数据发送次数.vi" "小时数据发送次数"() -> (w1296:i32)
      n502 = global read "全局 小时数据发送次数.vi" "小时数据发送次数"() -> (w1316:i32)
      n503 = global read "全局 小时数据发送次数.vi" "小时数据发送次数"() -> (w1302:i32)
      n504 = global read "全局 小时数据发送次数.vi" "小时数据发送次数"() -> (w1314:i32)
      n505 = global read "全局 小时数据发送次数.vi" "小时数据发送次数"() -> (w1299:i32)
      n506 = global read "全局 小时数据发送次数.vi" "小时数据发送次数"() -> (w1268:i32)
      n507 = global read "全局 小时数据发送次数.vi" "小时数据发送次数"() -> (w1269:i32)
      n508 = global read "全局 小时数据发送次数.vi" "小时数据发送次数"() -> (w1277:i32)
      n509 = global read "全局 小时数据发送次数.vi" "小时数据发送次数"() -> (w1267:i32)
      n510 = global read "全局 小时数据发送次数.vi" "小时数据发送次数"() -> (w1276:i32)
      n511 = global read "全局 小时数据发送次数.vi" "小时数据发送次数"() -> (w1318:i32)
      n512 = global read "全局 小时数据发送次数.vi" "小时数据发送次数"() -> (w1278:i32)
      n513 = global read "全局 小时数据发送次数.vi" "小时数据发送次数"() -> (w1304:i32)
      n514 = global read "全局 小时数据发送次数.vi" "小时数据发送次数"() -> (w1312:i32)
      n515 = global read "全局 小时数据发送次数.vi" "小时数据发送次数"() -> (w1259:i32)
      n516 = global read "全局 小时数据发送次数.vi" "小时数据发送次数"() -> (w1258:i32)
      n517 = global read "全局 小时数据发送次数.vi" "小时数据发送次数"() -> (w1260:i32)
      n518 = global read "全局 小时数据发送次数.vi" "小时数据发送次数"() -> (w1300:i32)
      n519 = global read "全局 小时数据发送次数.vi" "小时数据发送次数"() -> (w1320:i32)
      n520 = Index Array(array=w1266, index (row)=w1269) -> (element=w1263:string[])  [unwired: 1 in]
      n521 = Index Array(array=w1275, index (row)=w1276) -> (element=w1272:string[])  [unwired: 1 in]
      n522 = Index Array(array=w1264, index (row)=w1268) -> (element=w1261:string[])  [unwired: 1 in]
      n523 = Index Array(array=w1273, index (row)=w1277) -> (element=w1270:string[])  [unwired: 1 in]
      n524 = Index Array(array=w1265, index (row)=w1267) -> (element=w1262:string[])  [unwired: 1 in]
      n525 = Index Array(array=w1274, index (row)=w1278) -> (element=w1271:string[])  [unwired: 1 in]
      n526 = Index Array(array=w1257, index (row)=w1258) -> (element=w1254:string[])  [unwired: 1 in]
      n527 = Index Array(array=w1327, index (row)=w1307) -> (element=w1308:string[])  [unwired: 1 in]
      n528 = Index Array(array=w1291, index (row)=w1294) -> (element=w1293:string[])  [unwired: 1 in]
      n529 = Index Array(array=w1282, index (row)=w1290) -> (element=w1286:string[])  [unwired: 1 in]
      n530 = Index Array(array=w1328, index (row)=w1310) -> (element=w1309:string[])  [unwired: 1 in]
      n531 = Index Array(array=w1281, index (row)=w1289) -> (element=w1285:string[])  [unwired: 1 in]
      n532 = Index Array(array=w1280, index (row)=w1288) -> (element=w1284:string[])  [unwired: 1 in]
      n533 = Index Array(array=w1279, index (row)=w1287) -> (element=w1283:string[])  [unwired: 1 in]
      n534 = Index Array(array=w1255, index (row)=w1259) -> (element=w1252:string[])  [unwired: 1 in]
      n535 = Index Array(array=w1292, index (row)=w1296) -> (element=w1295:string[])  [unwired: 1 in]
      n536 = Index Array(array=w1256, index (row)=w1260) -> (element=w1253:string[])  [unwired: 1 in]
      n537 = Index Array(array=w1332, index (row)=w1318) -> (element=w1317:string[])  [unwired: 1 in]
      n538 = Index Array(array=w1331, index (row)=w1316) -> (element=w1315:string[])  [unwired: 1 in]
      n539 = Index Array(array=w1330, index (row)=w1314) -> (element=w1313:string[])  [unwired: 1 in]
      n540 = Index Array(array=w1333, index (row)=w1320) -> (element=w1319:string[])  [unwired: 1 in]
      n541 = Index Array(array=w1326, index (row)=w1306) -> (element=w1305:string[])  [unwired: 1 in]
      n542 = Index Array(array=w1324, index (row)=w1302) -> (element=w1301:string[])  [unwired: 1 in]
      n543 = Index Array(array=w1325, index (row)=w1304) -> (element=w1303:string[])  [unwired: 1 in]
      n544 = Index Array(array=w1329, index (row)=w1312) -> (element=w1311:string[])  [unwired: 1 in]
      n545 = Index Array(array=w1322, index (row)=w1299) -> (element=w1297:string[])  [unwired: 1 in]
      n546 = Index Array(array=w1323, index (row)=w1300) -> (element=w1298:string[])  [unwired: 1 in]
      n547 = global read "全局1.vi" "枚举"() -> (w1321:enum16{"返回请求应答", "上传数据", "返回执行结果"})
      n548 = case shown="\"上传数据\"" w1321 {
        tunnel: ["QnRtn=1" w1562 "ExeRtn=1"] -> w1334
        tunnel: w1319 -> [_ w1589 _]
        tunnel: w1315 -> [_ w1603 _]
        tunnel: w1313 -> [_ w1602 _]
        tunnel: w1311 -> [_ w1601 _]
        tunnel: w1317 -> [_ w1599 _]
        tunnel: w1309 -> [_ w1588 _]
        tunnel: w1308 -> [_ w1594 _]
        tunnel: w1305 -> [_ w1591 _]
        tunnel: w1303 -> [_ w1590 _]
        tunnel: w1301 -> [_ w1587 _]
        tunnel: w1298 -> [_ w1586 _]
        tunnel: w1297 -> [_ w1585 _]
        tunnel: w1295 -> [_ w1567 _]
        tunnel: w1293 -> [_ w1566 _]
        tunnel: w1286 -> [_ w1561 _]
        tunnel: w1285 -> [_ w1560 _]
        tunnel: w1284 -> [_ w1559 _]
        tunnel: w1283 -> [_ w1558 _]
        tunnel: w1272 -> [_ w1479 _]
        tunnel: w1271 -> [_ w1478 _]
        tunnel: w1270 -> [_ w1477 _]
        tunnel: w1263 -> [_ w1379 _]
        tunnel: w1262 -> [_ w1378 _]
        tunnel: w1261 -> [_ w1377 _]
        tunnel: w1254 -> [_ w1346 _]
        tunnel: w1253 -> [_ w1345 _]
        tunnel: w1252 -> [_ w1344 _]
        frame "返回请求应答", Default {
          (unwired) 0 ("当前包数")
          n549 = global read "全局 数据数组大小.vi" "数据数组大小"() -> (w1335:i32)
          n550 = global write "全局1.vi" "枚举"(enum16{"返回请求应答", "上传数据", "返回执行结果"}."上传数据" ("枚举")) -> ()
          n551 = Equal To 0?(x=w1335) -> (x = 0?=w1336:bool)
          n552 = case shown="真" w1336 {
            frame False {
            }
            frame True {
              n553 = global read "全局 小时数据发送次数.vi" "小时数据发送次数"() -> (w1340:i32)
              n554 = Increment(x=w1340) -> (x+1=w1339:i32)
              n555 = global write "全局 小时数据发送次数.vi" "小时数据发送次数"(w1339) -> ()
            }
          }
        }
        frame "上传数据" {
          (unwired) 2 ("数据精度")
          (unwired) 3 ("数据精度")
          (unwired) 3 ("数据精度")
          (unwired) 3 ("数据精度")
          # "汞"
          # "锰"
          # "镍"
          # "锌"
          # "镉"
          # "铅"
          # "藻密度"
          # "叶绿素"
          # "浊度"
          # "电导率"
          # "DO"
          # "水温"
          # "CODMn"
          # "ORP"
          # "硫化物"
          # "亚硝酸盐"
          # "PH"
          # "总氮"
          # "总磷"
          # "CODCr"
          # "NH3"
          n556 = global read "断电保存全局.vi" "数据发送协议"() -> (w1512:enum16{"2005-212协议", "2017-212协议"})
          n557 = case shown="\"2017-212协议\", 默认" w1512 {
            tunnel: w1567 -> [_ w1729]
            tunnel: w1566 -> [_ w1728]
            tunnel: [w1683 w1727] -> w1565
            tunnel: [w1683 w1726] -> w1564
            tunnel: w1561 -> [_ w1713]
            tunnel: w1560 -> [_ w1712]
            tunnel: w1559 -> [w1675 w1711]
            tunnel: w1558 -> [_ w1710]
            tunnel: [w1683 w1709] -> w1557
            tunnel: [w1683 w1708] -> w1556
            tunnel: [w1676 w1707] -> w1555
            tunnel: [w1683 w1706] -> w1554
            frame "2005-212协议" {
              w1683 = "" ("编码输出")
              # "瞬时流量"
              n558 = Index Array(array=w1675, index #1=5 ("索引"), index #2=1 ("索引")) -> (element #2=w1681:string)  [unwired: 1 out]
              n559 = call "数据编码整合输出.vi"("数据标识"="N", "数据类型"="-Avg=", "污染物编码"="B01", "数据值"=w1681) -> ("编码输出"=w1676:string)  [unwired: 7 in]
            }
            frame "2017-212协议", Default {
              # "盐度改COD"
              # "总铜"
              n560 = Index Array(array=w1728, index #1=2 ("索引"), index #2=3 ("索引"), index #3=5 ("索引")) -> (element #1=w1700:string, element #2=w1699:string, element #3=w1684:string)
              n561 = Index Array(array=w1712, index=1 ("索引")) -> (element=w1688:string)
              n562 = Index Array(array=w1713, index=1 ("索引")) -> (element=w1689:string)
              n563 = Index Array(array=w1711, index=1 ("索引")) -> (element=w1690:string)
              n564 = Index Array(array=w1729, index #1=2 ("索引"), index #2=3 ("索引"), index #3=5 ("索引")) -> (element #1=w1703:string, element #2=w1702:string, element #3=w1686:string)
              n565 = Index Array(array=w1710, index=1 ("索引")) -> (element=w1691:string)
              n566 = case shown="\"M\"" w1703 {
                tunnel: [w1736 ""] -> w1701
                tunnel: w1702 -> [w1736 _]
                frame "N", Default {
                }
                frame "M" {
                }
              }
              n567 = case shown="\"M\"" w1700 {
                tunnel: [w1734 ""] -> w1698
                tunnel: w1699 -> [w1734 _]
                frame "N", Default {
                }
                frame "M" {
                }
              }
              n568 = call "数据编码整合输出.vi"("数据标识"="N" ("字符串"), "数据类型"="-Avg=", "污染物编码"="e01204", "数据值"=w1691) -> ("编码输出"=w1706:string)  [unwired: 7 in]
              n569 = call "数据编码整合输出.vi"("数据标识"="N" ("字符串"), "数据类型"="-Avg=", "污染物编码"="e01203", "数据值"=w1690) -> ("编码输出"=w1707:string)  [unwired: 7 in]
              n570 = call "数据编码整合输出.vi"("数据标识"=w1686, "数据类型"="-Avg=", "污染物编码"="w20122", "数据值"=w1701) -> ("编码输出"=w1727:string)  [unwired: 7 in]
              n571 = call "数据编码整合输出.vi"("数据标识"="N" ("字符串"), "数据类型"="-Avg=", "污染物编码"="e01201", "数据值"=w1689) -> ("编码输出"=w1709:string)  [unwired: 7 in]
              n572 = call "数据编码整合输出.vi"("数据标识"="N" ("字符串"), "数据类型"="-Avg=", "污染物编码"="e01202", "数据值"=w1688) -> ("编码输出"=w1708:string)  [unwired: 7 in]
              n573 = call "数据编码整合输出.vi"("数据标识"=w1684, "数据类型"="-Avg=", "污染物编码"="w01018", "数据值"=w1698) -> ("编码输出"=w1726:string)  [unwired: 7 in]
            }
          }
          n574 = Index Array(array=w1586, index #1=2 ("索引"), index #2=3 ("索引"), index #3=5 ("索引")) -> (element #1=w1422:string, element #2=w1424:string, element #3=w1409:string)
          n575 = Index Array(array=w1591, index #1=2 ("索引"), index #2=3 ("索引"), index #3=5 ("索引")) -> (element #1=w1429:string, element #2=w1430:string, element #3=w1413:string)
          n576 = Index Array(array=w1587, index #1=2 ("索引"), index #2=3 ("索引"), index #3=5 ("索引")) -> (element #1=w1427:string, element #2=w1426:string, element #3=w1411:string)
          n577 = Index Array(array=w1585, index #1=2 ("索引"), index #2=3 ("索引"), index #3=5 ("索引")) -> (element #1=w1421:string, element #2=w1420:string, element #3=w1407:string)
          n578 = Index Array(array=w1479, index #1=2 ("索引"), index #2=3 ("索引"), index #3=5 ("索引")) -> (element #1=w1490:string, element #2=w1488:string, element #3=w1492:string)
          n579 = Index Array(array=w1590, index #1=2 ("索引"), index #2=3 ("索引"), index #3=5 ("索引")) -> (element #1=w1456:string, element #2=w1457:string, element #3=w1452:string)
          n580 = Index Array(array=w1344, index #1=2 ("索引"), index #2=3 ("索引"), index #3=5 ("索引")) -> (element #1=w1371:string, element #2=w1369:string, element #3=w1373:string)
          n581 = Index Array(array=w1377, index #1=2 ("索引"), index #2=3 ("索引"), index #3=5 ("索引")) -> (element #1=w1382:string, element #2=w1384:string, element #3=w1380:string)
          n582 = Index Array(array=w1345, index #1=2 ("索引"), index #2=3 ("索引"), index #3=5 ("索引")) -> (element #1=w1358:string, element #2=w1360:string, element #3=w1356:string)
          n583 = Index Array(array=w1603, index #1=2 ("索引"), index #2=3 ("索引"), index #3=5 ("索引")) -> (element #1=w1433:string, element #2=w1432:string, element #3=w1415:string)
          n584 = Index Array(array=w1378, index #1=2 ("索引"), index #2=3 ("索引"), index #3=5 ("索引")) -> (element #1=w1395:string, element #2=w1393:string, element #3=w1397:string)
          n585 = Index Array(array=w1346, index #1=2 ("索引"), index #2=3 ("索引"), index #3=5 ("索引")) -> (element #1=w1353:string, element #2=w1351:string, element #3=w1355:string)
          n586 = Index Array(array=w1477, index #1=2 ("索引"), index #2=3 ("索引"), index #3=5 ("索引")) -> (element #1=w1502:string, element #2=w1500:string, element #3=w1504:string)
          n587 = Index Array(array=w1379, index #1=2 ("索引"), index #2=3 ("索引"), index #3=5 ("索引")) -> (element #1=w1400:string, element #2=w1402:string, element #3=w1398:string)
          n588 = Index Array(array=w1589, index #1=2 ("索引"), index #2=3 ("索引"), index #3=5 ("索引")) -> (element #1=w1465:string, element #2=w1464:string, element #3=w1461:string)
          n589 = Index Array(array=w1588, index #1=2 ("索引"), index #2=3 ("索引"), index #3=5 ("索引")) -> (element #1=w1535:string, element #2=w1534:string, element #3=w1518:string)
          n590 = Index Array(array=w1478, index #1=2 ("索引"), index #2=3 ("索引"), index #3=5 ("索引")) -> (element #1=w1497:string, element #2=w1495:string, element #3=w1506:string)
          n591 = Index Array(array=w1599, index #1=2 ("索引"), index #2=3 ("索引"), index #3=5 ("索引")) -> (element #1=w1545:string, element #2=w1547:string, element #3=w1526:string)
          n592 = Index Array(array=w1594, index #1=2 ("索引"), index #2=3 ("索引"), index #3=5 ("索引")) -> (element #1=w1543:string, element #2=w1544:string, element #3=w1524:string)
          n593 = Index Array(array=w1602, index #1=2 ("索引"), index #2=3 ("索引"), index #3=5 ("索引")) -> (element #1=w1541:string, element #2=w1540:string, element #3=w1522:string)
          n594 = global read "全局 水样时间.vi" "选择发送的参数"() -> (w1508:string)
          n595 = Index Array(array=w1601, index #1=2 ("索引"), index #2=3 ("索引"), index #3=5 ("索引")) -> (element #1=w1538:string, element #2=w1537:string, element #3=w1520:string)
          n596 = case shown="\"M\"" w1433 {
            tunnel: [w1626 ""] -> w1431
            tunnel: w1432 -> [w1626 _]
            frame "N", Default {
            }
            frame "M" {
            }
          }
          n597 = case shown="\"M\"" w1429 {
            tunnel: [w1624 ""] -> w1428
            tunnel: w1430 -> [w1624 _]
            frame "N", Default {
            }
            frame "M" {
            }
          }
          n598 = case shown="\"M\"" w1427 {
            tunnel: [w1622 ""] -> w1425
            tunnel: w1426 -> [w1622 _]
            frame "N", Default {
            }
            frame "M" {
            }
          }
          n599 = case shown="\"M\"" w1422 {
            tunnel: [w1620 ""] -> w1423
            tunnel: w1424 -> [w1620 _]
            frame "N", Default {
            }
            frame "M" {
            }
          }
          n600 = case shown="\"M\"" w1421 {
            tunnel: [w1618 ""] -> w1419
            tunnel: w1420 -> [w1618 _]
            frame "N", Default {
            }
            frame "M" {
            }
          }
          n601 = case shown="\"M\"" w1541 {
            tunnel: [w1742 ""] -> w1539
            tunnel: w1540 -> [w1742 _]
            frame "N", Default {
            }
            frame "M" {
            }
          }
          n602 = case shown="\"M\"" w1543 {
            tunnel: [w1744 ""] -> w1542
            tunnel: w1544 -> [w1744 _]
            frame "N", Default {
            }
            frame "M" {
            }
          }
          n603 = case shown="\"M\"" w1535 {
            tunnel: [w1738 ""] -> w1533
            tunnel: w1534 -> [w1738 _]
            frame "N", Default {
            }
            frame "M" {
            }
          }
          n604 = case shown="\"N\", 默认" w1490 {
            tunnel: [w1636 ""] -> w1491
            tunnel: w1488 -> [w1636 _]
            frame "N", Default {
            }
            frame "M" {
            }
          }
          n605 = case shown="\"M\"" w1538 {
            tunnel: [w1740 ""] -> w1536
            tunnel: w1537 -> [w1740 _]
            frame "N", Default {
            }
            frame "M" {
            }
          }
          n606 = case shown="\"N\", 默认" w1371 {
            tunnel: [w1606 ""] -> w1372
            tunnel: w1369 -> [w1606 _]
            frame "N", Default {
            }
            frame "M" {
            }
          }
          n607 = case shown="\"N\", 默认" w1382 {
            tunnel: [w1612 ""] -> w1381
            tunnel: w1384 -> [w1612 _]
            frame "N", Default {
            }
            frame "M" {
            }
          }
          n608 = case shown="\"N\", 默认" w1358 {
            tunnel: [w1608 ""] -> w1357
            tunnel: w1360 -> [w1608 _]
            frame "N", Default {
            }
            frame "M" {
            }
          }
          n609 = case shown="\"M\"" w1545 {
            tunnel: [w1746 ""] -> w1546
            tunnel: w1547 -> [w1746 _]
            frame "N", Default {
            }
            frame "M" {
            }
          }
          n610 = case shown="\"N\", 默认" w1395 {
            tunnel: [w1614 ""] -> w1396
            tunnel: w1393 -> [w1614 _]
            frame "N", Default {
            }
            frame "M" {
            }
          }
          n611 = case shown="\"M\"" w1465 {
            tunnel: [w1630 ""] -> w1463
            tunnel: w1464 -> [w1630 _]
            frame "N", Default {
            }
            frame "M" {
            }
          }
          n612 = case shown="\"M\"" w1456 {
            tunnel: [w1628 ""] -> w1455
            tunnel: w1457 -> [w1628 _]
            frame "N", Default {
            }
            frame "M" {
            }
          }
          n613 = case shown="\"N\", 默认" w1353 {
            tunnel: [w1610 ""] -> w1354
            tunnel: w1351 -> [w1610 _]
            frame "N", Default {
            }
            frame "M" {
            }
          }
          n614 = case shown="\"N\", 默认" w1502 {
            tunnel: [w1632 ""] -> w1503
            tunnel: w1500 -> [w1632 _]
            frame "N", Default {
            }
            frame "M" {
            }
          }
          n615 = case shown="\"N\", 默认" w1400 {
            tunnel: [w1616 ""] -> w1399
            tunnel: w1402 -> [w1616 _]
            frame "N", Default {
            }
            frame "M" {
            }
          }
          n616 = case shown="\"N\", 默认" w1497 {
            tunnel: [w1634 ""] -> w1505
            tunnel: w1495 -> [w1634 _]
            frame "N", Default {
            }
            frame "M" {
            }
          }
          n617 = case shown="\"汞\"" w1508 {
            tunnel: [w1638 w1639 w1640 w1641 w1642 w1643 w1644 w1645 w1646 w1647 w1648 w1649 w1650 w1651 w1652 w1653 w1654 w1655 w1656 w1657 w1658 w1659 w1660 w1661 w1662 w1663 w1664] -> w1507
            frame "CODMn", Default {
              n618 = global read "全局 所有参数.vi" "CODMn"() -> (w1638:string[][])
            }
            frame "CODCr" {
              n619 = global read "全局 所有参数.vi" "CODCr"() -> (w1639:string[][])
            }
            frame "DO" {
              n620 = global read "全局 所有参数.vi" "DO"() -> (w1640:string[][])
            }
            frame "铜" {
              n621 = global read "全局 所有参数.vi" "铜"() -> (w1641:string[][])
            }
            frame "PH" {
              n622 = global read "全局 所有参数.vi" "PH"() -> (w1642:string[][])
            }
            frame "氨氮" {
              n623 = global read "全局 所有参数.vi" "氨氮"() -> (w1643:string[][])
            }
            frame "比电导率", "电导率" {
              n624 = global read "全局 所有参数.vi" "电导率"() -> (w1644:string[][])
            }
            frame "水温" {
              n625 = global read "全局 所有参数.vi" "水温"() -> (w1645:string[][])
            }
            frame "COD" {
              n626 = global read "全局 所有参数.vi" "盐度"() -> (w1646:string[][])
            }
            frame "浊度" {
              n627 = global read "全局 所有参数.vi" "浊度"() -> (w1647:string[][])
            }
            frame "总氮" {
              n628 = global read "全局 所有参数.vi" "总氮"() -> (w1648:string[][])
            }
            frame "总磷" {
              n629 = global read "全局 所有参数.vi" "总磷"() -> (w1649:string[][])
            }
            frame "叶绿素a" {
              n630 = global read "全局 所有参数.vi" "叶绿素"() -> (w1650:string[][])
            }
            frame "藻密度" {
              n631 = global read "全局 所有参数.vi" "藻密度"() -> (w1651:string[][])
            }
            frame "水位" {
              n632 = global read "全局流量数据小时.vi" "水位"() -> (w1652:string[][])
            }
            frame "流速" {
              n633 = global read "全局流量数据小时.vi" "流速"() -> (w1653:string[][])
            }
            frame "瞬时流量" {
              n634 = global read "全局流量数据小时.vi" "瞬时流量"() -> (w1654:string[][])
            }
            frame "累积流量" {
              n635 = global read "全局流量数据小时.vi" "累积流量"() -> (w1655:string[][])
            }
            frame "亚硝氮" {
              n636 = global read "全局 所有参数.vi" "亚硝酸盐"() -> (w1656:string[][])
            }
            frame "硫化物" {
              n637 = global read "全局 所有参数.vi" "硫化物"() -> (w1657:string[][])
            }
            frame "ORP" {
              n638 = global read "全局 所有参数.vi" "ORP"() -> (w1658:string[][])
            }
            frame "铅" {
              n639 = global read "全局 所有参数.vi" "铅"() -> (w1659:string[][])
            }
            frame "镉" {
              n640 = global read "全局 所有参数.vi" "镉"() -> (w1660:string[][])
            }
            frame "锌" {
              n641 = global read "全局 所有参数.vi" "锌"() -> (w1661:string[][])
            }
            frame "镍" {
              n642 = global read "全局 所有参数.vi" "镍"() -> (w1662:string[][])
            }
            frame "锰" {
              n643 = global read "全局 所有参数.vi" "锰"() -> (w1663:string[][])
            }
            frame "汞" {
              n644 = global read "全局 所有参数.vi" "汞"() -> (w1664:string[][])
            }
          }
          n645 = global read "全局 小时数据发送次数.vi" "小时数据发送次数"() -> (w1552:i32)
          n646 = global read "断电保存全局.vi" "数据发送协议"() -> (w1509:enum16{"2005-212协议", "2017-212协议"})
          n647 = global read "断电保存全局.vi" "数据发送协议"() -> (w1510:enum16{"2005-212协议", "2017-212协议"})
          n648 = global read "断电保存全局.vi" "数据发送协议"() -> (w1511:enum16{"2005-212协议", "2017-212协议"})
          n649 = Index Array(array=w1507, index (row)=w1552) -> (element=w1551:string[])  [unwired: 1 in]
          n650 = Index Array(array=w1551, index=0 ("索引")) -> (element=w1549:string)
          n651 = case shown="\"2017-212协议\", 默认" w1509 {
            tunnel: ["011" ("污染物编码") "w01018" ("污染物编码")] -> w1513
            frame "2005-212协议" {
            }
            frame "2017-212协议", Default {
            }
          }
          n652 = case shown="\"2005-212协议\"" w1511 {
            tunnel: ["101" ("污染物编码") "w21011" ("污染物编码")] -> w1517
            tunnel: ["065" ("污染物编码") "w21001" ("污染物编码")] -> w1516
            tunnel: ["001" ("污染物编码") "w01001" ("污染物编码")] -> w1515
            frame "2005-212协议" {
            }
            frame "2017-212协议", Default {
            }
          }
          n653 = case shown="\"2005-212协议\"" w1510 {
            tunnel: ["060" ("污染物编码") "w21003" ("污染物编码")] -> w1514
            frame "2005-212协议" {
            }
            frame "2017-212协议", Default {
            }
          }
          n654 = call "数据编码整合输出.vi"("数据标识"=w1373, "数据类型"="-Avg=", "污染物编码"="w20111", "数据值"=w1372) -> ("编码输出"=w1341:string)  [unwired: 7 in]
          n655 = call "数据编码整合输出.vi"("数据标识"=w1380, "数据类型"="-Avg=", "污染物编码"="w20123", "数据值"=w1381) -> ("编码输出"=w1376:string)  [unwired: 7 in]
          n656 = call "数据编码整合输出.vi"("数据标识"=w1356, "数据类型"="-Avg=", "污染物编码"="w20124", "数据值"=w1357) -> ("编码输出"=w1342:string)  [unwired: 7 in]
          n657 = call "数据编码整合输出.vi"("数据标识"=w1397, "数据类型"="-Avg=", "污染物编码"="w20115", "数据值"=w1396) -> ("编码输出"=w1375:string)  [unwired: 7 in]
          n658 = call "数据编码整合输出.vi"("数据标识"=w1355, "数据类型"="-Avg=", "污染物编码"="w20121", "数据值"=w1354) -> ("编码输出"=w1343:string)  [unwired: 7 in]
          n659 = call "数据编码整合输出.vi"("数据标识"=w1504, "数据类型"="-Avg=", "污染物编码"="w01100", "数据值"=w1503) -> ("编码输出"=w1476:string)  [unwired: 7 in]
          n660 = call "数据编码整合输出.vi"("数据标识"=w1398, "数据类型"="-Avg=", "污染物编码"="w20120", "数据值"=w1399) -> ("编码输出"=w1374:string)  [unwired: 7 in]
          n661 = call "数据编码整合输出.vi"("数据标识"=w1492, "数据类型"="-Avg=", "污染物编码"="w21006", "数据值"=w1491) -> ("编码输出"=w1474:string)  [unwired: 7 in]
          n662 = call "数据编码整合输出.vi"("数据标识"=w1506, "数据类型"="-Avg=", "污染物编码"="w21019", "数据值"=w1505) -> ("编码输出"=w1475:string)  [unwired: 7 in]
          n663 = call "规范小时时间戳.vi"("字符串"=w1549) -> ("result string"=w1529:string)  [unwired: 10 in]
          n664 = call "数据编码整合输出.vi"("数据标识"=w1461, "数据类型"="-Avg=", "污染物编码"="w01019", "数据值"=w1463) -> ("编码输出"=w1584:string)  [unwired: 7 in]
          n665 = call "数据编码整合输出.vi"("数据标识"=w1452, "数据类型"="-Avg=", "污染物编码"="w01010", "数据值"=w1455) -> ("编码输出"=w1581:string)  [unwired: 7 in]
          n666 = call "数据编码整合输出.vi"("数据标识"=w1524, "数据类型"="-Avg=", "污染物编码"=w1513, "数据值"=w1542) -> ("编码输出"=w1579:string)  [unwired: 7 in]
          n667 = call "数据编码整合输出.vi"("数据标识"=w1526, "数据类型"="-Avg=", "污染物编码"=w1514, "数据值"=w1546) -> ("编码输出"=w1582:string)  [unwired: 7 in]
          n668 = call "数据编码整合输出.vi"("数据标识"=w1520, "数据类型"="-Avg=", "污染物编码"=w1516, "数据值"=w1536) -> ("编码输出"=w1570:string)  [unwired: 7 in]
          n669 = call "数据编码整合输出.vi"("数据标识"=w1518, "数据类型"="-Avg=", "污染物编码"=w1515, "数据值"=w1533) -> ("编码输出"=w1568:string)  [unwired: 7 in]
          n670 = call "数据编码整合输出.vi"("数据标识"=w1413, "数据类型"="-Avg=", "污染物编码"="w01014", "数据值"=w1428) -> ("编码输出"=w1577:string)  [unwired: 7 in]
          n671 = call "数据编码整合输出.vi"("数据标识"=w1415, "数据类型"="-Avg=", "污染物编码"="w01009", "数据值"=w1431) -> ("编码输出"=w1578:string)  [unwired: 7 in]
          n672 = call "数据编码整合输出.vi"("数据标识"=w1407, "数据类型"="-Avg=", "污染物编码"="w19011", "数据值"=w1419) -> ("编码输出"=w1574:string)  [unwired: 7 in]
          n673 = call "数据编码整合输出.vi"("数据标识"=w1411, "数据类型"="-Avg=", "污染物编码"="w01003", "数据值"=w1425) -> ("编码输出"=w1576:string)  [unwired: 7 in]
          n674 = call "数据编码整合输出.vi"("数据标识"=w1409, "数据类型"="-Avg=", "污染物编码"="w01016", "数据值"=w1423) -> ("编码输出"=w1575:string)  [unwired: 7 in]
          n675 = call "数据编码整合输出.vi"("数据标识"=w1522, "数据类型"="-Avg=", "污染物编码"=w1517, "数据值"=w1539) -> ("编码输出"=w1572:string)  [unwired: 7 in]
          n676 = Format Into String(format string="DataTime=%s;", w1529) -> (resulting string=w1532:string)  [unwired: 2 in, 1 out]
          n677 = Format Into String(format string="%s%s%s%s%s%s%s%s%s%s%s%s%s%s%s%s%s%s%s%s%s%s%s%s%s%s%s" ("格式字符串"), w1584, w1582, w1581, w1579, w1578, w1577, w1576, w1575, w1574, w1572, w1570, w1568, w1565, w1564, w1557, w1556, w1555, w1554, w1474, w1475, w1476, w1374, w1375, w1376, w1343, w1342, w1341) -> (resulting string=w1530:string)  [unwired: 2 in, 1 out]
          n678 = Empty String/Path?(string/path=w1530) -> (empty?=w1563:bool)
          n679 = Concatenate Strings(w1532, w1530) -> (w1471:string)
          n680 = String Length(string=w1471) -> (length=w1473:i32)
          n681 = Decrement(x=w1473) -> (x-1=w1472:i32)
          n682 = String Subset(string=w1471, length (rest)=w1472) -> (substring=w1470:string)  [unwired: 1 in]
          n683 = global read "全局 数据发送重叠.vi" "主动上报数据中"() -> (w1548:bool)
          n684 = case shown="假" w1563 {
            tunnel: [w1749 ""] -> w1562
            tunnel: w1470 -> [w1749 _]
            tunnel: w1548 -> [w1748 w1752]
            frame False {
              n685 = case shown="真" w1748 {
                frame False {
                  n686 = global read "全局 小时数据发送次数.vi" "小时数据发送次数"() -> (w1751:i32)
                  n687 = Increment(x=w1751) -> (x+1=w1750:i32)
                  n688 = global write "全局 小时数据发送次数.vi" "小时数据发送次数"(w1750) -> ()
                }
                frame True {
                }
              }
            }
            frame True {
              n689 = case shown="假" w1752 {
                frame False {
                  n690 = global read "全局 小时数据发送次数.vi" "小时数据发送次数"() -> (w1755:i32)
                  n691 = Increment(x=w1755) -> (x+1=w1754:i32)
                  n692 = global write "全局 小时数据发送次数.vi" "小时数据发送次数"(w1754) -> ()
                }
                frame True {
                }
              }
            }
          }
        }
        frame "返回执行结果" {
          (unwired) 0 ("当前包数")
          n693 = global write "全局1.vi" "枚举"(enum16{"返回请求应答", "上传数据", "返回执行结果"}."返回请求应答" ("枚举")) -> ()
        }
      }
    }
    frame "剖面多参数H" {
      # "发送小时数据"
      n694 = global read "全局1.vi" "枚举"() -> (w1758:enum16{"返回请求应答", "上传数据", "返回执行结果"})
      n695 = case shown="\"上传数据\"" w1758 {
        tunnel: ["QnRtn=1" w1768 "ExeRtn=1"] -> w1759
        frame "返回请求应答", Default {
          (unwired) 0 ("当前包数")
          n696 = global read "全局 数据数组大小.vi" "数据数组大小"() -> (w1760:i32)
          n697 = global write "全局1.vi" "枚举"(enum16{"返回请求应答", "上传数据", "返回执行结果"}."上传数据" ("枚举")) -> ()
          n698 = Equal To 0?(x=w1760) -> (x = 0?=w1761:bool)
          n699 = case shown="真" w1761 {
            frame False {
            }
            frame True {
              n700 = global read "全局 小时数据发送次数.vi" "小时数据发送次数"() -> (w1765:i32)
              n701 = Increment(x=w1765) -> (x+1=w1764:i32)
              n702 = global write "全局 小时数据发送次数.vi" "小时数据发送次数"(w1764) -> ()
            }
          }
        }
        frame "上传数据" {
          n703 = global read "断电保存全局.vi" "数据发送协议"() -> (w1767:enum16{"2005-212协议", "2017-212协议"})
          n704 = case shown="\"2017-212协议\", 默认" w1767 {
            tunnel: ["" ("编码输出") w1773] -> w1766
            frame "2005-212协议" {
            }
            frame "2017-212协议", Default {
              (unwired) "w01010" ("污染物编码")
              (unwired) "w01016" ("污染物编码")
              (unwired) "w01003" ("污染物编码")
              (unwired) "w01009" ("污染物编码")
              (unwired) "w01001" ("污染物编码")
              (unwired) "w01014" ("污染物编码")
              (unwired) "w01100" ("污染物编码")
              # "时间,测量模式,数据类型,数据标识,层数,Temp,SpCond,Cond,Sal,TDS,pH,pHmV,ORP,ODO%,ODOmg/L,Turb,Chla,Depth,"
              n705 = global read "全局 小时数据发送次数.vi" "小时数据发送次数"() -> (w1791:i32)
              n706 = global read "全局 所有参数.vi" "剖面多参数"() -> (w1794:string[][])
              n707 = Index Array(array=w1794, index (row)=w1791) -> (element=w1792:string[])  [unwired: 1 in]
              n708 = Index Array(array=w1792, index #1=0 ("索引")) -> (element #1=w1776:string, element #3=w1790:string, element #4=w1789:string, element #5=w1788:string, element #6=w1787:string, element #7=w1786:string, element #11=w1784:string, element #13=w1783:string, element #15=w1782:string, element #16=w1781:string, element #17=w1780:string)  [unwired: 16 in, 6 out]
              n709 = Build Array(w1787, w1786, w1784, w1783, w1782, w1781, w1780) -> (w1785:string[])
              n710 = call "剖面多参数组合(子VI).vi"("数据类型实时小时"="-Avg=", "数据值"=w1785, "层数"=w1788, "数据标识"=w1789, "数据类型"=w1790) -> ("编码输出"=w1772:string)  [unwired: 6 in]
              n711 = call "规范小时时间戳.vi"("字符串"=w1776) -> ("result string"=w1777:string)  [unwired: 10 in]
              n712 = Format Into String(format string="DataTime=%s;", w1777) -> (resulting string=w1778:string)  [unwired: 2 in, 1 out]
              n713 = Concatenate Strings(w1778, w1772) -> (w1774:string)
              n714 = Empty String/Path?(string/path=w1772) -> (empty?=w1775:bool)
              n715 = case shown="真" w1775 {
                tunnel: [w1795 ""] -> w1773
                tunnel: w1774 -> [w1795 _]
                frame False {
                }
                frame True {
                }
              }
            }
          }
          n716 = Empty String/Path?(string/path=w1766) -> (empty?=w1769:bool)
          n717 = case shown="假" w1769 {
            tunnel: [w1799 ""] -> w1768
            tunnel: w1766 -> [w1799 _]
            frame False {
              n718 = global read "全局 小时数据发送次数.vi" "小时数据发送次数"() -> (w1798:i32)
              n719 = Increment(x=w1798) -> (x+1=w1797:i32)
              n720 = global write "全局 小时数据发送次数.vi" "小时数据发送次数"(w1797) -> ()
            }
            frame True {
              n721 = global read "全局 小时数据发送次数.vi" "小时数据发送次数"() -> (w1801:i32)
              n722 = Increment(x=w1801) -> (x+1=w1800:i32)
              n723 = global write "全局 小时数据发送次数.vi" "小时数据发送次数"(w1800) -> ()
            }
          }
        }
        frame "返回执行结果" {
          (unwired) 0 ("当前包数")
          n724 = global write "全局1.vi" "枚举"(enum16{"返回请求应答", "上传数据", "返回执行结果"}."返回请求应答" ("枚举")) -> ()
        }
      }
    }
    frame "剖面多参数S" {
      # "发送实时数据"
      n725 = global read "全局1.vi" "枚举"() -> (w1805:enum16{"返回请求应答", "上传数据", "返回执行结果"})
      n726 = case shown="\"上传数据\"" w1805 {
        tunnel: ["QnRtn=1" w1815 "ExeRtn=1"] -> w1806
        frame "返回请求应答", Default {
          (unwired) 0 ("当前包数")
          n727 = global read "全局 数据数组大小.vi" "数据数组大小"() -> (w1807:i32)
          n728 = global write "全局1.vi" "枚举"(enum16{"返回请求应答", "上传数据", "返回执行结果"}."上传数据" ("枚举")) -> ()
          n729 = Equal To 0?(x=w1807) -> (x = 0?=w1808:bool)
          n730 = case shown="真" w1808 {
            frame False {
            }
            frame True {
              n731 = global read "全局 小时数据发送次数.vi" "小时数据发送次数"() -> (w1812:i32)
              n732 = Increment(x=w1812) -> (x+1=w1811:i32)
              n733 = global write "全局 小时数据发送次数.vi" "小时数据发送次数"(w1811) -> ()
            }
          }
        }
        frame "上传数据" {
          n734 = global read "断电保存全局.vi" "数据发送协议"() -> (w1814:enum16{"2005-212协议", "2017-212协议"})
          n735 = case shown="\"2017-212协议\", 默认" w1814 {
            tunnel: ["" ("编码输出") w1822] -> w1813
            frame "2005-212协议" {
            }
            frame "2017-212协议", Default {
              (unwired) "w01010" ("污染物编码")
              (unwired) "w01016" ("污染物编码")
              (unwired) "w01003" ("污染物编码")
              (unwired) "w01009" ("污染物编码")
              (unwired) "w01001" ("污染物编码")
              (unwired) "w01014" ("污染物编码")
              (unwired) "w01100" ("污染物编码")
              # "时间,测量模式,数据类型,数据标识,层数,Temp,SpCond,Cond,Sal,TDS,pH,pHmV,ORP,ODO%,ODOmg/L,Turb,Chla,Depth,"
              n736 = global read "全局 小时数据发送次数.vi" "小时数据发送次数"() -> (w1838:i32)
              n737 = global read "全局 所有参数.vi" "剖面多参数"() -> (w1841:string[][])
              n738 = Index Array(array=w1841, index (row)=w1838) -> (element=w1839:string[])  [unwired: 1 in]
              n739 = Index Array(array=w1839, index #1=0 ("索引")) -> (element #1=w1819:string, element #3=w1837:string, element #4=w1836:string, element #5=w1835:string, element #6=w1834:string, element #7=w1833:string, element #11=w1831:string, element #13=w1830:string, element #15=w1829:string, element #16=w1828:string, element #17=w1827:string)  [unwired: 16 in, 6 out]
              n740 = Build Array(w1834, w1833, w1831, w1830, w1829, w1828, w1827) -> (w1832:string[])
              n741 = call "剖面多参数组合(子VI).vi"("数据类型实时小时"="-Rtd=", "数据值"=w1832, "层数"=w1835, "数据标识"=w1836, "数据类型"=w1837) -> ("编码输出"=w1821:string)  [unwired: 6 in]
              n742 = call "规范时间戳.vi"("字符串"=w1819) -> ("result string"=w1818:string)  [unwired: 10 in]
              n743 = Format Into String(format string="DataTime=%s;", w1818) -> (resulting string=w1825:string)  [unwired: 2 in, 1 out]
              n744 = Concatenate Strings(w1825, w1821) -> (w1823:string)
              n745 = Empty String/Path?(string/path=w1821) -> (empty?=w1824:bool)
              n746 = case shown="假" w1824 {
                tunnel: [w1842 ""] -> w1822
                tunnel: w1823 -> [w1842 _]
                frame False {
                }
                frame True {
                }
              }
            }
          }
          n747 = Empty String/Path?(string/path=w1813) -> (empty?=w1816:bool)
          n748 = case shown="假" w1816 {
            tunnel: [w1846 ""] -> w1815
            tunnel: w1813 -> [w1846 _]
            frame False {
              n749 = global read "全局 小时数据发送次数.vi" "小时数据发送次数"() -> (w1845:i32)
              n750 = Increment(x=w1845) -> (x+1=w1844:i32)
              n751 = global write "全局 小时数据发送次数.vi" "小时数据发送次数"(w1844) -> ()
            }
            frame True {
              n752 = global read "全局 小时数据发送次数.vi" "小时数据发送次数"() -> (w1848:i32)
              n753 = Increment(x=w1848) -> (x+1=w1847:i32)
              n754 = global write "全局 小时数据发送次数.vi" "小时数据发送次数"(w1847) -> ()
            }
          }
        }
        frame "返回执行结果" {
          (unwired) 0 ("当前包数")
          n755 = global write "全局1.vi" "枚举"(enum16{"返回请求应答", "上传数据", "返回执行结果"}."返回请求应答" ("枚举")) -> ()
        }
      }
    }
    frame "提取小时数据" {
      # "藻密度"
      # "叶绿素"
      # "浊度"
      # "水温"
      # "发送小时数据"
      n756 = global read "全局 小时数据发送次数.vi" "小时数据发送次数"() -> (w1867:i32)
      n757 = global read "全局 小时数据发送次数.vi" "小时数据发送次数"() -> (w1868:i32)
      n758 = global read "全局 小时数据发送次数.vi" "小时数据发送次数"() -> (w1855:i32)
      n759 = global read "全局 小时数据发送次数.vi" "小时数据发送次数"() -> (w1871:i32)
      n760 = global read "全局 小时数据发送次数.vi" "小时数据发送次数"() -> (w1857:i32)
      n761 = global read "全局 小时数据发送次数.vi" "小时数据发送次数"() -> (w1877:i32)
      n762 = global read "全局 小时数据发送次数.vi" "小时数据发送次数"() -> (w1863:i32)
      n763 = global read "全局 小时数据发送次数.vi" "小时数据发送次数"() -> (w1875:i32)
      n764 = global read "全局 小时数据发送次数.vi" "小时数据发送次数"() -> (w1860:i32)
      n765 = global read "全局 小时数据发送次数.vi" "小时数据发送次数"() -> (w1879:i32)
      n766 = global read "全局 小时数据发送次数.vi" "小时数据发送次数"() -> (w1865:i32)
      n767 = global read "全局 小时数据发送次数.vi" "小时数据发送次数"() -> (w1873:i32)
      n768 = global read "全局 小时数据发送次数.vi" "小时数据发送次数"() -> (w1861:i32)
      n769 = global read "全局 小时数据发送次数.vi" "小时数据发送次数"() -> (w1881:i32)
      n770 = Index Array(array=w1888, index (row)=w1868) -> (element=w1869:string[])  [unwired: 1 in]
      n771 = Index Array(array=w1852, index (row)=w1855) -> (element=w1854:string[])  [unwired: 1 in]
      n772 = Index Array(array=w1889, index (row)=w1871) -> (element=w1870:string[])  [unwired: 1 in]
      n773 = Index Array(array=w1853, index (row)=w1857) -> (element=w1856:string[])  [unwired: 1 in]
      n774 = Index Array(array=w1893, index (row)=w1879) -> (element=w1878:string[])  [unwired: 1 in]
      n775 = Index Array(array=w1892, index (row)=w1877) -> (element=w1876:string[])  [unwired: 1 in]
      n776 = Index Array(array=w1891, index (row)=w1875) -> (element=w1874:string[])  [unwired: 1 in]
      n777 = Index Array(array=w1894, index (row)=w1881) -> (element=w1880:string[])  [unwired: 1 in]
      n778 = Index Array(array=w1887, index (row)=w1867) -> (element=w1866:string[])  [unwired: 1 in]
      n779 = Index Array(array=w1885, index (row)=w1863) -> (element=w1862:string[])  [unwired: 1 in]
      n780 = Index Array(array=w1886, index (row)=w1865) -> (element=w1864:string[])  [unwired: 1 in]
      n781 = Index Array(array=w1890, index (row)=w1873) -> (element=w1872:string[])  [unwired: 1 in]
      n782 = Index Array(array=w1883, index (row)=w1860) -> (element=w1858:string[])  [unwired: 1 in]
      n783 = Index Array(array=w1884, index (row)=w1861) -> (element=w1859:string[])  [unwired: 1 in]
      n784 = global read "全局1.vi" "枚举"() -> (w1882:enum16{"返回请求应答", "上传数据", "返回执行结果"})
      n785 = case shown="\"上传数据\"" w1882 {
        tunnel: ["QnRtn=1" w1930 "ExeRtn=1"] -> w1895
        tunnel: w1880 -> [_ w1994 _]
        tunnel: w1876 -> [_ w2007 _]
        tunnel: w1874 -> [_ w2006 _]
        tunnel: w1872 -> [_ w2005 _]
        tunnel: w1878 -> [_ w2004 _]
        tunnel: w1870 -> [_ w1993 _]
        tunnel: w1869 -> [_ w1998 _]
        tunnel: w1866 -> [_ w1996 _]
        tunnel: w1864 -> [_ w1995 _]
        tunnel: w1862 -> [_ w1992 _]
        tunnel: w1859 -> [_ w1991 _]
        tunnel: w1858 -> [_ w1990 _]
        tunnel: w1856 -> [_ w1935 _]
        tunnel: w1854 -> [_ w1934 _]
        frame "返回请求应答", Default {
          n786 = global read "全局 数据数组大小.vi" "数据数组大小"() -> (w1896:i32)
          n787 = Equal To 0?(x=w1896) -> (x = 0?=w1897:bool)
          n788 = case shown="真" w1897 {
            frame False {
            }
            frame True {
              n789 = global read "全局 小时数据发送次数.vi" "小时数据发送次数"() -> (w1900:i32)
              n790 = Increment(x=w1900) -> (x+1=w1899:i32)
              n791 = global write "全局 小时数据发送次数.vi" "小时数据发送次数"(w1899) -> ()
            }
          }
        }
        frame "上传数据" {
          (unwired) 2 ("数据精度")
          (unwired) 3 ("数据精度")
          (unwired) 3 ("数据精度")
          (unwired) 3 ("数据精度")
          (unwired) 3 ("数据精度")
          # "盐度"
          # "总铜"
          # "PH"
          # "总氮"
          # "总磷"
          # "藻密度"
          # "叶绿素"
          # "浊度"
          # "电导率"
          # "DO"
          # "CODCr"
          # "水温"
          # "NH3"
          # "CODMn"
          n792 = Index Array(array=w1991, index #2=1 ("索引")) -> (element #2=w1916:string)  [unwired: 1 in, 1 out]
          n793 = Index Array(array=w1996, index #2=1 ("索引")) -> (element #2=w1918:string)  [unwired: 1 in, 1 out]
          n794 = Index Array(array=w1992, index #2=1 ("索引")) -> (element #2=w1917:string)  [unwired: 1 in, 1 out]
          n795 = Index Array(array=w1990, index #2=1 ("索引")) -> (element #2=w1915:string)  [unwired: 1 in, 1 out]
          n796 = Index Array(array=w1995, index #2=1 ("索引")) -> (element #2=w1921:string)  [unwired: 1 in, 1 out]
          n797 = Index Array(array=w2007, index #2=1 ("索引")) -> (element #2=w1919:string)  [unwired: 1 in, 1 out]
          n798 = Index Array(array=w1994, index #2=1 ("索引")) -> (element #1=w1904:string, element #2=w1923:string)  [unwired: 1 in]
          n799 = Index Array(array=w1993, index #2=1 ("索引")) -> (element #2=w1912:string)  [unwired: 1 in, 1 out]
          n800 = Index Array(array=w1934, index #2=1 ("索引")) -> (element #2=w1910:string)  [unwired: 1 in, 1 out]
          n801 = Index Array(array=w1935, index #2=1 ("索引")) -> (element #2=w1911:string)  [unwired: 1 in, 1 out]
          n802 = Index Array(array=w2004, index #2=1 ("索引")) -> (element #2=w1922:string)  [unwired: 1 in, 1 out]
          n803 = Index Array(array=w1998, index #2=1 ("索引")) -> (element #2=w1920:string)  [unwired: 1 in, 1 out]
          n804 = Index Array(array=w2006, index #2=1 ("索引")) -> (element #2=w1914:string)  [unwired: 1 in, 1 out]
          n805 = Index Array(array=w2005, index #2=1 ("索引")) -> (element #2=w1913:string)  [unwired: 1 in, 1 out]
          n806 = call "规范小时时间戳.vi"("字符串"=w1904) -> ("result string"=w1905:string)  [unwired: 10 in]
          n807 = call "数据编码整合输出.vi"("数据标识"="N" ("字符串"), "数据类型"="-Avg=", "污染物编码"="w01019", "数据值"=w1923) -> ("编码输出"=w1989:string)  [unwired: 7 in]
          n808 = call "数据编码整合输出.vi"("数据标识"="N" ("字符串"), "数据类型"="-Avg=", "污染物编码"="w01010", "数据值"=w1921) -> ("编码输出"=w1978:string)  [unwired: 7 in]
          n809 = call "数据编码整合输出.vi"("数据标识"="N" ("字符串"), "数据类型"="-Avg=", "污染物编码"="w01018", "数据值"=w1920) -> ("编码输出"=w1974:string)  [unwired: 7 in]
          n810 = call "数据编码整合输出.vi"("数据标识"="N" ("字符串"), "数据类型"="-Avg=", "污染物编码"="w21003", "数据值"=w1922) -> ("编码输出"=w1982:string)  [unwired: 7 in]
          n811 = call "数据编码整合输出.vi"("数据标识"="N" ("字符串"), "数据类型"="-Avg=", "污染物编码"="w20122", "数据值"=w1911) -> ("编码输出"=w1933:string)  [unwired: 7 in]
          n812 = call "数据编码整合输出.vi"("数据标识"="N" ("字符串"), "数据类型"="-Avg=", "污染物编码"="w21001", "数据值"=w1913) -> ("编码输出"=w1946:string)  [unwired: 7 in]
          n813 = call "数据编码整合输出.vi"("数据标识"="N" ("字符串"), "数据类型"="-Avg=", "污染物编码"="w01001", "数据值"=w1912) -> ("编码输出"=w1942:string)  [unwired: 7 in]
          n814 = call "数据编码整合输出.vi"("数据标识"="N" ("字符串"), "数据类型"="-Avg=", "污染物编码"="w01015", "数据值"=w1910) -> ("编码输出"=w1932:string)  [unwired: 7 in]
          n815 = call "数据编码整合输出.vi"("数据标识"="N" ("字符串"), "数据类型"="-Avg=", "污染物编码"="w01014", "数据值"=w1918) -> ("编码输出"=w1966:string)  [unwired: 7 in]
          n816 = call "数据编码整合输出.vi"("数据标识"="N" ("字符串"), "数据类型"="-Avg=", "污染物编码"="w01009", "数据值"=w1919) -> ("编码输出"=w1970:string)  [unwired: 7 in]
          n817 = call "数据编码整合输出.vi"("数据标识"="N" ("字符串"), "数据类型"="-Avg=", "污染物编码"="w19011", "数据值"=w1915) -> ("编码输出"=w1954:string)  [unwired: 7 in]
          n818 = call "数据编码整合输出.vi"("数据标识"="N" ("字符串"), "数据类型"="-Avg=", "污染物编码"="w01003", "数据值"=w1917) -> ("编码输出"=w1962:string)  [unwired: 7 in]
          n819 = call "数据编码整合输出.vi"("数据标识"="N" ("字符串"), "数据类型"="-Avg=", "污染物编码"="w01016", "数据值"=w1916) -> ("编码输出"=w1958:string)  [unwired: 7 in]
          n820 = call "数据编码整合输出.vi"("数据标识"="N" ("字符串"), "数据类型"="-Avg=", "污染物编码"="w21011", "数据值"=w1914) -> ("编码输出"=w1950:string)  [unwired: 7 in]
          n821 = Format Into String(format string="DataTime=%s;", w1905) -> (resulting string=w1909:string)  [unwired: 2 in, 1 out]
          n822 = Format Into String(format string="%s%s%s%s%s%s%s%s%s%s%s%s%s%s" ("格式字符串"), w1989, w1982, w1978, w1974, w1970, w1966, w1962, w1958, w1954, w1950, w1946, w1942, w1933, w1932) -> (resulting string=w1907:string)  [unwired: 2 in, 1 out]
          n823 = Empty String/Path?(string/path=w1907) -> (empty?=w1931:bool)
          n824 = Concatenate Strings(w1909, w1907) -> (w1906:string)
          n825 = case shown="假" w1931 {
            tunnel: [w2010 ""] -> w1930
            tunnel: w1906 -> [w2010 _]
            frame False {
              n826 = global read "全局 小时数据发送次数.vi" "小时数据发送次数"() -> (w2009:i32)
              n827 = Increment(x=w2009) -> (x+1=w2008:i32)
              n828 = global write "全局 小时数据发送次数.vi" "小时数据发送次数"(w2008) -> ()
            }
            frame True {
              n829 = global read "全局 小时数据发送次数.vi" "小时数据发送次数"() -> (w2012:i32)
              n830 = Increment(x=w2012) -> (x+1=w2011:i32)
              n831 = global write "全局 小时数据发送次数.vi" "小时数据发送次数"(w2011) -> ()
            }
          }
        }
        frame "返回执行结果" {
        }
      }
    }
    frame "提取实时数据" {
      # "叶绿素"
      # "浊度"
      # "电导率"
      # "提取实时数据"
      n832 = global read "全局 小时数据发送次数.vi" "小时数据发送次数"() -> (w2019:i32)
      n833 = global read "全局 小时数据发送次数.vi" "小时数据发送次数"() -> (w2020:i32)
      n834 = global read "全局 小时数据发送次数.vi" "小时数据发送次数"() -> (w2034:i32)
      n835 = global read "全局 小时数据发送次数.vi" "小时数据发送次数"() -> (w2030:i32)
      n836 = global read "全局 小时数据发送次数.vi" "小时数据发送次数"() -> (w2024:i32)
      n837 = global read "全局 小时数据发送次数.vi" "小时数据发送次数"() -> (w2042:i32)
      n838 = global read "全局 小时数据发送次数.vi" "小时数据发送次数"() -> (w2044:i32)
      n839 = global read "全局 小时数据发送次数.vi" "小时数据发送次数"() -> (w2038:i32)
      n840 = global read "全局 小时数据发送次数.vi" "小时数据发送次数"() -> (w2026:i32)
      n841 = global read "全局 小时数据发送次数.vi" "小时数据发送次数"() -> (w2040:i32)
      n842 = global read "全局 小时数据发送次数.vi" "小时数据发送次数"() -> (w2023:i32)
      n843 = global read "全局 小时数据发送次数.vi" "小时数据发送次数"() -> (w2028:i32)
      n844 = global read "全局 小时数据发送次数.vi" "小时数据发送次数"() -> (w2036:i32)
      n845 = global read "全局 小时数据发送次数.vi" "小时数据发送次数"() -> (w2031:i32)
      n846 = Index Array(array=w2017, index (row)=w2019) -> (element=w2015:string[])  [unwired: 1 in]
      n847 = Index Array(array=w2018, index (row)=w2020) -> (element=w2016:string[])  [unwired: 1 in]
      n848 = Index Array(array=w2053, index (row)=w2034) -> (element=w2033:string[])  [unwired: 1 in]
      n849 = Index Array(array=w2058, index (row)=w2044) -> (element=w2043:string[])  [unwired: 1 in]
      n850 = Index Array(array=w2057, index (row)=w2042) -> (element=w2041:string[])  [unwired: 1 in]
      n851 = Index Array(array=w2050, index (row)=w2028) -> (element=w2027:string[])  [unwired: 1 in]
      n852 = Index Array(array=w2052, index (row)=w2031) -> (element=w2032:string[])  [unwired: 1 in]
      n853 = Index Array(array=w2056, index (row)=w2040) -> (element=w2039:string[])  [unwired: 1 in]
      n854 = Index Array(array=w2051, index (row)=w2030) -> (element=w2029:string[])  [unwired: 1 in]
      n855 = Index Array(array=w2055, index (row)=w2038) -> (element=w2037:string[])  [unwired: 1 in]
      n856 = Index Array(array=w2049, index (row)=w2026) -> (element=w2025:string[])  [unwired: 1 in]
      n857 = Index Array(array=w2048, index (row)=w2024) -> (element=w2022:string[])  [unwired: 1 in]
      n858 = Index Array(array=w2054, index (row)=w2036) -> (element=w2035:string[])  [unwired: 1 in]
      n859 = Index Array(array=w2047, index (row)=w2023) -> (element=w2021:string[])  [unwired: 1 in]
      n860 = global read "全局1.vi" "枚举"() -> (w2045:enum16{"返回请求应答", "上传数据", "返回执行结果"})
      n861 = case shown="\"上传数据\"" w2045 {
        tunnel: ["QnRtn=1" w2065 "ExeRtn=1"] -> w2046
        tunnel: w2043 -> [_ w2167 _]
        tunnel: w2039 -> [_ w2182 _]
        tunnel: w2037 -> [_ w2181 _]
        tunnel: w2035 -> [_ w2180 _]
        tunnel: w2041 -> [_ w2178 _]
        tunnel: w2033 -> [_ w2166 _]
        tunnel: w2032 -> [_ w2172 _]
        tunnel: w2029 -> [_ w2169 _]
        tunnel: w2027 -> [_ w2168 _]
        tunnel: w2025 -> [_ w2165 _]
        tunnel: w2022 -> [_ w2164 _]
        tunnel: w2021 -> [_ w2163 _]
        tunnel: w2016 -> [_ w2079 _]
        tunnel: w2015 -> [_ w2078 _]
        frame "返回请求应答", Default {
          n862 = global read "全局 数据数组大小.vi" "数据数组大小"() -> (w2059:i32)
          n863 = Equal To 0?(x=w2059) -> (x = 0?=w2060:bool)
          n864 = case shown="假" w2060 {
            frame False {
            }
            frame True {
              n865 = global read "全局 小时数据发送次数.vi" "小时数据发送次数"() -> (w2063:i32)
              n866 = Increment(x=w2063) -> (x+1=w2062:i32)
              n867 = global write "全局 小时数据发送次数.vi" "小时数据发送次数"(w2062) -> ()
            }
          }
        }
        frame "上传数据" {
          (unwired) 2 ("数据精度")
          (unwired) 3 ("数据精度")
          (unwired) 3 ("数据精度")
          (unwired) "-Rtd=" ("数据类型")
          (unwired) 3 ("数据精度")
          (unwired) 3 ("精度")
          # "盐度"
          # "总铜"
          # "PH"
          # "总氮"
          # "总磷"
          # "藻密度"
          # "叶绿素"
          # "浊度"
          # "电导率"
          # "DO"
          # "CODCr"
          # "水温"
          # "NH3"
          # "CODMn"
          n868 = Index Array(array=w2078, index #2=3 ("索引"), index #3=5 ("索引")) -> (element #2=w2071:string, element #3=w2070:string)  [unwired: 1 in, 1 out]
          n869 = Index Array(array=w2079, index #2=3 ("索引"), index #3=5 ("索引")) -> (element #2=w2073:string, element #3=w2072:string)  [unwired: 1 in, 1 out]
          n870 = Index Array(array=w2166, index #2=3 ("索引"), index #3=5 ("索引")) -> (element #2=w2086:string, element #3=w2087:string)  [unwired: 1 in, 1 out]
          n871 = Index Array(array=w2180, index #1=0 ("索引"), index #2=3 ("索引"), index #3=5 ("索引")) -> (element #2=w2089:string, element #3=w2090:string)  [unwired: 1 out]
          n872 = Index Array(array=w2164, index #2=3 ("索引"), index #3=5 ("索引")) -> (element #2=w2098:string, element #3=w2099:string)  [unwired: 1 in, 1 out]
          n873 = Index Array(array=w2163, index #2=3 ("索引"), index #3=5 ("索引")) -> (element #2=w2095:string, element #3=w2096:string)  [unwired: 1 in, 1 out]
          n874 = Index Array(array=w2168, index #2=3 ("索引"), index #3=5 ("索引")) -> (element #2=w2131:string, element #3=w2132:string)  [unwired: 1 in, 1 out]
          n875 = Index Array(array=w2169, index #2=3 ("索引"), index #3=5 ("索引")) -> (element #2=w2116:string, element #3=w2117:string)  [unwired: 1 in, 1 out]
          n876 = Index Array(array=w2165, index #2=3 ("索引"), index #3=5 ("索引")) -> (element #2=w2102:string, element #3=w2103:string)  [unwired: 1 in, 1 out]
          n877 = Index Array(array=w2181, index #1=0 ("索引"), index #2=3 ("索引"), index #3=5 ("索引")) -> (element #2=w2092:string, element #3=w2093:string)  [unwired: 1 out]
          n878 = Index Array(array=w2167, index #1=0 ("索引"), index #2=3 ("索引"), index #3=5 ("索引")) -> (element #1=w2085:string, element #2=w2141:string, element #3=w2140:string)
          n879 = Index Array(array=w2178, index #1=0 ("索引"), index #2=3 ("索引"), index #3=5 ("索引")) -> (element #2=w2134:string, element #3=w2135:string)  [unwired: 1 out]
          n880 = Index Array(array=w2172, index #1=0 ("索引"), index #2=3 ("索引"), index #3=5 ("索引")) -> (element #2=w2122:string, element #3=w2123:string)  [unwired: 1 out]
          n881 = Index Array(array=w2182, index #1=0 ("索引"), index #2=3 ("索引"), index #3=5 ("索引")) -> (element #2=w2119:string, element #3=w2120:string)  [unwired: 1 out]
          n882 = call "规范时间戳.vi"("字符串"=w2085) -> ("result string"=w2084:string)  [unwired: 10 in]
          n883 = call "数据编码整合输出.vi"("数据标识"=w2071, "数据类型"="-Rtd=", "污染物编码"="w01015", "数据值"=w2070) -> ("编码输出"=w2068:string)  [unwired: 7 in]
          n884 = call "数据编码整合输出.vi"("数据标识"=w2073, "数据类型"="-Rtd=", "污染物编码"="w20122", "数据值"=w2072) -> ("编码输出"=w2069:string)  [unwired: 7 in]
          n885 = call "数据编码整合输出.vi"("数据标识"=w2087, "数据类型"="-Rtd=", "污染物编码"="w01001", "数据值"=w2086) -> ("编码输出"=w2088:string)  [unwired: 7 in]
          n886 = call "数据编码整合输出.vi"("数据标识"=w2140, "数据类型"="-Rtd=", "污染物编码"="w01019", "数据值"=w2141) -> ("编码输出"=w2139:string)  [unwired: 7 in]
          n887 = call "数据编码整合输出.vi"("数据标识"=w2135, "数据类型"="-Rtd=", "污染物编码"="w21003", "数据值"=w2134) -> ("编码输出"=w2133:string)  [unwired: 7 in]
          n888 = call "数据编码整合输出.vi"("数据标识"=w2090, "数据类型"="-Rtd=", "污染物编码"="w21001", "数据值"=w2089) -> ("编码输出"=w2091:string)  [unwired: 7 in]
          n889 = call "数据编码整合输出.vi"("数据标识"=w2099, "数据类型"="-Rtd=", "污染物编码"="w01016", "数据值"=w2098) -> ("编码输出"=w2100:string)  [unwired: 7 in]
          n890 = call "数据编码整合输出.vi"("数据标识"=w2096, "数据类型"="-Rtd=", "污染物编码"="w19011", "数据值"=w2095) -> ("编码输出"=w2097:string)  [unwired: 7 in]
          n891 = call "数据编码整合输出.vi"("数据标识"=w2093, "污染物编码"="w21011", "数据值"=w2092) -> ("编码输出"=w2094:string)  [unwired: 8 in]
          n892 = call "数据编码整合输出.vi"("数据标识"=w2123, "数据类型"="-Rtd=", "污染物编码"="w01018", "数据值"=w2122) -> ("编码输出"=w2121:string)  [unwired: 7 in]
          n893 = call "数据编码整合输出.vi"("数据标识"=w2132, "数据类型"="-Rtd=", "污染物编码"="w01010", "数据值"=w2131) -> ("编码输出"=w2130:string)  [unwired: 7 in]
          n894 = call "数据编码整合输出.vi"("数据标识"=w2103, "数据类型"="-Rtd=", "污染物编码"="w01003", "数据值"=w2102) -> ("编码输出"=w2101:string)  [unwired: 7 in]
          n895 = call "数据编码整合输出.vi"("数据标识"=w2117, "数据类型"="-Rtd=", "污染物编码"="w01014", "数据值"=w2116) -> ("编码输出"=w2115:string)  [unwired: 7 in]
          n896 = call "数据编码整合输出.vi"("数据标识"=w2120, "数据类型"="-Rtd=", "污染物编码"="w01009", "数据值"=w2119) -> ("编码输出"=w2118:string)  [unwired: 7 in]
          n897 = Empty String/Path?(string/path=w2084) -> (empty?=w2067:bool)
          n898 = Format Into String(format string="DataTime=%s;%s%s%s%s%s%s%s%s%s%s%s%s%s%s" ("格式字符串"), w2084, w2139, w2133, w2130, w2121, w2118, w2115, w2101, w2100, w2097, w2094, w2091, w2088, w2069, w2068) -> (resulting string=w2066:string)  [unwired: 2 in, 1 out]
          n899 = case shown="真" w2067 {
            tunnel: [w2187 ""] -> w2065
            tunnel: w2066 -> [w2187 _]
            frame False {
              n900 = global read "全局 小时数据发送次数.vi" "小时数据发送次数"() -> (w2189:i32)
              n901 = Increment(x=w2189) -> (x+1=w2188:i32)
              n902 = global write "全局 小时数据发送次数.vi" "小时数据发送次数"(w2188) -> ()
            }
            frame True {
              n903 = global read "全局 小时数据发送次数.vi" "小时数据发送次数"() -> (w2191:i32)
              n904 = Increment(x=w2191) -> (x+1=w2190:i32)
              n905 = global write "全局 小时数据发送次数.vi" "小时数据发送次数"(w2190) -> ()
            }
          }
        }
        frame "返回执行结果" {
        }
      }
    }
    frame "核查数据" {
      # "提取标样核查数据"
      n906 = global read "全局 小时数据发送次数.vi" "小时数据发送次数"() -> (w2196:i32)
      n907 = global read "全局 小时数据发送次数.vi" "小时数据发送次数"() -> (w2213:i32)
      n908 = global read "全局 小时数据发送次数.vi" "小时数据发送次数"() -> (w2215:i32)
      n909 = global read "全局 小时数据发送次数.vi" "小时数据发送次数"() -> (w2211:i32)
      n910 = global read "全局 小时数据发送次数.vi" "小时数据发送次数"() -> (w2207:i32)
      n911 = global read "全局 小时数据发送次数.vi" "小时数据发送次数"() -> (w2199:i32)
      n912 = global read "全局 小时数据发送次数.vi" "小时数据发送次数"() -> (w2205:i32)
      n913 = global read "全局 小时数据发送次数.vi" "小时数据发送次数"() -> (w2202:i32)
      n914 = global read "全局 小时数据发送次数.vi" "小时数据发送次数"() -> (w2209:i32)
      n915 = Index Array(array=w2194, index (row)=w2196) -> (element=w2195:string[])  [unwired: 1 in]
      n916 = Index Array(array=w2221, index (row)=w2213) -> (element=w2212:string[])  [unwired: 1 in]
      n917 = Index Array(array=w2222, index (row)=w2215) -> (element=w2214:string[])  [unwired: 1 in]
      n918 = Index Array(array=w2220, index (row)=w2211) -> (element=w2210:string[])  [unwired: 1 in]
      n919 = Index Array(array=w2217, index (row)=w2207) -> (element=w2206:string[])  [unwired: 1 in]
      n920 = Index Array(array=w2197, index (row)=w2199) -> (element=w2198:string[])  [unwired: 1 in]
      n921 = Index Array(array=w2204, index (row)=w2205) -> (element=w2203:string[])  [unwired: 1 in]
      n922 = Index Array(array=w2200, index (row)=w2202) -> (element=w2201:string[])  [unwired: 1 in]
      n923 = Index Array(array=w2219, index (row)=w2209) -> (element=w2208:string[])  [unwired: 1 in]
      n924 = global read "全局1.vi" "枚举"() -> (w2216:enum16{"返回请求应答", "上传数据", "返回执行结果"})
      n925 = case shown="\"上传数据\"" w2216 {
        tunnel: ["QnRtn=1" w2273 "ExeRtn=1"] -> w2218
        tunnel: w2214 -> [_ w2293 _]
        tunnel: w2210 -> [_ w2292 _]
        tunnel: w2208 -> [_ w2291 _]
        tunnel: w2212 -> [_ w2289 _]
        tunnel: w2206 -> [_ w2277 _]
        tunnel: w2203 -> [_ w2252 _]
        tunnel: w2201 -> [_ w2244 _]
        tunnel: w2198 -> [_ w2240 _]
        tunnel: w2195 -> [_ w2232 _]
        frame "返回请求应答", Default {
          n926 = global read "全局 数据数组大小.vi" "数据数组大小"() -> (w2224:i32)
          n927 = Equal To 0?(x=w2224) -> (x = 0?=w2223:bool)
          n928 = case shown="真" w2223 {
            frame False {
            }
            frame True {
              n929 = global read "全局 小时数据发送次数.vi" "小时数据发送次数"() -> (w2227:i32)
              n930 = Increment(x=w2227) -> (x+1=w2226:i32)
              n931 = global write "全局 小时数据发送次数.vi" "小时数据发送次数"(w2226) -> ()
            }
          }
        }
        frame "上传数据" {
          # "将非空数组的时间戳写入"
          n932 = Index Array(array=w2232, index #1=0 ("索引"), index #2=3 ("索引"), index #3=7 ("索引")) -> (element #2=w2233:string, element #3=w2234:string)  [unwired: 1 out]
          n933 = Index Array(array=w2240, index #1=0 ("索引"), index #2=3 ("索引"), index #3=7 ("索引")) -> (element #2=w2239:string, element #3=w2238:string)  [unwired: 1 out]
          n934 = Index Array(array=w2252, index #1=0 ("索引"), index #2=3 ("索引"), index #3=7 ("索引")) -> (element #2=w2251:string, element #3=w2250:string)  [unwired: 1 out]
          n935 = Index Array(array=w2244, index #1=0 ("索引"), index #2=3 ("索引"), index #3=7 ("索引")) -> (element #2=w2245:string, element #3=w2246:string)  [unwired: 1 out]
          n936 = Index Array(array=w2291, index #1=0 ("索引"), index #2=3 ("索引"), index #3=7 ("索引")) -> (element #2=w2261:string, element #3=w2260:string)  [unwired: 1 out]
          n937 = Index Array(array=w2289, index #1=0 ("索引"), index #2=3 ("索引"), index #3=7 ("索引")) -> (element #1=w2272:string, element #2=w2267:string, element #3=w2266:string)
          n938 = Index Array(array=w2293, index #1=0 ("索引"), index #2=3 ("索引"), index #3=7 ("索引")) -> (element #2=w2270:string, element #3=w2269:string)  [unwired: 1 out]
          n939 = Index Array(array=w2292, index #1=0 ("索引"), index #2=3 ("索引"), index #3=7 ("索引")) -> (element #2=w2263:string, element #3=w2262:string)  [unwired: 1 out]
          n940 = Index Array(array=w2277, index #1=0 ("索引"), index #2=3 ("索引"), index #3=7 ("索引")) -> (element #2=w2256:string, element #3=w2258:string)  [unwired: 1 out]
          n941 = case shown="\"真\", 默认" w2233 {
            tunnel: [w2297 w2308] -> w2228
            tunnel: w2233 -> [w2297 w2302]
            tunnel: w2234 -> [_ w2301]
            frame "" {
            }
            frame "真", Default {
              n942 = call "核查数据编码整合输出.vi"("字段结束"=FALSE, "数据标识"="N" ("字符串"), "数据类型"="-Check=", "污染物编码"="w01003", "数据值"=w2302) -> ("编码输出"=w2309:string)  [unwired: 6 in]
              n943 = call "核查数据编码整合输出.vi"("字段结束"=TRUE, "数据标识"="N" ("字符串"), "数据类型"="-StandardValue=", "污染物编码"="w01003", "数据精度"=2, "数据值"=w2301) -> ("编码输出"=w2305:string)  [unwired: 5 in]
              n944 = Concatenate Strings(w2309, w2305) -> (w2308:string)
            }
          }
          n945 = case shown="\"真\", 默认" w2245 {
            tunnel: w2245 -> [w2327 w2340]
            tunnel: [w2327 w2337] -> w2230
            tunnel: w2246 -> [_ w2333]
            frame "" {
            }
            frame "真", Default {
              n946 = call "核查数据编码整合输出.vi"("字段结束"=FALSE, "数据标识"="N" ("字符串"), "数据类型"="-Check=", "污染物编码"="w01009", "数据值"=w2340) -> ("编码输出"=w2338:string)  [unwired: 6 in]
              n947 = call "核查数据编码整合输出.vi"("字段结束"=TRUE, "数据标识"="N" ("字符串"), "数据类型"="-StandardValue=", "污染物编码"="w01009", "数据精度"=2, "数据值"=w2333) -> ("编码输出"=w2334:string)  [unwired: 5 in]
              n948 = Concatenate Strings(w2338, w2334) -> (w2337:string)
            }
          }
          n949 = case shown="\"真\", 默认" w2239 {
            tunnel: [w2312 w2323] -> w2229
            tunnel: w2239 -> [w2312 w2315]
            tunnel: w2238 -> [_ w2314]
            frame "" {
            }
            frame "真", Default {
              n950 = call "核查数据编码整合输出.vi"("字段结束"=FALSE, "数据标识"="N" ("字符串"), "数据类型"="-Check=", "污染物编码"="w01014", "数据值"=w2315) -> ("编码输出"=w2324:string)  [unwired: 6 in]
              n951 = call "核查数据编码整合输出.vi"("字段结束"=TRUE, "数据标识"="N" ("字符串"), "数据类型"="-StandardValue=", "污染物编码"="w01014", "数据精度"=2, "数据值"=w2314) -> ("编码输出"=w2320:string)  [unwired: 5 in]
              n952 = Concatenate Strings(w2324, w2320) -> (w2323:string)
            }
          }
          n953 = case shown="\"真\", 默认" w2251 {
            tunnel: w2251 -> [w2342 w2355]
            tunnel: [w2342 w2352] -> w2231
            tunnel: w2250 -> [_ w2348]
            frame "" {
            }
            frame "真", Default {
              n954 = call "核查数据编码整合输出.vi"("字段结束"=FALSE, "数据标识"="N" ("字符串"), "数据类型"="-Check=", "污染物编码"="w01001", "数据值"=w2355) -> ("编码输出"=w2353:string)  [unwired: 6 in]
              n955 = call "核查数据编码整合输出.vi"("字段结束"=TRUE, "数据标识"="N" ("字符串"), "数据类型"="-StandardValue=", "污染物编码"="w01001", "数据精度"=2, "数据值"=w2348) -> ("编码输出"=w2349:string)  [unwired: 5 in]
              n956 = Concatenate Strings(w2353, w2349) -> (w2352:string)
            }
          }
          n957 = case shown="\"真\", 默认" w2270 {
            tunnel: w2270 -> [w2417 w2430]
            tunnel: [w2417 w2426] -> w2268
            tunnel: w2269 -> [_ w2421]
            frame "" {
            }
            frame "真", Default {
              # "CODMn"
              n958 = call "核查数据编码整合输出.vi"("字段结束"=FALSE, "数据标识"="N" ("字符串"), "数据类型"="-Check=", "污染物编码"="w01019", "数据值"=w2430) -> ("编码输出"=w2427:string)  [unwired: 6 in]
              n959 = call "核查数据编码整合输出.vi"("字段结束"=TRUE, "数据标识"="N" ("字符串"), "数据类型"="-StandardValue=", "污染物编码"="w01019", "数据精度"=2, "数据值"=w2421) -> ("编码输出"=w2422:string)  [unwired: 5 in]
              n960 = Concatenate Strings(w2427, w2422) -> (w2426:string)
            }
          }
          n961 = case shown="\"真\", 默认" w2256 {
            tunnel: w2256 -> [w2357 w2370]
            tunnel: [w2357 w2367] -> w2257
            tunnel: w2258 -> [_ w2363]
            frame "" {
            }
            frame "真", Default {
              n962 = call "核查数据编码整合输出.vi"("字段结束"=FALSE, "数据标识"="N" ("字符串"), "数据类型"="-Check=", "污染物编码"="w01018", "数据值"=w2370) -> ("编码输出"=w2368:string)  [unwired: 6 in]
              n963 = call "核查数据编码整合输出.vi"("字段结束"=TRUE, "数据标识"="N" ("字符串"), "数据类型"="-StandardValue=", "污染物编码"="w01018", "数据精度"=2, "数据值"=w2363) -> ("编码输出"=w2364:string)  [unwired: 5 in]
              n964 = Concatenate Strings(w2368, w2364) -> (w2367:string)
            }
          }
          n965 = case shown="\"真\", 默认" w2267 {
            tunnel: w2267 -> [w2402 w2415]
            tunnel: [w2402 w2412] -> w2265
            tunnel: w2266 -> [_ w2408]
            frame "" {
            }
            frame "真", Default {
              n966 = call "核查数据编码整合输出.vi"("字段结束"=FALSE, "数据标识"="N" ("字符串"), "数据类型"="-Check=", "污染物编码"="w21003", "数据值"=w2415) -> ("编码输出"=w2413:string)  [unwired: 6 in]
              n967 = call "核查数据编码整合输出.vi"("字段结束"=TRUE, "数据标识"="N" ("字符串"), "数据类型"="-StandardValue=", "污染物编码"="w21003", "数据精度"=2, "数据值"=w2408) -> ("编码输出"=w2409:string)  [unwired: 5 in]
              n968 = Concatenate Strings(w2413, w2409) -> (w2412:string)
            }
          }
          n969 = case shown="\"真\", 默认" w2263 {
            tunnel: w2263 -> [w2387 w2400]
            tunnel: [w2387 w2397] -> w2264
            tunnel: w2262 -> [_ w2393]
            frame "" {
            }
            frame "真", Default {
              n970 = call "核查数据编码整合输出.vi"("字段结束"=FALSE, "数据标识"="N" ("字符串"), "数据类型"="-Check=", "污染物编码"="w21011", "数据值"=w2400) -> ("编码输出"=w2398:string)  [unwired: 6 in]
              n971 = call "核查数据编码整合输出.vi"("字段结束"=TRUE, "数据标识"="N" ("字符串"), "数据类型"="-StandardValue=", "污染物编码"="w21011", "数据精度"=2, "数据值"=w2393) -> ("编码输出"=w2394:string)  [unwired: 5 in]
              n972 = Concatenate Strings(w2398, w2394) -> (w2397:string)
            }
          }
          n973 = case shown="\"真\", 默认" w2261 {
            tunnel: w2261 -> [w2372 w2385]
            tunnel: [w2372 w2382] -> w2259
            tunnel: w2260 -> [_ w2378]
            frame "" {
            }
            frame "真", Default {
              n974 = call "核查数据编码整合输出.vi"("字段结束"=FALSE, "数据标识"="N" ("字符串"), "数据类型"="-Check=", "污染物编码"="w21001", "数据值"=w2385) -> ("编码输出"=w2383:string)  [unwired: 6 in]
              n975 = call "核查数据编码整合输出.vi"("字段结束"=TRUE, "数据标识"="N" ("字符串"), "数据类型"="-StandardValue=", "污染物编码"="w21001", "数据精度"=2, "数据值"=w2378) -> ("编码输出"=w2379:string)  [unwired: 5 in]
              n976 = Concatenate Strings(w2383, w2379) -> (w2382:string)
            }
          }
          n977 = call "规范时间戳.vi"("字符串"=w2272) -> ("result string"=w2271:string)  [unwired: 10 in]
          n978 = Format Into String(format string="DataTime=%s;%s%s%s%s%s%s%s%s%s" ("格式字符串"), w2271, w2268, w2265, w2264, w2259, w2257, w2231, w2230, w2229, w2228) -> (resulting string=w2274:string)  [unwired: 2 in, 1 out]
          n979 = Empty String/Path?(string/path=w2271) -> (empty?=w2275:bool)
          n980 = case shown="假" w2275 {
            tunnel: [w2434 ""] -> w2273
            tunnel: w2274 -> [w2434 _]
            frame False {
              n981 = global read "全局 小时数据发送次数.vi" "小时数据发送次数"() -> (w2433:i32)
              n982 = Increment(x=w2433) -> (x+1=w2432:i32)
              n983 = global write "全局 小时数据发送次数.vi" "小时数据发送次数"(w2432) -> ()
            }
            frame True {
              n984 = global read "全局 小时数据发送次数.vi" "小时数据发送次数"() -> (w2436:i32)
              n985 = Increment(x=w2436) -> (x+1=w2435:i32)
              n986 = global write "全局 小时数据发送次数.vi" "小时数据发送次数"(w2435) -> ()
            }
          }
        }
        frame "返回执行结果" {
        }
      }
    }
    frame "空白测试", "跨度核查", "零点核查" {
      # "提取空白测试数据/零点核查数据/跨度核查数据"
      n987 = global read "全局 小时数据发送次数.vi" "小时数据发送次数"() -> (w2446:i32)
      n988 = global read "全局 小时数据发送次数.vi" "小时数据发送次数"() -> (w2448:i32)
      n989 = global read "全局 小时数据发送次数.vi" "小时数据发送次数"() -> (w2444:i32)
      n990 = global read "全局 小时数据发送次数.vi" "小时数据发送次数"() -> (w2440:i32)
      n991 = global read "全局 小时数据发送次数.vi" "小时数据发送次数"() -> (w2442:i32)
      n992 = Index Array(array=w2454, index (row)=w2446) -> (element=w2445:string[])  [unwired: 1 in]
      n993 = Index Array(array=w2455, index (row)=w2448) -> (element=w2447:string[])  [unwired: 1 in]
      n994 = Index Array(array=w2453, index (row)=w2444) -> (element=w2443:string[])  [unwired: 1 in]
      n995 = Index Array(array=w2450, index (row)=w2440) -> (element=w2439:string[])  [unwired: 1 in]
      n996 = Index Array(array=w2452, index (row)=w2442) -> (element=w2441:string[])  [unwired: 1 in]
      n997 = global read "全局1.vi" "枚举"() -> (w2449:enum16{"返回请求应答", "上传数据", "返回执行结果"})
      n998 = case shown="\"上传数据\"" w2449 {
        tunnel: ["QnRtn=1" w2487 "ExeRtn=1"] -> w2451
        tunnel: w2447 -> [_ w2507 _]
        tunnel: w2443 -> [_ w2506 _]
        tunnel: w2441 -> [_ w2505 _]
        tunnel: w2445 -> [_ w2503 _]
        tunnel: w2439 -> [_ w2491 _]
        frame "返回请求应答", Default {
          (unwired) 0 ("当前包数")
          n999 = global read "全局 数据数组大小.vi" "数据数组大小"() -> (w2457:i32)
          n1000 = Equal To 0?(x=w2457) -> (x = 0?=w2456:bool)
          n1001 = case shown="真" w2456 {
            frame False {
            }
            frame True {
              n1002 = global read "全局 小时数据发送次数.vi" "小时数据发送次数"() -> (w2460:i32)
              n1003 = Increment(x=w2460) -> (x+1=w2459:i32)
              n1004 = global write "全局 小时数据发送次数.vi" "小时数据发送次数"(w2459) -> ()
            }
          }
        }
        frame "上传数据" {
          # "将非空数组的时间戳写入"
          n1005 = Index Array(array=w2505, index #1=0 ("索引"), index #2=3 ("索引"), index #3=7 ("索引")) -> (element #2=w2468:string, element #3=w2467:string)  [unwired: 1 out]
          n1006 = Index Array(array=w2503, index #1=0 ("索引"), index #2=3 ("索引"), index #3=7 ("索引")) -> (element #1=w2486:string, element #2=w2478:string, element #3=w2477:string)
          n1007 = Index Array(array=w2507, index #1=0 ("索引"), index #2=3 ("索引"), index #3=7 ("索引")) -> (element #2=w2483:string, element #3=w2482:string)  [unwired: 1 out]
          n1008 = Index Array(array=w2506, index #1=0 ("索引"), index #2=3 ("索引"), index #3=7 ("索引")) -> (element #2=w2473:string, element #3=w2472:string)  [unwired: 1 out]
          n1009 = Index Array(array=w2491, index #1=0 ("索引"), index #2=3 ("索引"), index #3=7 ("索引")) -> (element #2=w2463:string, element #3=w2462:string)  [unwired: 1 out]
          n1010 = call "规范时间戳.vi"("字符串"=w2486) -> ("result string"=w2485:string)  [unwired: 10 in]
          n1011 = call "零点跨度数据组合 (子VI).vi"("span value"="0", "standard value"=w2482, "check value"=w2483, "污染物编码"="w01019") -> ("组合输出"=w2481:string)  [unwired: 7 in]
          n1012 = call "零点跨度数据组合 (子VI).vi"("standard value"=w2462, "check value"=w2463, "污染物编码"="w01018") -> ("组合输出"=w2461:string)  [unwired: 8 in]
          n1013 = call "零点跨度数据组合 (子VI).vi"("span value"="0", "standard value"=w2467, "check value"=w2468, "污染物编码"="w21001") -> ("组合输出"=w2465:string)  [unwired: 7 in]
          n1014 = call "零点跨度数据组合 (子VI).vi"("span value"="0", "standard value"=w2477, "check value"=w2478, "污染物编码"="w21003") -> ("组合输出"=w2475:string)  [unwired: 7 in]
          n1015 = call "零点跨度数据组合 (子VI).vi"("span value"="0", "standard value"=w2472, "check value"=w2473, "污染物编码"="w21011") -> ("组合输出"=w2471:string)  [unwired: 7 in]
          n1016 = Format Into String(format string="DataTime=%s;%s%s%s%s%s" ("格式字符串"), w2485, w2481, w2475, w2471, w2465, w2461) -> (resulting string=w2488:string)  [unwired: 2 in, 1 out]
          n1017 = Empty String/Path?(string/path=w2485) -> (empty?=w2489:bool)
          n1018 = case shown="假" w2489 {
            tunnel: [w2513 ""] -> w2487
            tunnel: w2488 -> [w2513 _]
            frame False {
              n1019 = global read "全局 小时数据发送次数.vi" "小时数据发送次数"() -> (w2512:i32)
              n1020 = Increment(x=w2512) -> (x+1=w2511:i32)
              n1021 = global write "全局 小时数据发送次数.vi" "小时数据发送次数"(w2511) -> ()
            }
            frame True {
              n1022 = global read "全局 小时数据发送次数.vi" "小时数据发送次数"() -> (w2515:i32)
              n1023 = Increment(x=w2515) -> (x+1=w2514:i32)
              n1024 = global write "全局 小时数据发送次数.vi" "小时数据发送次数"(w2514) -> ()
            }
          }
        }
        frame "返回执行结果" {
        }
      }
    }
    frame "提取加标回收" {
      # "提取加标回收数据"
      n1025 = global read "全局1.vi" "枚举"() -> (w2524:enum16{"返回请求应答", "上传数据", "返回执行结果"})
      n1026 = case shown="\"上传数据\"" w2524 {
        tunnel: ["QnRtn=1" w2546 "ExeRtn=1"] -> w2518
        tunnel: w2522 -> [_ w2548 _]
        tunnel: w2523 -> [_ w2541 _]
        tunnel: w2521 -> [_ w2538 _]
        tunnel: w2520 -> [_ w2535 _]
        tunnel: w2519 -> [_ w2532 _]
        frame "返回请求应答", Default {
          n1027 = global read "全局 数据数组大小.vi" "数据数组大小"() -> (w2525:i32)
          n1028 = Equal To 0?(x=w2525) -> (x = 0?=w2526:bool)
          n1029 = case shown="真" w2526 {
            frame False {
            }
            frame True {
              n1030 = global read "全局 小时数据发送次数.vi" "小时数据发送次数"() -> (w2529:i32)
              n1031 = Increment(x=w2529) -> (x+1=w2528:i32)
              n1032 = global write "全局 小时数据发送次数.vi" "小时数据发送次数"(w2528) -> ()
            }
          }
        }
        frame "上传数据" {
          # "w01001-Check=63.0,w01001-WaterTime=20160801080000,w01001-Water=45.23,w01001-Chroma=1000,w01001-Volume=0.2,w01001-DVolume=200,w01003-Flag=N;"
          # "总氮"
          # "总磷"
          # "CODMn"
          n1033 = global read "全局 小时数据发送次数.vi" "小时数据发送次数"() -> (w2531:i32)
          n1034 = call "加标回收数据组合 (子VI).vi"("小时数据发送次数"=w2531, "数据"=w2532, "污染物编码"="w01018") -> ("组合输出"=w2530:string)  [unwired: 7 in, 1 out]
          n1035 = call "加标回收数据组合 (子VI).vi"("小时数据发送次数"=w2531, "数据"=w2541, "污染物编码"="w21003") -> ("组合输出"=w2540:string)  [unwired: 7 in, 1 out]
          n1036 = call "加标回收数据组合 (子VI).vi"("小时数据发送次数"=w2531, "数据"=w2535, "污染物编码"="w21001") -> ("组合输出"=w2534:string)  [unwired: 7 in, 1 out]
          n1037 = call "加标回收数据组合 (子VI).vi"("小时数据发送次数"=w2531, "数据"=w2538, "污染物编码"="w21011") -> ("组合输出"=w2537:string)  [unwired: 7 in, 1 out]
          n1038 = call "加标回收数据组合 (子VI).vi"("小时数据发送次数"=w2531, "数据"=w2548, "污染物编码"="w01019") -> ("组合输出"=w2543:string, "datatime"=w2550:string)  [unwired: 7 in]
          n1039 = call "规范时间戳.vi"("字符串"=w2550) -> ("result string"=w2549:string)  [unwired: 10 in]
          n1040 = Empty String/Path?(string/path=w2549) -> (empty?=w2545:bool)
          n1041 = Format Into String(format string="DataTime=%s;%s%s%s%s%s" ("格式字符串"), w2549, w2543, w2540, w2537, w2534, w2530) -> (resulting string=w2547:string)  [unwired: 2 in, 1 out]
          n1042 = case shown="真" w2545 {
            tunnel: [w2554 ""] -> w2546
            tunnel: w2547 -> [w2554 _]
            frame False {
              n1043 = global read "全局 小时数据发送次数.vi" "小时数据发送次数"() -> (w2553:i32)
              n1044 = Increment(x=w2553) -> (x+1=w2552:i32)
              n1045 = global write "全局 小时数据发送次数.vi" "小时数据发送次数"(w2552) -> ()
            }
            frame True {
              n1046 = global read "全局 小时数据发送次数.vi" "小时数据发送次数"() -> (w2556:i32)
              n1047 = Increment(x=w2556) -> (x+1=w2555:i32)
              n1048 = global write "全局 小时数据发送次数.vi" "小时数据发送次数"(w2555) -> ()
            }
          }
        }
        frame "返回执行结果" {
        }
      }
    }
    frame "提取平行样" {
      # "提取平行样数据"
      n1049 = global read "全局1.vi" "枚举"() -> (w2565:enum16{"返回请求应答", "上传数据", "返回执行结果"})
      n1050 = case shown="\"上传数据\"" w2565 {
        tunnel: ["QnRtn=1" w2592 "ExeRtn=1"] -> w2564
        tunnel: w2563 -> [_ w2585 _]
        tunnel: w2562 -> [_ w2583 _]
        tunnel: w2561 -> [_ w2580 _]
        tunnel: w2559 -> [_ w2577 _]
        tunnel: w2560 -> [_ w2573 _]
        frame "返回请求应答", Default {
          n1051 = global read "全局 数据数组大小.vi" "数据数组大小"() -> (w2566:i32)
          n1052 = Equal To 0?(x=w2566) -> (x = 0?=w2567:bool)
          n1053 = case shown="真" w2567 {
            frame False {
            }
            frame True {
              n1054 = global read "全局 小时数据发送次数.vi" "小时数据发送次数"() -> (w2570:i32)
              n1055 = Increment(x=w2570) -> (x+1=w2569:i32)
              n1056 = global write "全局 小时数据发送次数.vi" "小时数据发送次数"(w2569) -> ()
            }
          }
        }
        frame "上传数据" {
          # "CODMn"
          n1057 = global read "全局 小时数据发送次数.vi" "小时数据发送次数"() -> (w2574:i32)
          n1058 = Index Array(array=w2585, index (row)=w2574) -> (element=w2590:string[])  [unwired: 1 in]
          n1059 = Index Array(array=w2590, index=0 ("索引")) -> (element=w2587:string)
          n1060 = call "规范时间戳.vi"("字符串"=w2587) -> ("result string"=w2588:string)  [unwired: 10 in]
          n1061 = call "平行样集成干预数据组合(子VI).vi"("污染物编码"="w01019", "数据输入"=w2585, "小时数据发送次数"=w2574) -> ("输出组合"=w2584:string)  [unwired: 8 in]
          n1062 = call "平行样集成干预数据组合(子VI).vi"("污染物编码"="w21003", "数据输入"=w2583, "小时数据发送次数"=w2574) -> ("输出组合"=w2581:string)  [unwired: 8 in]
          n1063 = call "平行样集成干预数据组合(子VI).vi"("污染物编码"="w21011", "数据输入"=w2580, "小时数据发送次数"=w2574) -> ("输出组合"=w2578:string)  [unwired: 8 in]
          n1064 = call "平行样集成干预数据组合(子VI).vi"("污染物编码"="w21001", "数据输入"=w2577, "小时数据发送次数"=w2574) -> ("输出组合"=w2575:string)  [unwired: 8 in]
          n1065 = call "平行样集成干预数据组合(子VI).vi"("污染物编码"="w01018", "数据输入"=w2573, "小时数据发送次数"=w2574) -> ("输出组合"=w2571:string)  [unwired: 8 in]
          n1066 = Empty String/Path?(string/path=w2587) -> (empty?=w2591:bool)
          n1067 = Format Into String(format string="DataTime=%s;%s%s%s%s%s" ("格式字符串"), w2588, w2584, w2581, w2578, w2575, w2571) -> (resulting string=w2593:string)  [unwired: 2 in, 1 out]
          n1068 = case shown="真" w2591 {
            tunnel: [w2597 ""] -> w2592
            tunnel: w2593 -> [w2597 _]
            frame False {
              n1069 = global read "全局 小时数据发送次数.vi" "小时数据发送次数"() -> (w2596:i32)
              n1070 = Increment(x=w2596) -> (x+1=w2595:i32)
              n1071 = global write "全局 小时数据发送次数.vi" "小时数据发送次数"(w2595) -> ()
            }
            frame True {
              n1072 = global read "全局 小时数据发送次数.vi" "小时数据发送次数"() -> (w2599:i32)
              n1073 = Increment(x=w2599) -> (x+1=w2598:i32)
              n1074 = global write "全局 小时数据发送次数.vi" "小时数据发送次数"(w2598) -> ()
            }
          }
        }
        frame "返回执行结果" {
        }
      }
    }
    frame "提取集成干预" {
      # "提取平行样数据"
      n1075 = global read "全局1.vi" "枚举"() -> (w2613:enum16{"返回请求应答", "上传数据", "返回执行结果"})
      n1076 = case shown="\"上传数据\"" w2613 {
        tunnel: ["QnRtn=1" w2655 "ExeRtn=1"] -> w2612
        tunnel: w2611 -> [_ w2621 _]
        tunnel: w2610 -> [_ w2627 _]
        tunnel: w2604 -> [_ w2630 _]
        tunnel: w2605 -> [_ w2633 _]
        tunnel: w2606 -> [_ w2637 _]
        tunnel: w2603 -> [_ w2639 _]
        tunnel: w2602 -> [_ w2642 _]
        tunnel: w2607 -> [_ w2645 _]
        tunnel: w2609 -> [_ w2649 _]
        tunnel: w2608 -> [_ w2651 _]
        frame "返回请求应答", Default {
          n1077 = global read "全局 数据数组大小.vi" "数据数组大小"() -> (w2614:i32)
          n1078 = Equal To 0?(x=w2614) -> (x = 0?=w2615:bool)
          n1079 = case shown="真" w2615 {
            frame False {
            }
            frame True {
              n1080 = global read "全局 小时数据发送次数.vi" "小时数据发送次数"() -> (w2618:i32)
              n1081 = Increment(x=w2618) -> (x+1=w2617:i32)
              n1082 = global write "全局 小时数据发送次数.vi" "小时数据发送次数"(w2617) -> ()
            }
          }
        }
        frame "上传数据" {
          # "CODMn"
          n1083 = global read "全局 小时数据发送次数.vi" "小时数据发送次数"() -> (w2622:i32)
          n1084 = Index Array(array=w2621, index (row)=w2622) -> (element=w2625:string[])  [unwired: 1 in]
          n1085 = Index Array(array=w2625, index=0 ("索引")) -> (element=w2623:string)
          n1086 = call "规范时间戳.vi"("字符串"=w2623) -> ("result string"=w2653:string)  [unwired: 10 in]
          n1087 = call "平行样集成干预数据组合(子VI).vi"("污染物编码"="w21001", "数据输入"=w2649, "小时数据发送次数"=w2622) -> ("输出组合"=w2647:string)  [unwired: 8 in]
          n1088 = call "平行样集成干预数据组合(子VI).vi"("污染物编码"="w21011", "数据输入"=w2645, "小时数据发送次数"=w2622) -> ("输出组合"=w2644:string)  [unwired: 8 in]
          n1089 = call "平行样集成干预数据组合(子VI).vi"("污染物编码"="w01014", "数据输入"=w2639, "小时数据发送次数"=w2622) -> ("输出组合"=w2638:string)  [unwired: 8 in]
          n1090 = call "平行样集成干预数据组合(子VI).vi"("污染物编码"="w01019", "数据输入"=w2621, "小时数据发送次数"=w2622) -> ("输出组合"=w2619:string)  [unwired: 8 in]
          n1091 = call "平行样集成干预数据组合(子VI).vi"("污染物编码"="w01009", "数据输入"=w2637, "小时数据发送次数"=w2622) -> ("输出组合"=w2635:string)  [unwired: 8 in]
          n1092 = call "平行样集成干预数据组合(子VI).vi"("污染物编码"="w01001", "数据输入"=w2633, "小时数据发送次数"=w2622) -> ("输出组合"=w2632:string)  [unwired: 8 in]
          n1093 = call "平行样集成干预数据组合(子VI).vi"("污染物编码"="w21003", "数据输入"=w2627, "小时数据发送次数"=w2622) -> ("输出组合"=w2626:string)  [unwired: 8 in]
          n1094 = call "平行样集成干预数据组合(子VI).vi"("污染物编码"="w01010", "数据输入"=w2630, "小时数据发送次数"=w2622) -> ("输出组合"=w2629:string)  [unwired: 8 in]
          n1095 = call "平行样集成干预数据组合(子VI).vi"("污染物编码"="w01003", "数据输入"=w2642, "小时数据发送次数"=w2622) -> ("输出组合"=w2641:string)  [unwired: 8 in]
          n1096 = call "平行样集成干预数据组合(子VI).vi"("污染物编码"="w01018", "数据输入"=w2651, "小时数据发送次数"=w2622) -> ("输出组合"=w2652:string)  [unwired: 8 in]
          n1097 = Empty String/Path?(string/path=w2623) -> (empty?=w2654:bool)
          n1098 = Format Into String(format string="DataTime=%s;%s%s%s%s%s%s%s%s%s%s" ("格式字符串"), w2653, w2619, w2626, w2629, w2632, w2635, w2638, w2641, w2644, w2647, w2652) -> (resulting string=w2656:string)  [unwired: 2 in, 1 out]
          n1099 = case shown="真" w2654 {
            tunnel: [w2660 ""] -> w2655
            tunnel: w2656 -> [w2660 _]
            frame False {
              n1100 = global read "全局 小时数据发送次数.vi" "小时数据发送次数"() -> (w2659:i32)
              n1101 = Increment(x=w2659) -> (x+1=w2658:i32)
              n1102 = global write "全局 小时数据发送次数.vi" "小时数据发送次数"(w2658) -> ()
            }
            frame True {
              n1103 = global read "全局 小时数据发送次数.vi" "小时数据发送次数"() -> (w2662:i32)
              n1104 = Increment(x=w2662) -> (x+1=w2661:i32)
              n1105 = global write "全局 小时数据发送次数.vi" "小时数据发送次数"(w2661) -> ()
            }
          }
        }
        frame "返回执行结果" {
        }
      }
    }
    frame "操作日志" {
      n1106 = global read "全局 小时数据发送次数.vi" "小时数据发送次数"() -> (w2675:i32)
      n1107 = global read "全局 小时数据发送次数.vi" "小时数据发送次数"() -> (w2677:i32)
      n1108 = global read "全局 小时数据发送次数.vi" "小时数据发送次数"() -> (w2673:i32)
      n1109 = global read "全局 小时数据发送次数.vi" "小时数据发送次数"() -> (w2672:i32)
      n1110 = global read "全局 小时数据发送次数.vi" "小时数据发送次数"() -> (w2667:i32)
      n1111 = global read "全局 小时数据发送次数.vi" "小时数据发送次数"() -> (w2669:i32)
      n1112 = Index Array(array=w2683, index (row)=w2675) -> (element=w2674:string[])  [unwired: 1 in]
      n1113 = Index Array(array=w2682, index (row)=w2677) -> (element=w2676:string[])  [unwired: 1 in]
      n1114 = Index Array(array=w2680, index (row)=w2673) -> (element=w2671:string[])  [unwired: 1 in]
      n1115 = Index Array(array=w2679, index (row)=w2672) -> (element=w2670:string[])  [unwired: 1 in]
      n1116 = Index Array(array=w2666, index (row)=w2667) -> (element=w2665:string[])  [unwired: 1 in]
      n1117 = global read "全局1.vi" "枚举"() -> (w2678:enum16{"返回请求应答", "上传数据", "返回执行结果"})
      n1118 = Index Array(array=w2681, index (row)=w2669) -> (element=w2668:string[])  [unwired: 1 in]
      n1119 = case shown="\"上传数据\"" w2678 {
        tunnel: ["QnRtn=1" w2705 "ExeRtn=1"] -> w2684
        tunnel: w2676 -> [_ w2724 _]
        tunnel: w2674 -> [_ w2722 _]
        tunnel: w2671 -> [_ w2721 _]
        tunnel: w2670 -> [_ w2720 _]
        tunnel: w2668 -> [_ w2718 _]
        tunnel: w2665 -> [_ w2691 _]
        frame "返回请求应答", Default {
          n1120 = global read "全局 数据数组大小.vi" "数据数组大小"() -> (w2687:i32)
          n1121 = Equal To 0?(x=w2687) -> (x = 0?=w2686:bool)
          n1122 = case shown="真" w2686 {
            frame False {
            }
            frame True {
              n1123 = global read "全局 小时数据发送次数.vi" "小时数据发送次数"() -> (w2689:i32)
              n1124 = Increment(x=w2689) -> (x+1=w2688:i32)
              n1125 = global write "全局 小时数据发送次数.vi" "小时数据发送次数"(w2688) -> ()
            }
          }
        }
        frame "上传数据" {
          n1126 = Index Array(array=w2691, index #1=0 ("索引"), index #2=2 ("索引")) -> (element #1=w2694:string, element #2=w2696:string)
          n1127 = Index Array(array=w2720, index #1=0 ("索引"), index #2=2 ("索引")) -> (element #1=w2719:string, element #2=w2709:string)
          n1128 = Index Array(array=w2724, index #1=0 ("索引"), index #2=2 ("索引")) -> (element #1=w2723:string, element #2=w2711:string)
          n1129 = Index Array(array=w2718, index #1=0 ("索引"), index #2=2 ("索引")) -> (element #1=w2717:string, element #2=w2713:string)
          n1130 = Index Array(array=w2721, index #1=0 ("索引"), index #2=2 ("索引")) -> (element #1=w2725:string, element #2=w2707:string)
          n1131 = Index Array(array=w2722, index #1=0 ("索引"), index #2=2 ("索引")) -> (element #1=w2700:string, element #2=w2716:string)
          n1132 = Empty String/Path?(string/path=w2696) -> (empty?=w2695:bool)
          n1133 = Empty String/Path?(string/path=w2709) -> (empty?=w2710:bool)
          n1134 = Empty String/Path?(string/path=w2711) -> (empty?=w2712:bool)
          n1135 = Empty String/Path?(string/path=w2707) -> (empty?=w2708:bool)
          n1136 = case shown="假" w2712 {
            tunnel: [w2760 ""] -> w2737
            tunnel: w2711 -> [w2759 _]
            tunnel: w2723 -> [_ _]
            frame False {
              # "氨氮"
              n1137 = Format Into String(format string="PolId=w21003,i11001-Info=//%s//;" ("格式字符串"), w2759) -> (resulting string=w2760:string)  [unwired: 2 in, 1 out]
            }
            frame True {
            }
          }
          n1138 = case shown="假" w2695 {
            tunnel: [w2741 ""] -> w2690
            tunnel: w2694 -> [_ _]
            tunnel: w2696 -> [w2742 _]
            frame False {
              # "CODCr"
              n1139 = Format Into String(format string="PolId=w01018,i11001-Info=//%s//;" ("格式字符串"), w2742) -> (resulting string=w2741:string)  [unwired: 2 in, 1 out]
            }
            frame True {
            }
          }
          n1140 = case shown="假" w2710 {
            tunnel: [w2755 ""] -> w2732
            tunnel: w2719 -> [_ _]
            tunnel: w2709 -> [w2756 _]
            frame False {
              # "总氮"
              n1141 = Format Into String(format string="PolId=w21001,i11001-Info=//%s//;" ("格式字符串"), w2756) -> (resulting string=w2755:string)  [unwired: 2 in, 1 out]
            }
            frame True {
            }
          }
          n1142 = Empty String/Path?(string/path=w2713) -> (empty?=w2714:bool)
          n1143 = case shown="假" w2708 {
            tunnel: [w2753 ""] -> w2733
            tunnel: w2725 -> [_ _]
            tunnel: w2707 -> [w2751 _]
            frame False {
              # "总磷"
              n1144 = Format Into String(format string="PolId=w21011,i11001-Info=//%s//;" ("格式字符串"), w2751) -> (resulting string=w2753:string)  [unwired: 2 in, 1 out]
            }
            frame True {
            }
          }
          n1145 = case shown="假" w2714 {
            tunnel: [w2765 ""] -> w2736
            tunnel: w2717 -> [_ _]
            tunnel: w2713 -> [w2763 _]
            frame False {
              # "系统日志"
              n1146 = Format Into String(format string="PolId=w00000,i21001-Info=//%s//;" ("格式字符串"), w2763) -> (resulting string=w2765:string)  [unwired: 2 in, 1 out]
            }
            frame True {
            }
          }
          n1147 = Empty String/Path?(string/path=w2716) -> (empty?=w2715:bool)
          n1148 = case shown="假" w2715 {
            tunnel: [w2768 ""] -> w2738
            tunnel: w2700 -> [_ _]
            tunnel: w2716 -> [w2767 _]
            frame False {
              # "高锰酸钾盐"
              n1149 = Format Into String(format string="PolId=w01019,i11001-Info=//%s//;" ("格式字符串"), w2767) -> (resulting string=w2768:string)  [unwired: 2 in, 1 out]
            }
            frame True {
            }
          }
          n1150 = call "规范时间戳.vi"("字符串"=w2700) -> ("result string"=w2698:string)  [unwired: 10 in]
          n1151 = Format Into String(format string="DataTime=%s;", w2698) -> (resulting string=w2697:string)  [unwired: 2 in, 1 out]
          n1152 = Concatenate Strings(w2697, w2738, w2737, w2736, w2733, w2732, w2690) -> (w2702:string)
          n1153 = String Length(string=w2702) -> (length=w2704:i32)
          n1154 = Empty String/Path?(string/path=w2702) -> (empty?=w2706:bool)
          n1155 = Decrement(x=w2704) -> (x-1=w2703:i32)
          n1156 = String Subset(string=w2702, length (rest)=w2703) -> (substring=w2701:string)  [unwired: 1 in]
          n1157 = case shown="假" w2706 {
            tunnel: [w2747 ""] -> w2705
            tunnel: w2701 -> [w2747 _]
            frame False {
              n1158 = global read "全局 小时数据发送次数.vi" "小时数据发送次数"() -> (w2746:i32)
              n1159 = Increment(x=w2746) -> (x+1=w2745:i32)
              n1160 = global write "全局 小时数据发送次数.vi" "小时数据发送次数"(w2745) -> ()
            }
            frame True {
              n1161 = global read "全局 小时数据发送次数.vi" "小时数据发送次数"() -> (w2749:i32)
              n1162 = Increment(x=w2749) -> (x+1=w2748:i32)
              n1163 = global write "全局 小时数据发送次数.vi" "小时数据发送次数"(w2748) -> ()
            }
          }
        }
        frame "返回执行结果" {
        }
      }
    }
    frame "仪器参数" {
      n1164 = global read "全局 小时数据发送次数.vi" "小时数据发送次数"() -> (w2803:i32)
      n1165 = global read "全局 小时数据发送次数.vi" "小时数据发送次数"() -> (w2805:i32)
      n1166 = global read "全局 小时数据发送次数.vi" "小时数据发送次数"() -> (w2801:i32)
      n1167 = global read "全局 小时数据发送次数.vi" "小时数据发送次数"() -> (w2786:i32)
      n1168 = global read "全局 小时数据发送次数.vi" "小时数据发送次数"() -> (w2780:i32)
      n1169 = global read "全局 小时数据发送次数.vi" "小时数据发送次数"() -> (w2782:i32)
      n1170 = global read "全局 小时数据发送次数.vi" "小时数据发送次数"() -> (w2781:i32)
      n1171 = global read "全局 小时数据发送次数.vi" "小时数据发送次数"() -> (w2797:i32)
      n1172 = global read "全局 小时数据发送次数.vi" "小时数据发送次数"() -> (w2783:i32)
      n1173 = global read "全局 小时数据发送次数.vi" "小时数据发送次数"() -> (w2792:i32)
      n1174 = global read "全局 小时数据发送次数.vi" "小时数据发送次数"() -> (w2800:i32)
      n1175 = global read "全局 小时数据发送次数.vi" "小时数据发送次数"() -> (w2796:i32)
      n1176 = global read "全局 小时数据发送次数.vi" "小时数据发送次数"() -> (w2789:i32)
      n1177 = Index Array(array=w2811, index (row)=w2803) -> (element=w2802:string[])  [unwired: 1 in]
      n1178 = Index Array(array=w2810, index (row)=w2805) -> (element=w2804:string[])  [unwired: 1 in]
      n1179 = Index Array(array=w2785, index (row)=w2786) -> (element=w2784:string[])  [unwired: 1 in]
      n1180 = Index Array(array=w2773, index (row)=w2780) -> (element=w2772:string[])  [unwired: 1 in]
      n1181 = Index Array(array=w2777, index (row)=w2782) -> (element=w2776:string[])  [unwired: 1 in]
      n1182 = Index Array(array=w2775, index (row)=w2781) -> (element=w2774:string[])  [unwired: 1 in]
      n1183 = Index Array(array=w2809, index (row)=w2797) -> (element=w2793:string[])  [unwired: 1 in]
      n1184 = Index Array(array=w2808, index (row)=w2801) -> (element=w2799:string[])  [unwired: 1 in]
      n1185 = Index Array(array=w2779, index (row)=w2783) -> (element=w2778:string[])  [unwired: 1 in]
      n1186 = Index Array(array=w2791, index (row)=w2792) -> (element=w2790:string[])  [unwired: 1 in]
      n1187 = Index Array(array=w2807, index (row)=w2800) -> (element=w2798:string[])  [unwired: 1 in]
      n1188 = Index Array(array=w2795, index (row)=w2796) -> (element=w2794:string[])  [unwired: 1 in]
      n1189 = Index Array(array=w2788, index (row)=w2789) -> (element=w2787:string[])  [unwired: 1 in]
      n1190 = global read "全局1.vi" "枚举"() -> (w2806:enum16{"返回请求应答", "上传数据", "返回执行结果"})
      n1191 = case shown="\"上传数据\"" w2806 {
        tunnel: ["QnRtn=1" w2877 "ExeRtn=1"] -> w2812
        tunnel: w2804 -> [_ w2840 _]
        tunnel: w2802 -> [_ w2837 _]
        tunnel: w2799 -> [_ w2843 _]
        tunnel: w2798 -> [_ w2846 _]
        tunnel: w2794 -> [_ w2849 _]
        tunnel: w2793 -> [_ w2874 _]
        tunnel: w2790 -> [_ w2870 _]
        tunnel: w2787 -> [_ w2868 _]
        tunnel: w2784 -> [_ w2866 _]
        tunnel: w2778 -> [_ w2864 _]
        tunnel: w2776 -> [_ w2862 _]
        tunnel: w2774 -> [_ w2860 _]
        tunnel: w2772 -> [_ w2858 _]
        frame "返回请求应答", Default {
          n1192 = global read "全局 数据数组大小.vi" "数据数组大小"() -> (w2815:i32)
          n1193 = Equal To 0?(x=w2815) -> (x = 0?=w2814:bool)
          n1194 = case shown="真" w2814 {
            frame False {
            }
            frame True {
              n1195 = global read "全局 小时数据发送次数.vi" "小时数据发送次数"() -> (w2817:i32)
              n1196 = Increment(x=w2817) -> (x+1=w2816:i32)
              n1197 = global write "全局 小时数据发送次数.vi" "小时数据发送次数"(w2816) -> ()
            }
          }
        }
        frame "上传数据" {
          n1198 = call "关键参数组合 (子VI).vi"("table"="仪器参数", "因子编码"="w21001", "DO"=w2846) -> ("字符串"=w2845:string)  [unwired: 8 in]
          n1199 = call "关键参数组合 (子VI).vi"("table"="仪器参数", "因子编码"="w01001", "DO"=w2870) -> ("字符串"=w2857:string)  [unwired: 8 in]
          n1200 = call "关键参数组合 (子VI).vi"("table"="仪器参数", "因子编码"="w01019", "DO"=w2837) -> ("字符串"=w2835:string)  [unwired: 8 in]
          n1201 = call "关键参数组合 (子VI).vi"("table"="仪器参数", "因子编码"="w01014", "DO"=w2868) -> ("字符串"=w2856:string)  [unwired: 8 in]
          n1202 = call "关键参数组合 (子VI).vi"("table"="仪器参数", "因子编码"="w01003", "DO"=w2864) -> ("字符串"=w2854:string)  [unwired: 8 in]
          n1203 = call "关键参数组合 (子VI).vi"("table"="仪器参数", "因子编码"="w01010", "DO"=w2866) -> ("字符串"=w2855:string)  [unwired: 8 in]
          n1204 = call "关键参数组合 (子VI).vi"("table"="仪器参数", "因子编码"="w01018", "DO"=w2849) -> ("字符串"=w2848:string)  [unwired: 8 in]
          n1205 = call "关键参数组合 (子VI).vi"("table"="仪器参数", "因子编码"="w01009", "DO"=w2874) -> ("字符串"=w2873:string)  [unwired: 8 in]
          n1206 = call "关键参数组合 (子VI).vi"("table"="仪器参数", "因子编码"="w21011", "DO"=w2843) -> ("字符串"=w2842:string)  [unwired: 8 in]
          n1207 = call "关键参数组合 (子VI).vi"("table"="仪器参数", "因子编码"="w01016", "DO"=w2862) -> ("字符串"=w2853:string)  [unwired: 8 in]
          n1208 = call "关键参数组合 (子VI).vi"("table"="仪器参数", "因子编码"="w21003", "DO"=w2840) -> ("字符串"=w2839:string)  [unwired: 8 in]
          n1209 = call "关键参数组合 (子VI).vi"("table"="仪器参数", "因子编码"="w01100", "DO"=w2858) -> ("字符串"=w2851:string)  [unwired: 8 in]
          n1210 = call "关键参数组合 (子VI).vi"("table"="仪器参数", "因子编码"="w19011", "DO"=w2860) -> ("字符串"=w2852:string)  [unwired: 8 in]
          n1211 = Index Array(array=w2837) -> (element=w2836:string)  [unwired: 1 in]
          n1212 = call "规范时间戳.vi"("字符串"=w2836) -> ("result string"=w2875:string)  [unwired: 10 in]
          n1213 = Format Into String(format string="DataTime=%s;%s%s%s%s%s%s%s%s%s%s%s%s%s" ("格式字符串"), w2875, w2835, w2839, w2842, w2845, w2848, w2873, w2857, w2856, w2855, w2854, w2853, w2852, w2851) -> (resulting string=w2819:string)  [unwired: 2 in, 1 out]
          n1214 = String Length(string=w2819) -> (length=w2820:i32)
          n1215 = Decrement(x=w2820) -> (x-1=w2821:i32)
          n1216 = String Subset(string=w2819, length (rest)=w2821) -> (substring=w2818:string)  [unwired: 1 in]
          n1217 = Empty String/Path?(string/path=w2818) -> (empty?=w2878:bool)
          n1218 = case shown="假" w2878 {
            tunnel: [w2881 ""] -> w2877
            tunnel: w2818 -> [w2881 _]
            frame False {
              n1219 = global read "全局 小时数据发送次数.vi" "小时数据发送次数"() -> (w2880:i32)
              n1220 = Increment(x=w2880) -> (x+1=w2879:i32)
              n1221 = global write "全局 小时数据发送次数.vi" "小时数据发送次数"(w2879) -> ()
            }
            frame True {
              n1222 = global read "全局 小时数据发送次数.vi" "小时数据发送次数"() -> (w2883:i32)
              n1223 = Increment(x=w2883) -> (x+1=w2882:i32)
              n1224 = global write "全局 小时数据发送次数.vi" "小时数据发送次数"(w2882) -> ()
            }
          }
        }
        frame "返回执行结果" {
        }
      }
    }
    frame "3090仪器参数" {
      n1225 = global read "全局 小时数据发送次数.vi" "小时数据发送次数"() -> (w2917:i32)
      n1226 = global read "全局 小时数据发送次数.vi" "小时数据发送次数"() -> (w2919:i32)
      n1227 = global read "全局 小时数据发送次数.vi" "小时数据发送次数"() -> (w2915:i32)
      n1228 = global read "全局 小时数据发送次数.vi" "小时数据发送次数"() -> (w2900:i32)
      n1229 = global read "全局 小时数据发送次数.vi" "小时数据发送次数"() -> (w2894:i32)
      n1230 = global read "全局 小时数据发送次数.vi" "小时数据发送次数"() -> (w2896:i32)
      n1231 = global read "全局 小时数据发送次数.vi" "小时数据发送次数"() -> (w2895:i32)
      n1232 = global read "全局 小时数据发送次数.vi" "小时数据发送次数"() -> (w2911:i32)
      n1233 = global read "全局 小时数据发送次数.vi" "小时数据发送次数"() -> (w2897:i32)
      n1234 = global read "全局 小时数据发送次数.vi" "小时数据发送次数"() -> (w2906:i32)
      n1235 = global read "全局 小时数据发送次数.vi" "小时数据发送次数"() -> (w2914:i32)
      n1236 = global read "全局 小时数据发送次数.vi" "小时数据发送次数"() -> (w2910:i32)
      n1237 = global read "全局 小时数据发送次数.vi" "小时数据发送次数"() -> (w2903:i32)
      n1238 = Index Array(array=w2925, index (row)=w2917) -> (element=w2916:string[])  [unwired: 1 in]
      n1239 = Index Array(array=w2924, index (row)=w2919) -> (element=w2918:string[])  [unwired: 1 in]
      n1240 = Index Array(array=w2899, index (row)=w2900) -> (element=w2898:string[])  [unwired: 1 in]
      n1241 = Index Array(array=w2887, index (row)=w2894) -> (element=w2886:string[])  [unwired: 1 in]
      n1242 = Index Array(array=w2891, index (row)=w2896) -> (element=w2890:string[])  [unwired: 1 in]
      n1243 = Index Array(array=w2889, index (row)=w2895) -> (element=w2888:string[])  [unwired: 1 in]
      n1244 = Index Array(array=w2923, index (row)=w2911) -> (element=w2907:string[])  [unwired: 1 in]
      n1245 = Index Array(array=w2922, index (row)=w2915) -> (element=w2913:string[])  [unwired: 1 in]
      n1246 = Index Array(array=w2893, index (row)=w2897) -> (element=w2892:string[])  [unwired: 1 in]
      n1247 = Index Array(array=w2905, index (row)=w2906) -> (element=w2904:string[])  [unwired: 1 in]
      n1248 = Index Array(array=w2921, index (row)=w2914) -> (element=w2912:string[])  [unwired: 1 in]
      n1249 = Index Array(array=w2909, index (row)=w2910) -> (element=w2908:string[])  [unwired: 1 in]
      n1250 = Index Array(array=w2902, index (row)=w2903) -> (element=w2901:string[])  [unwired: 1 in]
      n1251 = global read "全局1.vi" "枚举"() -> (w2920:enum16{"返回请求应答", "上传数据", "返回执行结果"})
      n1252 = case shown="\"上传数据\"" w2920 {
        tunnel: ["QnRtn=1" w2991 "ExeRtn=1"] -> w2926
        tunnel: w2918 -> [_ w2954 _]
        tunnel: w2916 -> [_ w2951 _]
        tunnel: w2913 -> [_ w2957 _]
        tunnel: w2912 -> [_ w2960 _]
        tunnel: w2908 -> [_ w2963 _]
        tunnel: w2907 -> [_ w2988 _]
        tunnel: w2904 -> [_ w2984 _]
        tunnel: w2901 -> [_ w2982 _]
        tunnel: w2898 -> [_ w2980 _]
        tunnel: w2892 -> [_ w2978 _]
        tunnel: w2890 -> [_ w2976 _]
        tunnel: w2888 -> [_ w2974 _]
        tunnel: w2886 -> [_ w2972 _]
        frame "返回请求应答", Default {
          n1253 = global read "全局 数据数组大小.vi" "数据数组大小"() -> (w2929:i32)
          n1254 = Equal To 0?(x=w2929) -> (x = 0?=w2928:bool)
          n1255 = case shown="真" w2928 {
            frame False {
            }
            frame True {
              n1256 = global read "全局 小时数据发送次数.vi" "小时数据发送次数"() -> (w2931:i32)
              n1257 = Increment(x=w2931) -> (x+1=w2930:i32)
              n1258 = global write "全局 小时数据发送次数.vi" "小时数据发送次数"(w2930) -> ()
            }
          }
        }
        frame "上传数据" {
          n1259 = call "关键参数组合 (子VI).vi"("table"="3090仪器参数", "因子编码"="w21001", "DO"=w2960) -> ("字符串"=w2959:string)  [unwired: 8 in]
          n1260 = call "关键参数组合 (子VI).vi"("table"="3090仪器参数", "因子编码"="w01001", "DO"=w2984) -> ("字符串"=w2971:string)  [unwired: 8 in]
          n1261 = call "关键参数组合 (子VI).vi"("table"="3090仪器参数", "因子编码"="w01019", "DO"=w2951) -> ("字符串"=w2949:string)  [unwired: 8 in]
          n1262 = call "关键参数组合 (子VI).vi"("table"="3090仪器参数", "因子编码"="w01014", "DO"=w2982) -> ("字符串"=w2970:string)  [unwired: 8 in]
          n1263 = call "关键参数组合 (子VI).vi"("table"="3090仪器参数", "因子编码"="w01003", "DO"=w2978) -> ("字符串"=w2968:string)  [unwired: 8 in]
          n1264 = call "关键参数组合 (子VI).vi"("table"="3090仪器参数", "因子编码"="w01010", "DO"=w2980) -> ("字符串"=w2969:string)  [unwired: 8 in]
          n1265 = call "关键参数组合 (子VI).vi"("table"="3090仪器参数", "因子编码"="w01018", "DO"=w2963) -> ("字符串"=w2962:string)  [unwired: 8 in]
          n1266 = call "关键参数组合 (子VI).vi"("table"="3090仪器参数", "因子编码"="w01009", "DO"=w2988) -> ("字符串"=w2987:string)  [unwired: 8 in]
          n1267 = call "关键参数组合 (子VI).vi"("table"="3090仪器参数", "因子编码"="w21011", "DO"=w2957) -> ("字符串"=w2956:string)  [unwired: 8 in]
          n1268 = call "关键参数组合 (子VI).vi"("table"="3090仪器参数", "因子编码"="w01016", "DO"=w2976) -> ("字符串"=w2967:string)  [unwired: 8 in]
          n1269 = call "关键参数组合 (子VI).vi"("table"="3090仪器参数", "因子编码"="w21003", "DO"=w2954) -> ("字符串"=w2953:string)  [unwired: 8 in]
          n1270 = call "关键参数组合 (子VI).vi"("table"="3090仪器参数", "因子编码"="w01100", "DO"=w2972) -> ("字符串"=w2965:string)  [unwired: 8 in]
          n1271 = call "关键参数组合 (子VI).vi"("table"="3090仪器参数", "因子编码"="w19011", "DO"=w2974) -> ("字符串"=w2966:string)  [unwired: 8 in]
          n1272 = Index Array(array=w2951) -> (element=w2950:string)  [unwired: 1 in]
          n1273 = call "规范时间戳.vi"("字符串"=w2950) -> ("result string"=w2989:string)  [unwired: 10 in]
          n1274 = Format Into String(format string="DataTime=%s;%s%s%s%s%s%s%s%s%s%s%s%s%s" ("格式字符串"), w2989, w2949, w2953, w2956, w2959, w2962, w2987, w2971, w2970, w2969, w2968, w2967, w2966, w2965) -> (resulting string=w2933:string)  [unwired: 2 in, 1 out]
          n1275 = String Length(string=w2933) -> (length=w2934:i32)
          n1276 = Decrement(x=w2934) -> (x-1=w2935:i32)
          n1277 = String Subset(string=w2933, length (rest)=w2935) -> (substring=w2932:string)  [unwired: 1 in]
          n1278 = Empty String/Path?(string/path=w2932) -> (empty?=w2992:bool)
          n1279 = case shown="假" w2992 {
            tunnel: [w2995 ""] -> w2991
            tunnel: w2932 -> [w2995 _]
            frame False {
              n1280 = global read "全局 小时数据发送次数.vi" "小时数据发送次数"() -> (w2994:i32)
              n1281 = Increment(x=w2994) -> (x+1=w2993:i32)
              n1282 = global write "全局 小时数据发送次数.vi" "小时数据发送次数"(w2993) -> ()
            }
            frame True {
              n1283 = global read "全局 小时数据发送次数.vi" "小时数据发送次数"() -> (w2997:i32)
              n1284 = Increment(x=w2997) -> (x+1=w2996:i32)
              n1285 = global write "全局 小时数据发送次数.vi" "小时数据发送次数"(w2996) -> ()
            }
          }
        }
        frame "返回执行结果" {
        }
      }
    }
    frame "提取仪器参数" {
      n1286 = global read "全局 小时数据发送次数.vi" "小时数据发送次数"() -> (w3031:i32)
      n1287 = global read "全局 小时数据发送次数.vi" "小时数据发送次数"() -> (w3033:i32)
      n1288 = global read "全局 小时数据发送次数.vi" "小时数据发送次数"() -> (w3014:i32)
      n1289 = global read "全局 小时数据发送次数.vi" "小时数据发送次数"() -> (w3017:i32)
      n1290 = global read "全局 小时数据发送次数.vi" "小时数据发送次数"() -> (w3016:i32)
      n1291 = global read "全局 小时数据发送次数.vi" "小时数据发送次数"() -> (w3015:i32)
      n1292 = global read "全局 小时数据发送次数.vi" "小时数据发送次数"() -> (w3025:i32)
      n1293 = global read "全局 小时数据发送次数.vi" "小时数据发送次数"() -> (w3019:i32)
      n1294 = global read "全局 小时数据发送次数.vi" "小时数据发送次数"() -> (w3020:i32)
      n1295 = global read "全局 小时数据发送次数.vi" "小时数据发送次数"() -> (w3018:i32)
      n1296 = global read "全局 小时数据发送次数.vi" "小时数据发送次数"() -> (w3029:i32)
      n1297 = global read "全局 小时数据发送次数.vi" "小时数据发送次数"() -> (w3024:i32)
      n1298 = global read "全局 小时数据发送次数.vi" "小时数据发送次数"() -> (w3028:i32)
      n1299 = Index Array(array=w3003, index (row)=w3014) -> (element=w3000:string[])  [unwired: 1 in]
      n1300 = Index Array(array=w3007, index (row)=w3017) -> (element=w3006:string[])  [unwired: 1 in]
      n1301 = Index Array(array=w3005, index (row)=w3016) -> (element=w3002:string[])  [unwired: 1 in]
      n1302 = Index Array(array=w3004, index (row)=w3015) -> (element=w3001:string[])  [unwired: 1 in]
      n1303 = Index Array(array=w3037, index (row)=w3025) -> (element=w3021:string[])  [unwired: 1 in]
      n1304 = Index Array(array=w3012, index (row)=w3019) -> (element=w3009:string[])  [unwired: 1 in]
      n1305 = Index Array(array=w3039, index (row)=w3031) -> (element=w3030:string[])  [unwired: 1 in]
      n1306 = Index Array(array=w3013, index (row)=w3020) -> (element=w3010:string[])  [unwired: 1 in]
      n1307 = Index Array(array=w3011, index (row)=w3018) -> (element=w3008:string[])  [unwired: 1 in]
      n1308 = Index Array(array=w3038, index (row)=w3033) -> (element=w3032:string[])  [unwired: 1 in]
      n1309 = Index Array(array=w3036, index (row)=w3029) -> (element=w3027:string[])  [unwired: 1 in]
      n1310 = Index Array(array=w3023, index (row)=w3024) -> (element=w3022:string[])  [unwired: 1 in]
      n1311 = Index Array(array=w3035, index (row)=w3028) -> (element=w3026:string[])  [unwired: 1 in]
      n1312 = global read "全局1.vi" "枚举"() -> (w3034:enum16{"返回请求应答", "上传数据", "返回执行结果"})
      n1313 = case shown="\"上传数据\"" w3034 {
        tunnel: ["QnRtn=1" w3086 "ExeRtn=1"] -> w3040
        tunnel: w3032 -> [_ w3053 _]
        tunnel: w3030 -> [_ w3047 _]
        tunnel: w3027 -> [_ w3057 _]
        tunnel: w3026 -> [_ w3085 _]
        tunnel: w3022 -> [_ w3050 _]
        tunnel: w3021 -> [_ w3081 _]
        tunnel: w3010 -> [_ w3073 _]
        tunnel: w3009 -> [_ w3072 _]
        tunnel: w3008 -> [_ w3071 _]
        tunnel: w3006 -> [_ w3070 _]
        tunnel: w3002 -> [_ w3069 _]
        tunnel: w3001 -> [_ w3068 _]
        tunnel: w3000 -> [_ w3067 _]
        frame "返回请求应答", Default {
          n1314 = global read "全局 数据数组大小.vi" "数据数组大小"() -> (w3043:i32)
          n1315 = Equal To 0?(x=w3043) -> (x = 0?=w3042:bool)
          n1316 = case shown="假" w3042 {
            frame False {
            }
            frame True {
              n1317 = global read "全局 小时数据发送次数.vi" "小时数据发送次数"() -> (w3045:i32)
              n1318 = Increment(x=w3045) -> (x+1=w3044:i32)
              n1319 = global write "全局 小时数据发送次数.vi" "小时数据发送次数"(w3044) -> ()
            }
          }
        }
        frame "上传数据" {
          n1320 = call "提取仪器参数 (子VI).vi"("因子编码"="w01016", "数据输入"=w3069) -> ("字符串"=w3059:string)  [unwired: 9 in]
          n1321 = call "提取仪器参数 (子VI).vi"("因子编码"="w01100", "数据输入"=w3067) -> ("字符串"=w3061:string)  [unwired: 9 in]
          n1322 = call "提取仪器参数 (子VI).vi"("因子编码"="w01014", "数据输入"=w3071) -> ("字符串"=w3063:string)  [unwired: 9 in]
          n1323 = call "提取仪器参数 (子VI).vi"("因子编码"="w01003", "数据输入"=w3070) -> ("字符串"=w3062:string)  [unwired: 9 in]
          n1324 = call "提取仪器参数 (子VI).vi"("因子编码"="w19011", "数据输入"=w3068) -> ("字符串"=w3060:string)  [unwired: 9 in]
          n1325 = call "提取仪器参数 (子VI).vi"("因子编码"="w21011", "数据输入"=w3057) -> ("字符串"=w3055:string)  [unwired: 9 in]
          n1326 = call "提取仪器参数 (子VI).vi"("因子编码"="w01010", "数据输入"=w3072) -> ("字符串"=w3064:string)  [unwired: 9 in]
          n1327 = call "提取仪器参数 (子VI).vi"("因子编码"="w21003", "数据输入"=w3053) -> ("字符串"=w3052:string)  [unwired: 9 in]
          n1328 = call "提取仪器参数 (子VI).vi"("因子编码"="w01001", "数据输入"=w3073) -> ("字符串"=w3065:string)  [unwired: 9 in]
          n1329 = call "提取仪器参数 (子VI).vi"("因子编码"="w01009", "数据输入"=w3081) -> ("字符串"=w3066:string)  [unwired: 9 in]
          n1330 = call "提取仪器参数 (子VI).vi"("因子编码"="w21001", "数据输入"=w3085) -> ("字符串"=w3084:string)  [unwired: 9 in]
          n1331 = call "提取仪器参数 (子VI).vi"("因子编码"="w01018", "数据输入"=w3050) -> ("字符串"=w3049:string)  [unwired: 9 in]
          n1332 = call "提取仪器参数 (子VI).vi"("因子编码"="w01019", "数据输入"=w3047) -> ("字符串"=w3046:string)  [unwired: 9 in]
          n1333 = Concatenate Strings(w3066, w3065, w3064, w3063, w3062, w3059, w3060, w3061) -> (w3058:string)
          n1334 = Concatenate Strings(w3046, w3049, w3052, w3055, w3084, w3058) -> (w3087:string)
          n1335 = Empty String/Path?(string/path=w3087) -> (empty?=w3088:bool)
          n1336 = case shown="假" w3088 {
            tunnel: [w3091 ""] -> w3086
            tunnel: w3087 -> [w3091 _]
            frame False {
              n1337 = global read "全局 小时数据发送次数.vi" "小时数据发送次数"() -> (w3090:i32)
              n1338 = Increment(x=w3090) -> (x+1=w3089:i32)
              n1339 = global write "全局 小时数据发送次数.vi" "小时数据发送次数"(w3089) -> ()
            }
            frame True {
              n1340 = global read "全局 小时数据发送次数.vi" "小时数据发送次数"() -> (w3093:i32)
              n1341 = Increment(x=w3093) -> (x+1=w3092:i32)
              n1342 = global write "全局 小时数据发送次数.vi" "小时数据发送次数"(w3092) -> ()
            }
          }
        }
        frame "返回执行结果" {
        }
      }
    }
    frame "报警信息" {
      n1343 = global read "全局 小时数据发送次数.vi" "小时数据发送次数"() -> (w3104:i32)
      n1344 = global read "全局 小时数据发送次数.vi" "小时数据发送次数"() -> (w3103:i32)
      n1345 = global read "全局 小时数据发送次数.vi" "小时数据发送次数"() -> (w3110:i32)
      n1346 = global read "全局 小时数据发送次数.vi" "小时数据发送次数"() -> (w3107:i32)
      n1347 = global read "全局 小时数据发送次数.vi" "小时数据发送次数"() -> (w3102:i32)
      n1348 = global read "全局 小时数据发送次数.vi" "小时数据发送次数"() -> (w3125:i32)
      n1349 = global read "全局 小时数据发送次数.vi" "小时数据发送次数"() -> (w3113:i32)
      n1350 = global read "全局 小时数据发送次数.vi" "小时数据发送次数"() -> (w3127:i32)
      n1351 = global read "全局 小时数据发送次数.vi" "小时数据发送次数"() -> (w3117:i32)
      n1352 = global read "全局 小时数据发送次数.vi" "小时数据发送次数"() -> (w3123:i32)
      n1353 = global read "全局 小时数据发送次数.vi" "小时数据发送次数"() -> (w3122:i32)
      n1354 = global read "全局 小时数据发送次数.vi" "小时数据发送次数"() -> (w3119:i32)
      n1355 = Index Array(array=w3101, index (row)=w3104) -> (element=w3098:string[])  [unwired: 1 in]
      n1356 = Index Array(array=w3100, index (row)=w3103) -> (element=w3097:string[])  [unwired: 1 in]
      n1357 = Index Array(array=w3109, index (row)=w3110) -> (element=w3108:string[])  [unwired: 1 in]
      n1358 = Index Array(array=w3106, index (row)=w3107) -> (element=w3105:string[])  [unwired: 1 in]
      n1359 = Index Array(array=w3099, index (row)=w3102) -> (element=w3096:string[])  [unwired: 1 in]
      n1360 = Index Array(array=w3132, index (row)=w3125) -> (element=w3124:string[])  [unwired: 1 in]
      n1361 = Index Array(array=w3111, index (row)=w3113) -> (element=w3112:string[])  [unwired: 1 in]
      n1362 = Index Array(array=w3131, index (row)=w3127) -> (element=w3126:string[])  [unwired: 1 in]
      n1363 = Index Array(array=w3116, index (row)=w3117) -> (element=w3115:string[])  [unwired: 1 in]
      n1364 = Index Array(array=w3130, index (row)=w3123) -> (element=w3121:string[])  [unwired: 1 in]
      n1365 = Index Array(array=w3129, index (row)=w3122) -> (element=w3120:string[])  [unwired: 1 in]
      n1366 = global read "全局1.vi" "枚举"() -> (w3128:enum16{"返回请求应答", "上传数据", "返回执行结果"})
      n1367 = Index Array(array=w3114, index (row)=w3119) -> (element=w3118:string[])  [unwired: 1 in]
      n1368 = case shown="\"上传数据\"" w3128 {
        tunnel: ["QnRtn=1" w3208 "ExeRtn=1"] -> w3133
        tunnel: w3126 -> [_ w3227 _]
        tunnel: w3124 -> [_ w3225 _]
        tunnel: w3121 -> [_ w3224 _]
        tunnel: w3120 -> [_ w3223 _]
        tunnel: w3118 -> [_ w3221 _]
        tunnel: w3115 -> [_ w3172 _]
        tunnel: w3112 -> [_ w3169 _]
        tunnel: w3108 -> [_ w3168 _]
        tunnel: w3105 -> [_ w3167 _]
        tunnel: w3098 -> [_ w3166 _]
        tunnel: w3097 -> [_ w3165 _]
        tunnel: w3096 -> [_ w3164 _]
        frame "返回请求应答", Default {
          n1369 = global read "全局 数据数组大小.vi" "数据数组大小"() -> (w3136:i32)
          n1370 = Equal To 0?(x=w3136) -> (x = 0?=w3135:bool)
          n1371 = case shown="真" w3135 {
            frame False {
            }
            frame True {
              n1372 = global read "全局 小时数据发送次数.vi" "小时数据发送次数"() -> (w3138:i32)
              n1373 = Increment(x=w3138) -> (x+1=w3137:i32)
              n1374 = global write "全局 小时数据发送次数.vi" "小时数据发送次数"(w3137) -> ()
            }
          }
        }
        frame "上传数据" {
          n1375 = global read "全局1.vi" "register values"() -> (w3158:u16[])
          n1376 = Index Array(array=w3158, index #1=1 ("索引")) -> (element #1=w3156:u16, element #2=w3154:u16, element #3=w3152:u16, element #4=w3151:u16, element #5=w3150:u16)  [unwired: 4 in]
          n1377 = Number To Decimal String(number=w3150) -> (decimal integer string=w3147:string)  [unwired: 1 in]
          n1378 = Number To Decimal String(number=w3156) -> (decimal integer string=w3155:string)  [unwired: 1 in]
          n1379 = Number To Decimal String(number=w3154) -> (decimal integer string=w3153:string)  [unwired: 1 in]
          n1380 = Number To Decimal String(number=w3152) -> (decimal integer string=w3149:string)  [unwired: 1 in]
          n1381 = Number To Decimal String(number=w3151) -> (decimal integer string=w3148:string)  [unwired: 1 in]
          n1382 = Index Array(array=w3164, index #1=0 ("索引"), index #2=2 ("索引")) -> (element #1=w3177:string, element #2=w3175:string)
          n1383 = Index Array(array=w3166, index #1=0 ("索引"), index #2=2 ("索引")) -> (element #1=w3196:string, element #2=w3205:string)
          n1384 = Index Array(array=w3168, index #1=0 ("索引"), index #2=2 ("索引")) -> (element #1=w3194:string, element #2=w3203:string)
          n1385 = Index Array(array=w3223, index #1=0 ("索引"), index #2=2 ("索引")) -> (element #1=w3222:string, element #2=w3212:string)
          n1386 = Index Array(array=w3227, index #1=0 ("索引"), index #2=2 ("索引")) -> (element #1=w3226:string, element #2=w3214:string)
          n1387 = Empty String/Path?(string/path=w3203) -> (empty?=w3202:bool)
          n1388 = Index Array(array=w3165, index #1=0 ("索引"), index #2=2 ("索引")) -> (element #1=w3178:string, element #2=w3173:string)
          n1389 = Empty String/Path?(string/path=w3175) -> (empty?=w3176:bool)
          n1390 = Empty String/Path?(string/path=w3214) -> (empty?=w3215:bool)
          n1391 = Index Array(array=w3169, index #1=0 ("索引"), index #2=2 ("索引")) -> (element #1=w3197:string, element #2=w3201:string)
          n1392 = Index Array(array=w3167, index #1=0 ("索引"), index #2=2 ("索引")) -> (element #1=w3193:string, element #2=w3207:string)
          n1393 = Index Array(array=w3172, index #1=0 ("索引"), index #2=2 ("索引")) -> (element #1=w3195:string, element #2=w3198:string)
          n1394 = Empty String/Path?(string/path=w3205) -> (empty?=w3204:bool)
          n1395 = case shown="假" w3202 {
            tunnel: [w3359 ""] -> w3163
            tunnel: w3203 -> [w3357 _]
            tunnel: w3194 -> [_ _]
            frame False {
              # "PH"
              n1396 = case shown="\"溶解氧光强异常\"" w3357 {
                tunnel: ["0" ("输入 3") "1" ("输入 3") "2" ("输入 3") "3" ("输入 3") "4" ("输入 3") "5" ("输入 3") "6" ("输入 3") "7" ("输入 3") "8" ("输入 3") "9" ("输入 3") "10" ("输入 3") "11" ("输入 3") "12" ("输入 3") "13" ("输入 3") "14" ("输入 3") "15" ("输入 3") "16" ("输入 3") "17" ("输入 3") "18" ("输入 3") "19" ("输入 3") "20" ("输入 3") "21" ("输入 3")] -> w3356
                frame "无告警" {
                }
                frame "缺试剂告警" {
                }
                frame "缺水样告警" {
                }
                frame "缺蒸馏水告警" {
                }
                frame "缺标液告警" {
                }
                frame "仪表漏液告警" {
                }
                frame "标定异常告警" {
                }
                frame "超量程告警" {
                }
                frame "加热异常" {
                }
                frame "低试剂预警" {
                }
                frame "超上限告警" {
                }
                frame "超下限告警" {
                }
                frame "仪表内部其他异常", Default {
                }
                frame "滴定异常告警" {
                }
                frame "电极异常告警" {
                }
                frame "量程切换告警" {
                }
                frame "参数设置告警" {
                }
                frame "PH电极电位异常" {
                }
                frame "电导率电极异常" {
                }
                frame "浊度光度异常" {
                }
                frame "溶解氧电极异常" {
                }
                frame "溶解氧光强异常" {
                }
              }
              n1397 = Format Into String(format string="PolId=w01001,i12001-Info=%s,i12031-Info=%s;" ("格式字符串"), "0" ("输入 2"), w3356) -> (resulting string=w3359:string)  [unwired: 2 in, 1 out]
            }
            frame True {
            }
          }
          n1398 = Index Array(array=w3221, index #1=0 ("索引"), index #2=2 ("索引")) -> (element #1=w3220:string, element #2=w3216:string)
          n1399 = Empty String/Path?(string/path=w3201) -> (empty?=w3200:bool)
          n1400 = Index Array(array=w3224, index #1=0 ("索引"), index #2=2 ("索引")) -> (element #1=w3228:string, element #2=w3210:string)
          n1401 = Index Array(array=w3225, index #1=0 ("索引"), index #2=2 ("索引")) -> (element #1=w3139:string, element #2=w3219:string)
          n1402 = Empty String/Path?(string/path=w3212) -> (empty?=w3213:bool)
          n1403 = case shown="假" w3215 {
            tunnel: [w3505 ""] -> w3240
            tunnel: w3214 -> [w3504 _]
            tunnel: w3226 -> [_ _]
            tunnel: w3153 -> [w3502 _]
            frame False {
              # "氨氮"
              n1404 = case shown="\"溶解氧光强异常\"" w3504 {
                tunnel: ["0" ("输入 3") "1" ("输入 3") "2" ("输入 3") "3" ("输入 3") "4" ("输入 3") "5" ("输入 3") "6" ("输入 3") "7" ("输入 3") "8" ("输入 3") "9" ("输入 3") "10" ("输入 3") "11" ("输入 3") "12" ("输入 3") "13" ("输入 3") "14" ("输入 3") "15" ("输入 3") "16" ("输入 3") "17" ("输入 3") "18" ("输入 3") "19" ("输入 3") "20" ("输入 3") "21" ("输入 3")] -> w3503
                frame "无告警" {
                }
                frame "缺试剂告警" {
                }
                frame "缺水样告警" {
                }
                frame "缺蒸馏水告警" {
                }
                frame "缺标液告警" {
                }
                frame "仪表漏液告警" {
                }
                frame "标定异常告警" {
                }
                frame "超量程告警" {
                }
                frame "加热异常" {
                }
                frame "低试剂预警" {
                }
                frame "超上限告警" {
                }
                frame "超下限告警" {
                }
                frame "仪表内部其他异常", Default {
                }
                frame "滴定异常告警" {
                }
                frame "电极异常告警" {
                }
                frame "量程切换告警" {
                }
                frame "参数设置告警" {
                }
                frame "PH电极电位异常" {
                }
                frame "电导率电极异常" {
                }
                frame "浊度光度异常" {
                }
                frame "溶解氧电极异常" {
                }
                frame "溶解氧光强异常" {
                }
              }
              n1405 = Format Into String(format string="PolId=w21003,i12001-Info=%s,i12031-Info=%s;" ("格式字符串"), w3502, w3503) -> (resulting string=w3505:string)  [unwired: 2 in, 1 out]
            }
            frame True {
            }
          }
          n1406 = Empty String/Path?(string/path=w3173) -> (empty?=w3174:bool)
          n1407 = Empty String/Path?(string/path=w3216) -> (empty?=w3217:bool)
          n1408 = Empty String/Path?(string/path=w3198) -> (empty?=w3199:bool)
          n1409 = Empty String/Path?(string/path=w3207) -> (empty?=w3206:bool)
          n1410 = case shown="假" w3176 {
            tunnel: [w3275 ""] -> w3159
            tunnel: w3177 -> [_ _]
            tunnel: w3175 -> [w3273 _]
            frame False {
              # "叶绿素"
              n1411 = case shown="\"溶解氧光强异常\"" w3273 {
                tunnel: ["0" ("输入 3") "1" ("输入 3") "2" ("输入 3") "3" ("输入 3") "4" ("输入 3") "5" ("输入 3") "6" ("输入 3") "7" ("输入 3") "8" ("输入 3") "9" ("输入 3") "10" ("输入 3") "11" ("输入 3") "12" ("输入 3") "13" ("输入 3") "14" ("输入 3") "15" ("输入 3") "16" ("输入 3") "17" ("输入 3") "18" ("输入 3") "19" ("输入 3") "20" ("输入 3") "21" ("输入 3")] -> w3272
                frame "无告警" {
                }
                frame "缺试剂告警" {
                }
                frame "缺水样告警" {
                }
                frame "缺蒸馏水告警" {
                }
                frame "缺标液告警" {
                }
                frame "仪表漏液告警" {
                }
                frame "标定异常告警" {
                }
                frame "超量程告警" {
                }
                frame "加热异常" {
                }
                frame "低试剂预警" {
                }
                frame "超上限告警" {
                }
                frame "超下限告警" {
                }
                frame "仪表内部其他异常", Default {
                }
                frame "滴定异常告警" {
                }
                frame "电极异常告警" {
                }
                frame "量程切换告警" {
                }
                frame "参数设置告警" {
                }
                frame "PH电极电位异常" {
                }
                frame "电导率电极异常" {
                }
                frame "浊度光度异常" {
                }
                frame "溶解氧电极异常" {
                }
                frame "溶解氧光强异常" {
                }
              }
              n1412 = Format Into String(format string="PolId=w01016,i12001-Info=%s,i12031-Info=%s;" ("格式字符串"), "0" ("输入 2"), w3272) -> (resulting string=w3275:string)  [unwired: 2 in, 1 out]
            }
            frame True {
            }
          }
          n1413 = case shown="假" w3200 {
            tunnel: [w3388 ""] -> w3170
            tunnel: w3197 -> [_ _]
            tunnel: w3201 -> [w3385 _]
            frame False {
              # "DO"
              n1414 = case shown="\"溶解氧光强异常\"" w3385 {
                tunnel: ["0" ("输入 3") "1" ("输入 3") "2" ("输入 3") "3" ("输入 3") "4" ("输入 3") "5" ("输入 3") "6" ("输入 3") "7" ("输入 3") "8" ("输入 3") "9" ("输入 3") "10" ("输入 3") "11" ("输入 3") "12" ("输入 3") "13" ("输入 3") "14" ("输入 3") "15" ("输入 3") "16" ("输入 3") "17" ("输入 3") "18" ("输入 3") "19" ("输入 3") "20" ("输入 3") "21" ("输入 3")] -> w3384
                frame "无告警" {
                }
                frame "缺试剂告警" {
                }
                frame "缺水样告警" {
                }
                frame "缺蒸馏水告警" {
                }
                frame "缺标液告警" {
                }
                frame "仪表漏液告警" {
                }
                frame "标定异常告警" {
                }
                frame "超量程告警" {
                }
                frame "加热异常" {
                }
                frame "低试剂预警" {
                }
                frame "超上限告警" {
                }
                frame "超下限告警" {
                }
                frame "仪表内部其他异常", Default {
                }
                frame "滴定异常告警" {
                }
                frame "电极异常告警" {
                }
                frame "量程切换告警" {
                }
                frame "参数设置告警" {
                }
                frame "PH电极电位异常" {
                }
                frame "电导率电极异常" {
                }
                frame "浊度光度异常" {
                }
                frame "溶解氧电极异常" {
                }
                frame "溶解氧光强异常" {
                }
              }
              n1415 = Format Into String(format string="PolId=w01009,i22001-Info=%s,i22003-Info=%s;" ("格式字符串"), "0" ("输入 2"), w3384) -> (resulting string=w3388:string)  [unwired: 2 in, 1 out]
            }
            frame True {
            }
          }
          n1416 = Empty String/Path?(string/path=w3219) -> (empty?=w3218:bool)
          n1417 = case shown="假" w3204 {
            tunnel: [w3331 ""] -> w3161
            tunnel: w3196 -> [_ _]
            tunnel: w3205 -> [w3329 _]
            frame False {
              # "水温"
              n1418 = case shown="\"溶解氧光强异常\"" w3329 {
                tunnel: ["0" ("输入 3") "1" ("输入 3") "2" ("输入 3") "3" ("输入 3") "4" ("输入 3") "5" ("输入 3") "6" ("输入 3") "7" ("输入 3") "8" ("输入 3") "9" ("输入 3") "10" ("输入 3") "11" ("输入 3") "12" ("输入 3") "13" ("输入 3") "14" ("输入 3") "15" ("输入 3") "16" ("输入 3") "17" ("输入 3") "18" ("输入 3") "19" ("输入 3") "20" ("输入 3") "21" ("输入 3")] -> w3328
                frame "无告警" {
                }
                frame "缺试剂告警" {
                }
                frame "缺水样告警" {
                }
                frame "缺蒸馏水告警" {
                }
                frame "缺标液告警" {
                }
                frame "仪表漏液告警" {
                }
                frame "标定异常告警" {
                }
                frame "超量程告警" {
                }
                frame "加热异常" {
                }
                frame "低试剂预警" {
                }
                frame "超上限告警" {
                }
                frame "超下限告警" {
                }
                frame "仪表内部其他异常", Default {
                }
                frame "滴定异常告警" {
                }
                frame "电极异常告警" {
                }
                frame "量程切换告警" {
                }
                frame "参数设置告警" {
                }
                frame "PH电极电位异常" {
                }
                frame "电导率电极异常" {
                }
                frame "浊度光度异常" {
                }
                frame "溶解氧电极异常" {
                }
                frame "溶解氧光强异常" {
                }
              }
              n1419 = Format Into String(format string="PolId=w01010,i12001-Info=%s,i12031-Info=%s;" ("格式字符串"), "0" ("输入 2"), w3328) -> (resulting string=w3331:string)  [unwired: 2 in, 1 out]
            }
            frame True {
            }
          }
          n1420 = case shown="假" w3174 {
            tunnel: [w3248 ""] -> w3160
            tunnel: w3178 -> [_ _]
            tunnel: w3173 -> [w3245 _]
            frame False {
              # "浊度"
              n1421 = case shown="\"溶解氧光强异常\"" w3245 {
                tunnel: ["0" ("输入 3") "1" ("输入 3") "2" ("输入 3") "3" ("输入 3") "4" ("输入 3") "5" ("输入 3") "6" ("输入 3") "7" ("输入 3") "8" ("输入 3") "9" ("输入 3") "10" ("输入 3") "11" ("输入 3") "12" ("输入 3") "13" ("输入 3") "14" ("输入 3") "15" ("输入 3") "16" ("输入 3") "17" ("输入 3") "18" ("输入 3") "19" ("输入 3") "20" ("输入 3") "21" ("输入 3")] -> w3244
                frame "无告警" {
                }
                frame "缺试剂告警" {
                }
                frame "缺水样告警" {
                }
                frame "缺蒸馏水告警" {
                }
                frame "缺标液告警" {
                }
                frame "仪表漏液告警" {
                }
                frame "标定异常告警" {
                }
                frame "超量程告警" {
                }
                frame "加热异常" {
                }
                frame "低试剂预警" {
                }
                frame "超上限告警" {
                }
                frame "超下限告警" {
                }
                frame "仪表内部其他异常", Default {
                }
                frame "滴定异常告警" {
                }
                frame "电极异常告警" {
                }
                frame "量程切换告警" {
                }
                frame "参数设置告警" {
                }
                frame "PH电极电位异常" {
                }
                frame "电导率电极异常" {
                }
                frame "浊度光度异常" {
                }
                frame "溶解氧电极异常" {
                }
                frame "溶解氧光强异常" {
                }
              }
              n1422 = Format Into String(format string="PolId=w01003,i12001-Info=%s,i12031-Info=%s;" ("格式字符串"), "0" ("输入 2"), w3244) -> (resulting string=w3248:string)  [unwired: 2 in, 1 out]
            }
            frame True {
            }
          }
          n1423 = Empty String/Path?(string/path=w3210) -> (empty?=w3211:bool)
          n1424 = case shown="假" w3217 {
            tunnel: [w3534 ""] -> w3239
            tunnel: w3220 -> [_ _]
            tunnel: w3216 -> [w3531 _]
            frame False {
              # "系统日志"
              n1425 = case shown="\"仪表内部其他异常\", 默认" w3531 {
                tunnel: ["0" ("输入 3") "1" ("输入 3") "2" ("输入 3") "3" ("输入 3") "4" ("输入 3") "5" ("输入 3") "6" ("输入 3") "7" ("输入 3") "8" ("输入 3") "9" ("输入 3") "10" ("输入 3") "11" ("输入 3") "12" ("输入 3") "13" ("输入 3") "14" ("输入 3") "15" ("输入 3") "16" ("输入 3") "17" ("输入 3") "18" ("输入 3") "19" ("输入 3") "20" ("输入 3") "21" ("输入 3")] -> w3530
                frame "无告警" {
                }
                frame "缺试剂告警" {
                }
                frame "缺水样告警" {
                }
                frame "缺蒸馏水告警" {
                }
                frame "缺标液告警" {
                }
                frame "仪表漏液告警" {
                }
                frame "标定异常告警" {
                }
                frame "超量程告警" {
                }
                frame "加热异常" {
                }
                frame "低试剂预警" {
                }
                frame "超上限告警" {
                }
                frame "超下限告警" {
                }
                frame "仪表内部其他异常", Default {
                }
                frame "滴定异常告警" {
                }
                frame "电极异常告警" {
                }
                frame "量程切换告警" {
                }
                frame "参数设置告警" {
                }
                frame "PH电极电位异常" {
                }
                frame "电导率电极异常" {
                }
                frame "浊度光度异常" {
                }
                frame "溶解氧电极异常" {
                }
                frame "溶解氧光强异常" {
                }
              }
              n1426 = Format Into String(format string="PolId=w00000,i22001-Info=%s,i22003-Info=%s;" ("格式字符串"), "0" ("输入 2"), w3530) -> (resulting string=w3534:string)  [unwired: 2 in, 1 out]
            }
            frame True {
            }
          }
          n1427 = case shown="假" w3206 {
            tunnel: [w3304 ""] -> w3162
            tunnel: w3193 -> [_ _]
            tunnel: w3207 -> [w3301 _]
            frame False {
              # "比电导率"
              n1428 = case shown="\"溶解氧光强异常\"" w3301 {
                tunnel: ["0" ("输入 3") "1" ("输入 3") "2" ("输入 3") "3" ("输入 3") "4" ("输入 3") "5" ("输入 3") "6" ("输入 3") "7" ("输入 3") "8" ("输入 3") "9" ("输入 3") "10" ("输入 3") "11" ("输入 3") "12" ("输入 3") "13" ("输入 3") "14" ("输入 3") "15" ("输入 3") "16" ("输入 3") "17" ("输入 3") "18" ("输入 3") "19" ("输入 3") "20" ("输入 3") "21" ("输入 3")] -> w3300
                frame "无告警" {
                }
                frame "缺试剂告警" {
                }
                frame "缺水样告警" {
                }
                frame "缺蒸馏水告警" {
                }
                frame "缺标液告警" {
                }
                frame "仪表漏液告警" {
                }
                frame "标定异常告警" {
                }
                frame "超量程告警" {
                }
                frame "加热异常" {
                }
                frame "低试剂预警" {
                }
                frame "超上限告警" {
                }
                frame "超下限告警" {
                }
                frame "仪表内部其他异常", Default {
                }
                frame "滴定异常告警" {
                }
                frame "电极异常告警" {
                }
                frame "量程切换告警" {
                }
                frame "参数设置告警" {
                }
                frame "PH电极电位异常" {
                }
                frame "电导率电极异常" {
                }
                frame "浊度光度异常" {
                }
                frame "溶解氧电极异常" {
                }
                frame "溶解氧光强异常" {
                }
              }
              n1429 = Format Into String(format string="PolId=w01014,i12001-Info=%s,i12031-Info=%s;" ("格式字符串"), "0" ("输入 2"), w3300) -> (resulting string=w3304:string)  [unwired: 2 in, 1 out]
            }
            frame True {
            }
          }
          n1430 = case shown="假" w3213 {
            tunnel: [w3477 ""] -> w3235
            tunnel: w3222 -> [_ _]
            tunnel: w3212 -> [w3476 _]
            tunnel: w3148 -> [w3474 _]
            frame False {
              # "总氮"
              n1431 = case shown="\"溶解氧光强异常\"" w3476 {
                tunnel: ["0" ("输入 3") "1" ("输入 3") "2" ("输入 3") "3" ("输入 3") "4" ("输入 3") "5" ("输入 3") "6" ("输入 3") "7" ("输入 3") "8" ("输入 3") "9" ("输入 3") "10" ("输入 3") "11" ("输入 3") "12" ("输入 3") "13" ("输入 3") "14" ("输入 3") "15" ("输入 3") "16" ("输入 3") "17" ("输入 3") "18" ("输入 3") "19" ("输入 3") "20" ("输入 3") "21" ("输入 3")] -> w3475
                frame "无告警" {
                }
                frame "缺试剂告警" {
                }
                frame "缺水样告警" {
                }
                frame "缺蒸馏水告警" {
                }
                frame "缺标液告警" {
                }
                frame "仪表漏液告警" {
                }
                frame "标定异常告警" {
                }
                frame "超量程告警" {
                }
                frame "加热异常" {
                }
                frame "低试剂预警" {
                }
                frame "超上限告警" {
                }
                frame "超下限告警" {
                }
                frame "仪表内部其他异常", Default {
                }
                frame "滴定异常告警" {
                }
                frame "电极异常告警" {
                }
                frame "量程切换告警" {
                }
                frame "参数设置告警" {
                }
                frame "PH电极电位异常" {
                }
                frame "电导率电极异常" {
                }
                frame "浊度光度异常" {
                }
                frame "溶解氧电极异常" {
                }
                frame "溶解氧光强异常" {
                }
              }
              n1432 = Format Into String(format string="PolId=w21001,i12001-Info=%s,i12031-Info=%s;" ("格式字符串"), w3474, w3475) -> (resulting string=w3477:string)  [unwired: 2 in, 1 out]
            }
            frame True {
            }
          }
          n1433 = case shown="假" w3199 {
            tunnel: [w3415 ""] -> w3171
            tunnel: w3195 -> [_ _]
            tunnel: w3198 -> [w3413 _]
            tunnel: w3147 -> [w3412 _]
            frame False {
              # "CODCr"
              n1434 = case shown="\"溶解氧光强异常\"" w3413 {
                tunnel: ["0" ("输入 3") "1" ("输入 3") "2" ("输入 3") "3" ("输入 3") "4" ("输入 3") "5" ("输入 3") "6" ("输入 3") "7" ("输入 3") "8" ("输入 3") "9" ("输入 3") "10" ("输入 3") "11" ("输入 3") "12" ("输入 3") "13" ("输入 3") "14" ("输入 3") "15" ("输入 3") "16" ("输入 3") "17" ("输入 3") "18" ("输入 3") "19" ("输入 3") "20" ("输入 3") "21" ("输入 3")] -> w3414
                frame "无告警" {
                }
                frame "缺试剂告警" {
                }
                frame "缺水样告警" {
                }
                frame "缺蒸馏水告警" {
                }
                frame "缺标液告警" {
                }
                frame "仪表漏液告警" {
                }
                frame "标定异常告警" {
                }
                frame "超量程告警" {
                }
                frame "加热异常" {
                }
                frame "低试剂预警" {
                }
                frame "超上限告警" {
                }
                frame "超下限告警" {
                }
                frame "仪表内部其他异常", Default {
                }
                frame "滴定异常告警" {
                }
                frame "电极异常告警" {
                }
                frame "量程切换告警" {
                }
                frame "参数设置告警" {
                }
                frame "PH电极电位异常" {
                }
                frame "电导率电极异常" {
                }
                frame "浊度光度异常" {
                }
                frame "溶解氧电极异常" {
                }
                frame "溶解氧光强异常" {
                }
              }
              n1435 = Format Into String(format string="PolId=w01018,i12001-Info=%s,i12031-Info=%s;" ("格式字符串"), w3412, w3414) -> (resulting string=w3415:string)  [unwired: 2 in, 1 out]
            }
            frame True {
            }
          }
          n1436 = case shown="假" w3211 {
            tunnel: [w3450 ""] -> w3236
            tunnel: w3228 -> [_ _]
            tunnel: w3210 -> [w3448 _]
            tunnel: w3149 -> [w3446 _]
            frame False {
              # "总磷"
              n1437 = case shown="\"溶解氧光强异常\"" w3448 {
                tunnel: ["0" ("输入 3") "1" ("输入 3") "2" ("输入 3") "3" ("输入 3") "4" ("输入 3") "5" ("输入 3") "6" ("输入 3") "7" ("输入 3") "8" ("输入 3") "9" ("输入 3") "10" ("输入 3") "11" ("输入 3") "12" ("输入 3") "13" ("输入 3") "14" ("输入 3") "15" ("输入 3") "16" ("输入 3") "17" ("输入 3") "18" ("输入 3") "19" ("输入 3") "20" ("输入 3") "21" ("输入 3")] -> w3447
                frame "无告警" {
                }
                frame "缺试剂告警" {
                }
                frame "缺水样告警" {
                }
                frame "缺蒸馏水告警" {
                }
                frame "缺标液告警" {
                }
                frame "仪表漏液告警" {
                }
                frame "标定异常告警" {
                }
                frame "超量程告警" {
                }
                frame "加热异常" {
                }
                frame "低试剂预警" {
                }
                frame "超上限告警" {
                }
                frame "超下限告警" {
                }
                frame "仪表内部其他异常", Default {
                }
                frame "滴定异常告警" {
                }
                frame "电极异常告警" {
                }
                frame "量程切换告警" {
                }
                frame "参数设置告警" {
                }
                frame "PH电极电位异常" {
                }
                frame "电导率电极异常" {
                }
                frame "浊度光度异常" {
                }
                frame "溶解氧电极异常" {
                }
                frame "溶解氧光强异常" {
                }
              }
              n1438 = Format Into String(format string="PolId=w21011,i12001-Info=%s,i12031-Info=%s;" ("格式字符串"), w3446, w3447) -> (resulting string=w3450:string)  [unwired: 2 in, 1 out]
            }
            frame True {
            }
          }
          n1439 = case shown="假" w3218 {
            tunnel: [w3561 ""] -> w3241
            tunnel: w3139 -> [_ _]
            tunnel: w3219 -> [w3559 _]
            tunnel: w3155 -> [w3558 _]
            frame False {
              # "高锰酸钾盐"
              n1440 = case shown="\"缺试剂告警\"" w3559 {
                tunnel: ["0" ("输入 3") "1" ("输入 3") "2" ("输入 3") "3" ("输入 3") "4" ("输入 3") "5" ("输入 3") "6" ("输入 3") "7" ("输入 3") "8" ("输入 3") "9" ("输入 3") "10" ("输入 3") "11" ("输入 3") "12" ("输入 3") "13" ("输入 3") "14" ("输入 3") "15" ("输入 3") "16" ("输入 3") "17" ("输入 3") "18" ("输入 3") "19" ("输入 3") "20" ("输入 3") "21" ("输入 3")] -> w3560
                frame "无告警" {
                }
                frame "缺试剂告警" {
                }
                frame "缺水样告警" {
                }
                frame "缺蒸馏水告警" {
                }
                frame "缺标液告警" {
                }
                frame "仪表漏液告警" {
                }
                frame "标定异常告警" {
                }
                frame "超量程告警" {
                }
                frame "加热异常" {
                }
                frame "低试剂预警" {
                }
                frame "超上限告警" {
                }
                frame "超下限告警" {
                }
                frame "仪表内部其他异常", Default {
                }
                frame "滴定异常告警" {
                }
                frame "电极异常告警" {
                }
                frame "量程切换告警" {
                }
                frame "参数设置告警" {
                }
                frame "PH电极电位异常" {
                }
                frame "电导率电极异常" {
                }
                frame "浊度光度异常" {
                }
                frame "溶解氧电极异常" {
                }
                frame "溶解氧光强异常" {
                }
              }
              n1441 = Format Into String(format string="PolId=w01019,i12001-Info=%s,i12031-Info=%s;" ("格式字符串"), w3558, w3560) -> (resulting string=w3561:string)  [unwired: 2 in, 1 out]
            }
            frame True {
            }
          }
          n1442 = call "规范时间戳.vi"("字符串"=w3139) -> ("result string"=w3141:string)  [unwired: 10 in]
          n1443 = Format Into String(format string="DataTime=%s;", w3141) -> (resulting string=w3140:string)  [unwired: 2 in, 1 out]
          n1444 = Concatenate Strings(w3140, w3241, w3240, w3239, w3236, w3235, w3171, w3170, w3163, w3162, w3161, w3160, w3159) -> (w3144:string)
          n1445 = Empty String/Path?(string/path=w3144) -> (empty?=w3209:bool)
          n1446 = String Length(string=w3144) -> (length=w3146:i32)
          n1447 = Decrement(x=w3146) -> (x-1=w3145:i32)
          n1448 = String Subset(string=w3144, length (rest)=w3145) -> (substring=w3143:string)  [unwired: 1 in]
          n1449 = case shown="假" w3209 {
            tunnel: [w3442 ""] -> w3208
            tunnel: w3143 -> [w3442 _]
            frame False {
              n1450 = global read "全局 小时数据发送次数.vi" "小时数据发送次数"() -> (w3441:i32)
              n1451 = Increment(x=w3441) -> (x+1=w3440:i32)
              n1452 = global write "全局 小时数据发送次数.vi" "小时数据发送次数"(w3440) -> ()
            }
            frame True {
              n1453 = global read "全局 小时数据发送次数.vi" "小时数据发送次数"() -> (w3444:i32)
              n1454 = Increment(x=w3444) -> (x+1=w3443:i32)
              n1455 = global write "全局 小时数据发送次数.vi" "小时数据发送次数"(w3443) -> ()
            }
          }
        }
        frame "返回执行结果" {
        }
      }
    }
    frame "系统状态" {
      # "DataTime=20100301145000;PolId=w01018,i12001-Info=1,i12003-Info=0"
      # "100  当前模式\n101  CODMn状态  （0待机，1运行）\n102  氨氮状态\n103  总磷状态\n104  总氮状态\n105  CODCr状态\n106  运行周期"
      n1456 = global read "全局1.vi" "register values"() -> (w3615:u16[])
      n1457 = Index Array(array=w3615, index #1=1 ("索引")) -> (element #1=w3611:u16, element #2=w3607:u16, element #3=w3601:u16, element #4=w3600:u16, element #5=w3596:u16)  [unwired: 4 in]
      n1458 = Number To Decimal String(number=w3611) -> (decimal integer string=w3610:string)  [unwired: 1 in]
      n1459 = Number To Decimal String(number=w3596) -> (decimal integer string=w3598:string)  [unwired: 1 in]
      n1460 = Number To Decimal String(number=w3601) -> (decimal integer string=w3602:string)  [unwired: 1 in]
      n1461 = Number To Decimal String(number=w3607) -> (decimal integer string=w3606:string)  [unwired: 1 in]
      n1462 = Number To Decimal String(number=w3600) -> (decimal integer string=w3599:string)  [unwired: 1 in]
      n1463 = Format Into String(format string="PolId=w01019,i12001-Info=%s;" ("格式字符串"), w3610) -> (resulting string=w3609:string)  [unwired: 2 in, 1 out]
      n1464 = Format Into String(format string="PolId=w01018,i12001-Info=%s;" ("格式字符串"), w3598) -> (resulting string=w3593:string)  [unwired: 2 in, 1 out]
      n1465 = Format Into String(format string="PolId=w21003,i12001-Info=%s;" ("格式字符串"), w3606) -> (resulting string=w3605:string)  [unwired: 2 in, 1 out]
      n1466 = Format Into String(format string="PolId=w21011,i12001-Info=%s;" ("格式字符串"), w3602) -> (resulting string=w3595:string)  [unwired: 2 in, 1 out]
      n1467 = Format Into String(format string="PolId=w21001,i12001-Info=%s;" ("格式字符串"), w3599) -> (resulting string=w3594:string)  [unwired: 2 in, 1 out]
      n1468 = Get Date/Time In Seconds() -> (seconds since 1Jan1904=w3613:timestamp)
      n1469 = Format Date/Time String(time format string (%c)="%Y%m%d%H%M%S" ("时间格式字符串(%c)"), seconds (now)=w3613) -> (date/time string=w3591:string)  [unwired: 1 in]
      n1470 = Format Into String(format string="DataTime=%s;%s%s%s%s%s" ("格式字符串"), w3591, w3609, w3605, w3595, w3594, w3593) -> (resulting string=w3588:string)  [unwired: 2 in, 1 out]
      n1471 = String Length(string=w3588) -> (length=w3590:i32)
      n1472 = Decrement(x=w3590) -> (x-1=w3589:i32)
      n1473 = String Subset(string=w3588, length (rest)=w3589) -> (substring=w3587:string)  [unwired: 1 in]
    }
    frame "运行模式" {
      # "DataTime=20100301145000;PolId=w01018,i12001-Info=1,i12003-Info=0"
      # "100  当前模式\n101  CODMn状态  （0待机，1运行）\n102  氨氮状态\n103  总磷状态\n104  总氮状态\n105  CODCr状态\n106  运行周期"
      n1474 = global read "全局1.vi" "register values"() -> (w3626:u16[])
      n1475 = Index Array(array=w3626, index=0 ("索引")) -> (element=w3618:u16)
      n1476 = Number To Decimal String(number=w3618) -> (decimal integer string=w3620:string)  [unwired: 1 in]
      n1477 = Format Into String(format string="RunMode=%s;" ("格式字符串"), w3620) -> (resulting string=w3617:string)  [unwired: 2 in, 1 out]
      n1478 = Get Date/Time In Seconds() -> (seconds since 1Jan1904=w3624:timestamp)
      n1479 = Format Date/Time String(time format string (%c)="%Y%m%d%H%M%S" ("时间格式字符串(%c)"), seconds (now)=w3624) -> (date/time string=w3621:string)  [unwired: 1 in]
      n1480 = Format Into String(format string="DataTime=%s;%s" ("格式字符串"), w3621, w3617) -> (resulting string=w3623:string)  [unwired: 2 in, 1 out]
    }
    frame "测量周期" {
      # "DataTime=20100301145000;PolId=w01018,i12001-Info=1,i12003-Info=0"
      # "100  当前模式\n101  CODMn状态  （0待机，1运行）\n102  氨氮状态\n103  总磷状态\n104  总氮状态\n105  CODCr状态\n106  运行周期"
      n1481 = global read "全局1.vi" "register values"() -> (w3637:u16[])
      n1482 = Index Array(array=w3637, index=6 ("索引")) -> (element=w3629:u16)
      n1483 = Number To Decimal String(number=w3629) -> (decimal integer string=w3630:string)  [unwired: 1 in]
      n1484 = Format Into String(format string="RunInterval=%s;" ("格式字符串"), w3630) -> (resulting string=w3628:string)  [unwired: 2 in, 1 out]
      n1485 = Get Date/Time In Seconds() -> (seconds since 1Jan1904=w3635:timestamp)
      n1486 = Format Date/Time String(time format string (%c)="%Y%m%d%H%M%S" ("时间格式字符串(%c)"), seconds (now)=w3635) -> (date/time string=w3632:string)  [unwired: 1 in]
      n1487 = Format Into String(format string="DataTime=%s;%s" ("格式字符串"), w3632, w3628) -> (resulting string=w3634:string)  [unwired: 2 in, 1 out]
    }
    frame "超标留样" {
      # "DataTime=20100301145000;PolId=w01018,i12001-Info=1,i12003-Info=0"
      # "100  当前模式\n101  CODMn状态  （0待机，1运行）\n102  氨氮状态\n103  总磷状态\n104  总氮状态\n105  CODCr状态\n106  运行周期"
      n1488 = global read "全局1.vi" "register values"() -> (w3648:u16[])
      n1489 = Index Array(array=w3648, index=7 ("索引")) -> (element=w3640:u16)
      n1490 = Number To Decimal String(number=w3640) -> (decimal integer string=w3641:string)  [unwired: 1 in]
      n1491 = Format Into String(format string="VaseNo=%s;" ("格式字符串"), w3641) -> (resulting string=w3639:string)  [unwired: 2 in, 1 out]
      n1492 = Get Date/Time In Seconds() -> (seconds since 1Jan1904=w3646:timestamp)
      n1493 = Format Date/Time String(time format string (%c)="%Y%m%d%H%M%S" ("时间格式字符串(%c)"), seconds (now)=w3646) -> (date/time string=w3643:string)  [unwired: 1 in]
      n1494 = Format Into String(format string="DataTime=%s;%s" ("格式字符串"), w3643, w3639) -> (resulting string=w3645:string)  [unwired: 2 in, 1 out]
    }
  }
  n1495 = Equal?(x="table输入", y="反控命令") -> (x = y?=w44:bool)
  n1496 = case shown="假" w44 {
    tunnel: [w3651 w3655] -> w46
    frame False {
      n1497 = global read "全局1.vi" "枚举"() -> (w3650:enum16{"返回请求应答", "上传数据", "返回执行结果"})
      n1498 = case shown="\"上传数据\"" w3650 {
        tunnel: ["91" ("CN") w3653 "91" ("CN")] -> w3651
        frame "返回请求应答", Default {
        }
        frame "上传数据" {
          n1499 = global read "全局1.vi" "系统编码ST"() -> (w3653:string)
        }
        frame "返回执行结果" {
        }
      }
    }
    frame True {
      n1500 = global read "全局 反控命令枚举.vi" "反控命令枚举"() -> (w3656:enum16{"返回请求应答", "返回执行结果"})
      n1501 = case shown="\"返回执行结果\"" w3656 {
        tunnel: ["91" "91"] -> w3655
        frame "返回请求应答", Default {
        }
        frame "返回执行结果" {
        }
      }
    }
  }
  n1502 = case shown="\"小时数据\"" "table输入" {
    tunnel: ["9015" ("ST") w3669 w3677 w3685 w3692 w3699 w3707 w3715 w3724 w3739 w3747 w3755 w3764 w3773 w3790 w3798 w3806 w3814 w3822 w3830 w3841 w3853 w3861 "3020" ("ST") "3042" ("ST") "3056" ("ST") "3015" ("ST")] -> w50
    tunnel: ["9" ("ST") "8" ("ST") "8" ("ST") "8" ("ST") "8" ("ST") "8" ("ST") "8" ("ST") "8" ("ST") "9" ("ST") "9" ("ST") "9" ("ST") "9" ("ST") w3767 "8" ("ST") "9" ("ST") "8" ("ST") "8" ("ST") "9" ("ST") "9" ("ST") "8" ("ST") "9" ("ST") "9" ("ST") "8" ("ST") "9" ("ST") "9" ("ST") "9" ("ST") "9" ("ST")] -> w49
    tunnel: w35 -> [_ w3667 w3675 w3686 w3693 w3700 w3708 w3716 w3725 w3741 w3749 w3757 w3766 w3776 w3792 w3800 w3808 w3816 w3824 w3832 w3843 w3855 w3863 w3869 w3873 w3877 w3881]
    tunnel: [_ w3667 w3675 w3686 w3693 w3700 w3708 w3716 w3725 w3741 w3749 w3757 w3766 w3776 w3792 w3800 w3808 w3816 w3824 w3832 w3843 w3855 w3863 w3869 w3873 w3877 w3881] -> w48
    tunnel: [w3659 w3666 w3674 w3682 w3690 w3697 w3705 w3713 w3721 w3738 w3746 w3754 w3763 w3775 w3788 w3796 w3804 w3812 w3820 w3828 w3836 w3848 w3860 w3868 w3872 w3876 w3880] -> w36
    frame "心跳包", Default {
      # "心跳包"
      n1503 = Get Date/Time In Seconds() -> (seconds since 1Jan1904=w3662:timestamp)
      n1504 = Format Date/Time String(time format string (%c)="%Y%m%d%H%M%S%3u" ("时间格式字符串(%c)"), seconds (now)=w3662) -> (date/time string=w3661:string)  [unwired: 1 in]
      n1505 = Search and Replace String(input string=w3661, search string="." ("搜索字符串")) -> (result string=w3659:string)  [unwired: 6 in, 3 out]
    }
    frame "提取数采仪时间" {
      n1506 = global read "全局1.vi" "枚举"() -> (w3670:enum16{"返回请求应答", "上传数据", "返回执行结果"})
      n1507 = case shown="\"返回执行结果\"" w3670 {
        tunnel: ["9011" ("CN") "1014" ("CN") "9012" ("CN")] -> w3669
        frame "返回请求应答", Default {
        }
        frame "上传数据" {
        }
        frame "返回执行结果" {
        }
      }
      n1508 = local read "QN"() -> (w3666:string)
    }
    frame "提取实时数据间隔" {
      n1509 = global read "全局1.vi" "枚举"() -> (w3678:enum16{"返回请求应答", "上传数据", "返回执行结果"})
      n1510 = case shown="\"上传数据\"" w3678 {
        tunnel: ["9011" ("CN") "1061" ("CN") "9012" ("CN")] -> w3677
        frame "返回请求应答", Default {
        }
        frame "上传数据" {
        }
        frame "返回执行结果" {
        }
      }
      n1511 = local read "QN"() -> (w3674:string)
    }
    frame "反控命令" {
      n1512 = global read "全局 反控命令枚举.vi" "反控命令枚举"() -> (w3683:enum16{"返回请求应答", "返回执行结果"})
      n1513 = case shown="\"返回请求应答\", 默认" w3683 {
        tunnel: ["9011" ("CN") "9012" ("CN")] -> w3685
        frame "返回请求应答", Default {
        }
        frame "返回执行结果" {
        }
      }
      n1514 = local read "QN"() -> (w3682:string)
    }
    frame "超标留样返回" {
      n1515 = global read "全局1.vi" "枚举"() -> (w3689:enum16{"返回请求应答", "上传数据", "返回执行结果"})
      n1516 = case shown="\"上传数据\"" w3689 {
        tunnel: ["9011" ("CN") "3015" ("CN") "9012" ("CN")] -> w3692
        frame "返回请求应答", Default {
        }
        frame "上传数据" {
        }
        frame "返回执行结果" {
        }
      }
      n1517 = local read "QN"() -> (w3690:string)
    }
    frame "提取经纬度环境信息" {
      n1518 = global read "全局1.vi" "枚举"() -> (w3701:enum16{"返回请求应答", "上传数据", "返回执行结果"})
      n1519 = case shown="\"上传数据\"" w3701 {
        tunnel: ["9011" ("CN") "3041" ("CN") "9012" ("CN")] -> w3699
        frame "返回请求应答", Default {
        }
        frame "上传数据" {
        }
        frame "返回执行结果" {
        }
      }
      n1520 = local read "QN"() -> (w3697:string)
    }
    frame "提取现场系统信息" {
      n1521 = global read "全局1.vi" "枚举"() -> (w3709:enum16{"返回请求应答", "上传数据", "返回执行结果"})
      n1522 = case shown="\"上传数据\"" w3709 {
        tunnel: ["9011" ("CN") "3040" ("CN") "9012" ("CN")] -> w3707
        frame "返回请求应答", Default {
        }
        frame "上传数据" {
        }
        frame "返回执行结果" {
        }
      }
      n1523 = local read "QN"() -> (w3705:string)
    }
    frame "提取监测仪表时间" {
      n1524 = global read "全局1.vi" "枚举"() -> (w3717:enum16{"返回请求应答", "上传数据", "返回执行结果"})
      n1525 = case shown="\"返回执行结果\"" w3717 {
        tunnel: ["9011" ("CN") "1011" ("CN") "9012" ("CN")] -> w3715
        frame "返回请求应答", Default {
        }
        frame "上传数据" {
        }
        frame "返回执行结果" {
        }
      }
      n1526 = local read "QN"() -> (w3713:string)
    }
    frame "实时数据" {
      n1527 = global read "全局1.vi" "枚举"() -> (w3723:enum16{"返回请求应答", "上传数据", "返回执行结果"})
      n1528 = case shown="\"上传数据\"" w3723 {
        tunnel: ["9011" ("CN") w3728 "9012" ("CN")] -> w3724
        frame "返回请求应答", Default {
        }
        frame "上传数据" {
          n1529 = global read "全局 实时数据参数.vi" "实时数据参数"() -> (w3727:string)
          n1530 = case shown="\"平行样测试\"" w3727 {
            tunnel: ["2011" ("CN") "2064" ("CN") "2082" ("CN") "2063" ("CN") "2062" ("CN") "2065" ("CN") "2066" ("CN") "fff" ("CN")] -> w3728
            frame "水样测试", Default {
            }
            frame "平行样测试" {
            }
            frame "集成干预测试" {
            }
            frame "加标回收测试" {
            }
            frame "核查数据" {
            }
            frame "空白测试" {
            }
            frame "跨度核查" {
            }
            frame "" {
            }
          }
        }
        frame "返回执行结果" {
        }
      }
      n1531 = local read "QN"() -> (w3721:string)
    }
    frame "小时数据" {
      # "监测小时数据"
      n1532 = global read "全局1.vi" "枚举"() -> (w3740:enum16{"返回请求应答", "上传数据", "返回执行结果"})
      n1533 = case shown="\"上传数据\"" w3740 {
        tunnel: ["9011" ("CN") "2061" ("CN") "9012" ("CN")] -> w3739
        frame "返回请求应答", Default {
        }
        frame "上传数据" {
        }
        frame "返回执行结果" {
        }
      }
      n1534 = local read "QN"() -> (w3738:string)
    }
    frame "剖面多参数H" {
      # "监测小时数据"
      n1535 = global read "全局1.vi" "枚举"() -> (w3748:enum16{"返回请求应答", "上传数据", "返回执行结果"})
      n1536 = case shown="\"上传数据\"" w3748 {
        tunnel: ["9011" ("CN") "2061" ("CN") "9012" ("CN")] -> w3747
        frame "返回请求应答", Default {
        }
        frame "上传数据" {
        }
        frame "返回执行结果" {
        }
      }
      n1537 = local read "QN"() -> (w3746:string)
    }
    frame "剖面多参数S" {
      # "监测小时数据"
      n1538 = global read "全局1.vi" "枚举"() -> (w3756:enum16{"返回请求应答", "上传数据", "返回执行结果"})
      n1539 = case shown="\"上传数据\"" w3756 {
        tunnel: ["9011" ("CN") "2011" ("CN") "9012" ("CN")] -> w3755
        frame "返回请求应答", Default {
        }
        frame "上传数据" {
        }
        frame "返回执行结果" {
        }
      }
      n1540 = local read "QN"() -> (w3754:string)
    }
    frame "提取小时数据" {
      # "监测小时数据"
      n1541 = global read "断电保存全局.vi" "数据组合发送"() -> (w3762:bool)
      n1542 = global read "全局1.vi" "枚举"() -> (w3765:enum16{"返回请求应答", "上传数据", "返回执行结果"})
      n1543 = case shown="\"上传数据\"" w3765 {
        tunnel: ["9011" ("CN") "2061" ("CN") "9012" ("CN")] -> w3764
        frame "返回请求应答", Default {
        }
        frame "上传数据" {
        }
        frame "返回执行结果" {
        }
      }
      n1544 = case shown="真" w3762 {
        tunnel: ["8" ("ST") "9" ("ST")] -> w3767
        frame False {
        }
        frame True {
        }
      }
      n1545 = local read "QN"() -> (w3763:string)
    }
    frame "提取实时数据" {
      # "提取实时数据"
      n1546 = global read "全局1.vi" "枚举"() -> (w3774:enum16{"返回请求应答", "上传数据", "返回执行结果"})
      n1547 = case shown="\"上传数据\"" w3774 {
        tunnel: ["9011" ("CN") w3780 "9012" ("CN")] -> w3773
        frame "返回请求应答", Default {
        }
        frame "上传数据" {
          n1548 = global read "全局 实时数据参数.vi" "实时数据参数"() -> (w3779:string)
          n1549 = case shown="\"平行样测试\"" w3779 {
            tunnel: ["2011" ("CN") "2064" ("CN") "2063" ("CN") "2065" ("CN") "2066" ("CN") "fff" ("CN")] -> w3780
            frame "水样测试", Default {
            }
            frame "平行样测试" {
            }
            frame "加标回收测试" {
            }
            frame "空白测试" {
            }
            frame "跨度核查" {
            }
            frame "" {
            }
          }
        }
        frame "返回执行结果" {
        }
      }
      n1550 = local read "QN"() -> (w3775:string)
    }
    frame "跨度核查" {
      # "跨度核查"
      n1551 = global read "全局1.vi" "枚举"() -> (w3791:enum16{"返回请求应答", "上传数据", "返回执行结果"})
      n1552 = case shown="\"上传数据\"" w3791 {
        tunnel: ["9011" ("CN") "2066" ("ST") "9012" ("CN")] -> w3790
        frame "返回请求应答", Default {
        }
        frame "上传数据" {
        }
        frame "返回执行结果" {
        }
      }
      n1553 = local read "QN"() -> (w3788:string)
    }
    frame "提取加标回收" {
      # "提取加标回收"
      n1554 = global read "全局1.vi" "枚举"() -> (w3799:enum16{"返回请求应答", "上传数据", "返回执行结果"})
      n1555 = case shown="\"上传数据\"" w3799 {
        tunnel: ["9011" ("CN") "2063" ("ST") "9012" ("CN")] -> w3798
        frame "返回请求应答", Default {
        }
        frame "上传数据" {
        }
        frame "返回执行结果" {
        }
      }
      n1556 = local read "QN"() -> (w3796:string)
    }
    frame "提取平行样" {
      # "提取平行样"
      n1557 = global read "全局1.vi" "枚举"() -> (w3807:enum16{"返回请求应答", "上传数据", "返回执行结果"})
      n1558 = case shown="\"上传数据\"" w3807 {
        tunnel: ["9011" ("CN") "2064" ("ST") "9012" ("CN")] -> w3806
        frame "返回请求应答", Default {
        }
        frame "上传数据" {
        }
        frame "返回执行结果" {
        }
      }
      n1559 = local read "QN"() -> (w3804:string)
    }
    frame "空白测试", "零点核查" {
      # "零点核查"
      n1560 = global read "全局1.vi" "枚举"() -> (w3815:enum16{"返回请求应答", "上传数据", "返回执行结果"})
      n1561 = case shown="\"上传数据\"" w3815 {
        tunnel: ["9011" ("CN") "2065" ("ST") "9012" ("CN")] -> w3814
        frame "返回请求应答", Default {
        }
        frame "上传数据" {
        }
        frame "返回执行结果" {
        }
      }
      n1562 = local read "QN"() -> (w3812:string)
    }
    frame "核查数据" {
      # "核查数据"
      n1563 = global read "全局1.vi" "枚举"() -> (w3823:enum16{"返回请求应答", "上传数据", "返回执行结果"})
      n1564 = case shown="\"上传数据\"" w3823 {
        tunnel: ["9011" ("CN") "2062" ("ST") "9012" ("CN")] -> w3822
        frame "返回请求应答", Default {
        }
        frame "上传数据" {
        }
        frame "返回执行结果" {
        }
      }
      n1565 = local read "QN"() -> (w3820:string)
    }
    frame "提取集成干预" {
      # "核查数据"
      n1566 = global read "全局1.vi" "枚举"() -> (w3831:enum16{"返回请求应答", "上传数据", "返回执行结果"})
      n1567 = case shown="\"上传数据\"" w3831 {
        tunnel: ["9011" ("CN") "2082" ("ST") "9012" ("CN")] -> w3830
        frame "返回请求应答", Default {
        }
        frame "上传数据" {
        }
        frame "返回执行结果" {
        }
      }
      n1568 = local read "QN"() -> (w3828:string)
    }
    frame "报警信息", "操作日志", "仪器参数" {
      n1569 = global read "全局1.vi" "枚举"() -> (w3842:enum16{"返回请求应答", "上传数据", "返回执行结果"})
      n1570 = case shown="\"上传数据\"" w3842 {
        tunnel: ["9011" ("CN") "3020" ("CN") "9012" ("CN")] -> w3841
        frame "返回请求应答", Default {
        }
        frame "上传数据" {
        }
        frame "返回执行结果" {
        }
      }
      n1571 = Get Date/Time In Seconds() -> (seconds since 1Jan1904=w3839:timestamp)
      n1572 = Format Date/Time String(time format string (%c)="%Y%m%d%H%M%S%3u" ("时间格式字符串(%c)"), seconds (now)=w3839) -> (date/time string=w3838:string)  [unwired: 1 in]
      n1573 = Search and Replace String(input string=w3838, search string="." ("搜索字符串")) -> (result string=w3836:string)  [unwired: 6 in, 3 out]
    }
    frame "3090仪器参数" {
      n1574 = global read "全局1.vi" "枚举"() -> (w3854:enum16{"返回请求应答", "上传数据", "返回执行结果"})
      n1575 = case shown="\"上传数据\"" w3854 {
        tunnel: ["9011" ("CN") "3090" ("CN") "9012" ("CN")] -> w3853
        frame "返回请求应答", Default {
        }
        frame "上传数据" {
        }
        frame "返回执行结果" {
        }
      }
      n1576 = Get Date/Time In Seconds() -> (seconds since 1Jan1904=w3851:timestamp)
      n1577 = Format Date/Time String(time format string (%c)="%Y%m%d%H%M%S%3u" ("时间格式字符串(%c)"), seconds (now)=w3851) -> (date/time string=w3850:string)  [unwired: 1 in]
      n1578 = Search and Replace String(input string=w3850, search string="." ("搜索字符串")) -> (result string=w3848:string)  [unwired: 6 in, 3 out]
    }
    frame "提取仪器参数" {
      n1579 = global read "全局1.vi" "枚举"() -> (w3862:enum16{"返回请求应答", "上传数据", "返回执行结果"})
      n1580 = case shown="\"上传数据\"" w3862 {
        tunnel: ["9011" ("CN") "3020" ("CN") "9012" ("CN")] -> w3861
        frame "返回请求应答", Default {
        }
        frame "上传数据" {
        }
        frame "返回执行结果" {
        }
      }
      n1581 = local read "QN"() -> (w3860:string)
    }
    frame "系统状态" {
      n1582 = local read "QN"() -> (w3868:string)
    }
    frame "运行模式" {
      n1583 = local read "QN"() -> (w3872:string)
    }
    frame "测量周期" {
      n1584 = local read "QN"() -> (w3876:string)
    }
    frame "超标留样" {
      n1585 = local read "QN"() -> (w3880:string)
    }
  }
  n1586 = Bundle By Name(cluster="数据块", "ST"=w46, "CN"=w50, "FLAG"=w49, "CP"=w48, "QN"=w36, "MN"="MN", "PW"="PW", "PNUM"=w40, "PNO"=w40) -> (w47:T1)
  n1587 = call "HJ212-2017.vi"("PWD？"=FALSE, "数据段"=w47) -> ("通讯包字符串"=w54:string, "通讯包"=→"通讯包":T2)  [unwired: 7 in, 1 out]
  "通讯包字符串" <- w54
  n1588 = String Length(string=w54) -> (length=→"长度":i32)
  "错误常量" <- "错误常量 2"
  "小时数据发送次数" <- 0 ("小时数据发送次数")
  "核查数据发送次数" <- 0 ("核查数据发送次数")
